vi "WVDIAL+HSRL_v4.0.vi"() -> ()   [LabVIEW 2012]
uses:
  C:/Users/H2ODial/Desktop/Shared Telescope WV DIAL Code/Libraries and VIs/PowerMeterCommands.dll
  Shared Telescope WV DIAL Code/Libraries and VIs/PowerMeterCommands.dll
  <vilib>/DAQmx/write.llb/DAQmx Write (Digital 1D Bool NChan 1Samp 1Line).vi
  <vilib>/DAQmx/miscellaneous.llb/DAQmx Fill In Error Info.vi
  <vilib>/Analysis/baseanly.llb/Mean (DBL).vi
  AMCS_Data.vi
  Libraries and VIs/Scalar_Data.vi
  <vilib>/Analysis/NI_AALBase.lvlib
  Libraries and VIs/Scalar_Data_2.vi
  Libraries and VIs/Scalar_Data_4.vi
  Libraries and VIs/Scalar_Data_3.vi
  Shared Telescope WV DIAL Code/bristol/CLDevIFace.dll
panel:
  out "FileHour":i32=20
  out "L_Count":i32=43
  out "background start":u32=534
  in  "Tab Control 2":enum32{"WV ND narrow", "WV ND wide"}(tab)=enum."WV ND wide"
  out "CH3 RingBuffer long":dbl[][](array[numeric])
  out "CH3 RingBuffer short":dbl[][](array[numeric])
  in  "?":T1(tab)=enum."Raw Counts combined"
  out "NRB":dbl[][](graph) caption="Water Vapor Number Density"
  out "NRB 2":dbl[][](graph)=[[-2.5020981634886346e-06, -3.8273570593616536e-05, -0.0001038319411503206, -0.00016406881143786204, -0.00024572601577053764, -0.00034001735639440826, -0.0003495277310288337, -0.00033797799127632697, -2.508089447238247e-05, 0.0004628603911393724, 0.0008910726426874336, 0.0014015403952404464, 0.0014313599056918725, 0.0023638962541973306, 0.00363462235094875, 0.005273167971630326, 0.007177084059402028, 0.007921603484325369, 0.010612501535131786, 0.013715391450269933, 0.01773512062835457, 0.025311202683991355, 0.029501238164518568, 0.03663684456864366, 0.042833095042680805, 0.04585338221968253, 0.05157986876646168, 0.057672169500993145, 0.06480582531005098, 0.07494068068754126, 0.08374302915097871, 0.09012600975592831, 0.0975137618371565, 0.10316252486978073, 0.10713266491787977, 0.11105920366892658, 0.11731957195587771, 0.12190536182534215, 0.13263667129454806, 0.14291236842912694, 0.15648209640166563, 0.17000563027429774, 0.1781337441537761, 0.18845836788040057, 0.18774352015967605, 0.1846468106536388, 0.18853627471102877, 0.18467849065439743, 0.19086511631707134, 0.2040589251100288, 0.207911100976431, 0.2171413823506752, 0.22141130681510074, 0.21910574498821542, 0.22451361076955265, 0.23126120500572805, 0.2339651115949773, 0.23260695324025257, 0.2442695368570803, 0.24254083915478225, 0.24350501849934109, 0.25495583092371427, 0.256919203446593, 0.2588364738795642, 0.2752215466716228, 0.2780859354051604, 0.276346005548185, 0.2745175766787534, 0.2601535580068366, 0.2676645740334584, 0.28421418272066157, 0.3206297444553061, 0.7143078116413505, 21.54115268912089, 33.95125947144662, 31.700981872059664, 41.68522002923662, 49.68783445276399, 45.33320709409449, 50.91175336548996, 41.008304913663714, 7.850979651089744, 0.6303614668230137, 0.015684134239805404, -0.10748397859242446, -0.14387707768036828, -0.16031827295901913, -0.18772557122864725, -0.18330253680007566, -0.18786123473446648, -0.19225778267096172, -0.1708619433096678, -0.18061455888020886, -0.20344725887325812, -0.21222191618851236, -0.2230615330389505, -0.22863568943154486, -0.21415229293082613, -0.19801980569945724, -0.17746233563109473, -0.17232152452285898, -0.19301319899423522, -0.1928522325449715, -0.20695955144125755, -0.2198018954874654, -0.20891051933015198, -0.2450116286469604, -0.2762364146721713, -0.25775858469018326, -0.2869767975303511, -0.31227413136513704, -0.30464323595703785, -0.3409117288411666, -0.3002103543236415, -0.23741414224173096, -0.26319432381274527, -0.23706217272299082, -0.28542556132066793, -0.3145034821484638, -0.27746295249821534, -0.2910899621994402, -0.22821160056074022, -0.2453504388340374, -0.2668569865375988, -0.302726932626319, -0.36635809732218244, -0.31647236719541494, -0.3452309484397592, -0.3275452371280285, -0.3333382932273667, -0.33548626372238755, -0.25688129406848426, -0.2467778023481867, -0.23498727603876554, -0.3129911904091031, -0.36614944944121386, -0.3533463690282559, -0.34154994204384004, -0.25165828962384623, -0.31691690943776746, -0.3245958208612461, -0.30425963660235494, -0.36843072902715324, -0.3157345000339491, -0.3275597079763837, -0.35818288327065395, -0.352364263091795, -0.33006433024904047, -0.3112468058790122, -0.23728059325129242, -0.22160963498338146, -0.22843717220060503, -0.31911234637289393, -0.43330862371719997, -0.45699042470294016, -0.4997768306732525, -0.4433418654318298, -0.44943541181506524, -0.482701240492616, -0.45281165642757787, -0.4539575719756435, -0.44359959762718015, -0.394802905964343, -0.43110696608508436, -0.4487943579107743, -0.44914927650382974, -0.4947334937868066, -0.5341525316404566, -0.45103820079960005, -0.4235942576800866, -0.42969521521255355, -0.3104652257561939, -0.3955757538174749, -0.3907148860769188, -0.3413445405384114, -0.44499503326768464, -0.4321269376895156, -0.46081506960875707, -0.4251383509343469, -0.41557002793056597, -0.40480981179417447, -0.34227620645148243, -0.2837964365676406, -0.2403409864667895, -0.31151461583845225, -0.40458731751210936, -0.4530771605846155, -0.530890834134058, -0.5174474687334719, -0.4705780895443756, -0.6251390473827461, -0.5608002128241332, -0.4805744396213767, -0.4939558392940799, -0.49893090586369987, -0.5815126113425622, -0.7539013482542295, -0.7201830577508319, -0.5974136122426202, -0.427319227255229, -0.23109328371912188, -0.37265592068247794, -0.4846088601881629, -0.5593198327797039, -0.6475257233138102, -0.6087540942922537, -0.4874376718973655, -0.47865733754219053, -0.5401916562010755, -0.596485197542672, -0.5963785290973199, -0.5983461777031588, -0.44328861700080574, -0.26085296759952376, -0.2699562750294853, -0.34464975700012546, -0.378374175405242, -0.509164782406029, -0.49723438050335145, -0.55406973131386, -0.5550984406698001, -0.43996054512749955, -0.5206803647051025, -0.4095467324146769, -0.48370538312072786, -0.5692902449808945, -0.6330050873588459, -0.8193325502186768, -0.8779549530887577, -0.816539854359666, -0.6441653120171549, -0.4727360575130327, -0.4628552538239389, -0.5620478433524031, -0.655494042494383, -0.7399613369892488, -0.6405030408770369, -0.5765708949382735, -0.4726984725137904, -0.3915113429195965, -0.3134944364340016, -0.2248912333800384, -0.36875022215993414, -0.3554536886236827, -0.5980166385656092, -0.8193537790579545, -0.7521812952169191, -0.6971205141068005, -0.6181283857949139, -0.5900935588544917, -0.7562170181152746, -0.6416065082367906, -0.7307816848017402, -0.5270352944590446, -0.300116480279226, -0.37553963593937656, -0.2941933059065934, -0.47641380968548086, -0.5378654657741927, -0.6071779010544753, -0.4686312128566513, -0.5899512920252556, -0.6862698061644342, -0.7428879117678355, -0.8761602999416397, -0.7561276317699211, -0.7202615010974514, -0.7483281485207611, -0.7482154522350888, -0.5525177903179376, -0.4488008176595967, -0.22978861391703273, -0.13150232773217932, -0.1332402387625776, -0.06078266202039725, -0.39966517834005755, -0.5783801042920869, -0.8171422439228425, -0.9551656614336947, -0.8733043067019355, -0.6959516078841153, -0.7690989054771367, -0.8652022149225229, -0.6099182034625025, -0.7679998738959176, -0.7223416094461833, -0.7570644057546929, -1.2654974200164584, -1.3779590792235303, -1.5622266280255943, -1.386936070753788, -1.2471038836252353, -1.087283687193855, -0.8721120158881883, -1.0872571189847513, -0.9849759903134073, -0.771411546098274, -0.8509297898990206, -0.9081599500982982, -0.6790337607839299, -0.9278070419202001, -0.621797181323692, -0.5821482738615157, -1.0750661807231106, -1.2314382214462831, -1.5519022989390405, -1.4796651905938325, -1.2102421860882273, -1.0282077259873421, -0.4362873109031171, -0.40559426367495305, -0.2292032463648166, -0.21857441066377944, -0.9109430342662433, -1.282550258698898, -1.3876047401862814, -1.5045893419592666, -1.4374711281318844, -1.2050621952116298, -1.0103568077270157, -0.5897468684843571, -0.29535566057607804, -0.27893832184515194, -0.6263885355424194, -0.9074170726475529, -0.9534692140938759, -0.9710631908445434, -0.760777904963038, -0.8433895851549431, -0.7917487575180413, -0.7514584846094501, -0.8766094127754804, -0.671180633107386, -0.5887340833307931, -0.6049688202388804, -0.6515728951252249, -0.7953097338321125, -0.9273888663025621, -0.6352708304436501, -0.7532266459861103, -0.953097474788277, -1.014056313184273, -1.2798394152447108, -1.2552531089492367, -1.3478709811287533, -1.4390342075966889, -1.426306262141701, -1.381381316355439, -0.9252331614157784, -0.41493739744643776, -0.3243230693658629, -0.06387449281903544, -0.18609024214117245, -0.7804262391658887, -1.0493895157641866, -1.3174091629330624, -1.3903818994181472, -1.152477696612482, -1.0616779068473232, -0.9080173908622341, -0.8545100052333319, -0.47579763315226625, -0.08556205823523852, -0.22014402145078743, -0.10890642998361617, -0.5553035660570823, -0.2958777336933946, -0.3959921627809348, -0.556970419169587, -0.4186254510131068, -0.7485884874552019, -0.19289238765646766, 0.05430929448269791, -0.35478245323789875, -1.0561668550116012, -1.1898220201473728, -1.2458813203298933, -0.815334398103235, -0.0671490954357261, -0.018451762627068893, -0.11119254378964742, -0.4427154390499537, -0.6760221931822215, -1.3461845836896529, -1.8076463186027565, -1.8385077103062597, -1.7869301307658811, -1.6232306012680962, -1.4738471688873729, -1.3087672612167474, -1.2315906623490736, -1.1135123530760682, -1.139861483958716, -1.2569515292132314, -1.4088959931515883, -1.1250574891186882, -1.001539558123051, -0.7088183927720361, -0.514128544452265, -0.3454411632455565, 0.3000404281767336, 0.1645627582469719, 0.04890717768161907, 0.08947454524138758, -0.07724098944459341, -0.058958284211915034, -0.3667306904105761, -0.9904304551610316, -1.7027285480575052, -1.306338059968992, -1.1597564928464528, -0.3530837286192967, 0.5746539364824368, 0.23334933859722826, 0.4182851174867973, -0.30059774866289063, -0.8890626237655932, -0.9472750803671779, -0.8578628063534488, -0.9533360290473383, -0.5079315412639782, -0.26717148091086973, -0.45138122167384986, -0.8642746108786942, -0.7295568974321442, -0.6794525679270975, -0.4380641006827398, 0.5769193464805378, 0.22719774605138796, -0.2983324510443344, -0.30673253473033524, -0.8094870539813328, -1.035132568856701, -0.4124781117273112, -0.2747964251818897, -0.11039052863799699, -0.5885488301511802, -0.8058036703841541, -0.4663379722359256, -0.33030440722377336, -0.467927769570105, -1.1000558593661727, -2.0467207202621625, -2.551496069836077, -2.0536979920090666, -1.3499994517878882, -1.153871773838675, -0.5889425800789698, -0.2969193437698364, -0.37189047692613214, -0.09857520941841777, -0.892482435033178, -0.3015291458282375, -0.4266194375179333, -0.1408214342371235, 0.16821762837943968, -0.40361403530403833, -0.7177182682819262, -1.0728370530752864, -1.3729370161062138, -1.357043316659708, -1.0180794658931187, -1.3953152006681284, -0.7536344811984687, -0.5284048490717401, -0.4122172561441862, -0.054807712791502865, 0.5146587876030838, 0.4753438773876348, 0.3674548243403802, -0.7042427610448878, -1.1016058965545648, -0.9988289529332682, -1.6435072651641673, -0.6465888479397265, -0.7806826027457424, -1.022038241655911, -0.230679192242146, -0.759068236712521, -0.7535460754503612, -1.7178022862235443, -1.5663725973853304, -0.7565920024141967, -1.0450226922537755, -0.5586958948537327, -0.5488466781858061, -0.5568035653235451, -1.1032149253845942, -0.8009372538073485, -0.34126394357978, -0.8844203222099551, -0.6006849348938932, -0.6731739721978937, -1.460340765246951, -1.4452465918657313, -0.26441783208271397, -0.4943103053231315, -0.14316728933687042, 0.47572218129688315, -0.40079671920864024, -0.5505246695459326, -0.7083516606019646, -0.03233006932487573, -0.512690199641294, 0.26494490817366023, -0.7759032781550804, -1.578772092440307, -0.09584587307128617, 0.45052636975528176, 0.49960481452995287, 0.13866569826607072, -1.756634496879691, -3.626331301345096, -2.473565538083194, -2.245781662386054, -1.8764305761241498, -0.45052407312514464, -0.752383991024165, -0.758988271335676, 0.176068333208736, -0.1380694180006847, -0.06847766192829471, -0.37563895911621303, -0.9959950091463621, -0.9345547358580696, -1.2513440806923193, -0.41094699891746117, -0.2097207952913438, -1.4365356108808607, -0.7837923842133756, -0.3968929772583404, -1.0140166859071411, -0.9038007040018414, -0.7252283164133516, -1.5910573858643522, -0.25161165903524585, 0.3124499929369491, -0.7977022908808816, -0.9890490078668146, -1.1747915260490664, -1.0295378767351495, 0.45640125561722844, 1.0024654779812845, 0.6740581377789816, 1.033309351341288, 0.6186635225683902, -0.30003043189290396, 0.20275337833113002, 0.49308937811843856, 0.1813997653039158, 0.22789885511426033, 0.8665664819010523, 0.24739566365173932, 0.6284997182377698, 1.6889726435607322, 0.0, 0.0, 0.0, 0.0, 0.0]] caption="Water Vapor Number Density"
  out "CH 1 (WV off) counts display":dbl[][](graph) caption="Water Vapor Number Density"
  out "CH 3 (HSRL comb) counts display":dbl[][](graph)=[[163.47999999999956, -42.52000000000044, 147.47999999999956, 56.47999999999956, 162.47999999999956, -112.52000000000044, 181.47999999999956, 69.47999999999956, 61.47999999999956, -109.52000000000044, 99.47999999999956, 24.479999999999563, 29.479999999999563, -9.520000000000437, 82.47999999999956, 93.47999999999956, 110.47999999999956, -50.52000000000044, 22.479999999999563, -20.520000000000437, -58.52000000000044, 64.47999999999956, 110.47999999999956, 140.47999999999956, 300.47999999999956, 243.47999999999956, 153.47999999999956, 253.47999999999956, 165.47999999999956, 274.47999999999956, 247.47999999999956, 380.47999999999956, 156.47999999999956, 346.47999999999956, 248.47999999999956, 285.47999999999956, 327.47999999999956, 353.47999999999956, 258.47999999999956, 140.47999999999956, 243.47999999999956, 243.47999999999956, 229.47999999999956, 238.47999999999956, 279.47999999999956, 188.47999999999956, 327.47999999999956, 293.47999999999956, 292.47999999999956, 291.47999999999956, 196.47999999999956, 333.47999999999956, 129.47999999999956, 72.47999999999956, 119.47999999999956, 267.47999999999956, 205.47999999999956, 135.47999999999956, 305.47999999999956, 111.47999999999956, 145.47999999999956, 190.47999999999956, 271.47999999999956, 144.47999999999956, 133.47999999999956, 230.47999999999956, 162.47999999999956, 201.47999999999956, 195.47999999999956, 277.47999999999956, 258.47999999999956, 80.47999999999956, 44.47999999999956, 160.47999999999956, 347.47999999999956, 882.4799999999996, 31366.48, 56924.479999999996, -5504.52, 57991.479999999996, 42322.479999999996, 13697.48, 1435.4799999999996, 48.47999999999956, -40.52000000000044, -63.52000000000044, 22.479999999999563, -217.52000000000044, 91.47999999999956, -239.52000000000044, -60.52000000000044, -95.52000000000044, 6.479999999999563, -24.520000000000437, -143.52000000000044, -131.52000000000044, 25.479999999999563, -192.52000000000044, 31.479999999999563, -141.52000000000044, 71.47999999999956, -31.520000000000437, -63.52000000000044, -57.52000000000044, -23.520000000000437, -109.52000000000044, -10.520000000000437, 4.479999999999563, -42.52000000000044, -61.52000000000044, -92.52000000000044, -39.52000000000044, -46.52000000000044, 124.47999999999956, -113.52000000000044, 28.479999999999563, 55.47999999999956, -83.52000000000044, -197.52000000000044, 48.47999999999956, -50.52000000000044, -60.52000000000044, -104.52000000000044, -64.52000000000044, -26.520000000000437, -72.52000000000044, 34.47999999999956, 85.47999999999956, -56.52000000000044, -177.52000000000044, -104.52000000000044, -89.52000000000044, -140.52000000000044, -46.52000000000044, 0.47999999999956344, -11.520000000000437, -73.52000000000044, 29.479999999999563, -94.52000000000044, -59.52000000000044, -53.52000000000044, 38.47999999999956, -137.52000000000044, 57.47999999999956, 3.4799999999995634, -143.52000000000044, -10.520000000000437, 69.47999999999956, -167.52000000000044, -3.5200000000004366, 62.47999999999956, 6.479999999999563, 5.479999999999563, -83.52000000000044, -31.520000000000437, -159.52000000000044, -85.52000000000044, -72.52000000000044, -163.52000000000044, -137.52000000000044, -108.52000000000044, -30.520000000000437, 86.47999999999956, -37.52000000000044, 50.47999999999956, -66.52000000000044, 115.47999999999956, 45.47999999999956, 150.47999999999956, -129.52000000000044, -45.52000000000044, 28.479999999999563, -82.52000000000044, -160.52000000000044, -107.52000000000044, 59.47999999999956, -273.52000000000044, -3.5200000000004366, -25.520000000000437, -28.520000000000437, -9.520000000000437, -21.520000000000437, -111.52000000000044, 3.4799999999995634, -113.52000000000044, -100.52000000000044, 5.479999999999563, -9.520000000000437, 19.479999999999563, 59.47999999999956, -135.52000000000044, 83.47999999999956, 0.47999999999956344, -2.5200000000004366, -197.52000000000044, -24.520000000000437, 15.479999999999563, 2.4799999999995634, -176.52000000000044, -151.52000000000044, 113.47999999999956, 0.47999999999956344, 49.47999999999956, 115.47999999999956, -214.52000000000044, -17.520000000000437, 15.479999999999563, -41.52000000000044, 43.47999999999956, -36.52000000000044, -52.52000000000044, -157.52000000000044, -244.52000000000044, -63.52000000000044, 72.47999999999956, 90.47999999999956, 43.47999999999956, -9.520000000000437, 20.479999999999563, 145.47999999999956, -57.52000000000044, -139.52000000000044, 59.47999999999956, 51.47999999999956, -102.52000000000044, -199.52000000000044, -21.520000000000437, 111.47999999999956, -76.52000000000044, 54.47999999999956, -28.520000000000437, 8.479999999999563, 32.47999999999956, -121.52000000000044, -142.52000000000044, -106.52000000000044, 21.479999999999563, -22.520000000000437, 44.47999999999956, 43.47999999999956, -155.52000000000044, 64.47999999999956, 140.47999999999956, -107.52000000000044, -2.5200000000004366, 71.47999999999956, -17.520000000000437, -33.52000000000044, -85.52000000000044, 121.47999999999956, -191.52000000000044, 114.47999999999956, 2.4799999999995634, 24.479999999999563, 143.47999999999956, -107.52000000000044, 107.47999999999956, -2.5200000000004366, 31.479999999999563, -55.52000000000044, -102.52000000000044, -0.5200000000004366, -93.52000000000044, -209.52000000000044, 110.47999999999956, -50.52000000000044, 36.47999999999956, -52.52000000000044, 88.47999999999956, 22.479999999999563, -84.52000000000044, 52.47999999999956, 105.47999999999956, -94.52000000000044, 3.4799999999995634, -114.52000000000044, 108.47999999999956, -101.52000000000044, -3.5200000000004366, 86.47999999999956, -96.52000000000044, -42.52000000000044, -116.52000000000044, 90.47999999999956, 47.47999999999956, -26.520000000000437, -97.52000000000044, -161.52000000000044, 34.47999999999956, -30.520000000000437, 54.47999999999956, -117.52000000000044, -85.52000000000044, 46.47999999999956, 69.47999999999956, -1.5200000000004366, 135.47999999999956, 49.47999999999956, 4.479999999999563, 71.47999999999956, -11.520000000000437, -89.52000000000044, 83.47999999999956, -77.52000000000044, -74.52000000000044, -125.52000000000044, -176.52000000000044, -90.52000000000044, -0.5200000000004366, -148.52000000000044, 26.479999999999563, -34.52000000000044, -106.52000000000044, 97.47999999999956, 62.47999999999956, -68.52000000000044, 103.47999999999956, 68.47999999999956, 44.47999999999956, -1.5200000000004366, -112.52000000000044, 8.479999999999563, -159.52000000000044, 34.47999999999956, 34.47999999999956, -59.52000000000044, -89.52000000000044, -55.52000000000044, -82.52000000000044, 1.4799999999995634, -21.520000000000437, 13.479999999999563, 65.47999999999956, 154.47999999999956, -1.5200000000004366, -56.52000000000044, -3.5200000000004366, 89.47999999999956, 26.479999999999563, -15.520000000000437, 14.479999999999563, -28.520000000000437, -17.520000000000437, 38.47999999999956, -207.52000000000044, 30.479999999999563, -2.5200000000004366, 19.479999999999563, -59.52000000000044, 17.479999999999563, 3.4799999999995634, -23.520000000000437, 9.479999999999563, 178.47999999999956, 111.47999999999956, -89.52000000000044, -157.52000000000044, -84.52000000000044, -6.520000000000437, 80.47999999999956, 139.47999999999956, 15.479999999999563, -79.52000000000044, -157.52000000000044, 117.47999999999956, 12.479999999999563, -65.52000000000044, -15.520000000000437, -123.52000000000044, -44.52000000000044, 34.47999999999956, 2.4799999999995634, -118.52000000000044, -15.520000000000437, 34.47999999999956, 4.479999999999563, -17.520000000000437, -46.52000000000044, 103.47999999999956, 33.47999999999956, -6.520000000000437, 5.479999999999563, 94.47999999999956, -185.52000000000044, -14.520000000000437, -142.52000000000044, -40.52000000000044, -82.52000000000044, -8.520000000000437, -96.52000000000044, -58.52000000000044, -18.520000000000437, 35.47999999999956, 42.47999999999956, -8.520000000000437, 102.47999999999956, 159.47999999999956, 29.479999999999563, 131.47999999999956, 20.479999999999563, -62.52000000000044, -42.52000000000044, 99.47999999999956, 48.47999999999956, -1.5200000000004366, 35.47999999999956, -32.52000000000044, 128.47999999999956, -8.520000000000437, -83.52000000000044, 55.47999999999956, -1.5200000000004366, -92.52000000000044, 58.47999999999956, 23.479999999999563, 101.47999999999956, 63.47999999999956, -2.5200000000004366, 151.47999999999956, 6.479999999999563, 47.47999999999956, 44.47999999999956, -96.52000000000044, 79.47999999999956, -147.52000000000044, 25.479999999999563, -124.52000000000044, 77.47999999999956, 63.47999999999956, -5.520000000000437, 27.479999999999563, -142.52000000000044, -36.52000000000044, -58.52000000000044, -98.52000000000044, -83.52000000000044, 21.479999999999563, -7.520000000000437, -51.52000000000044, -123.52000000000044, 5.479999999999563, 69.47999999999956, -55.52000000000044, -79.52000000000044, 68.47999999999956, -40.52000000000044, -54.52000000000044, 28.479999999999563, -50.52000000000044, 64.47999999999956, -87.52000000000044, 104.47999999999956, 48.47999999999956, 44.47999999999956, -165.52000000000044, 87.47999999999956, -116.52000000000044, 5.479999999999563, -68.52000000000044, 44.47999999999956, 180.47999999999956, 175.47999999999956, 117.47999999999956, -28.520000000000437, 74.47999999999956, 83.47999999999956, 95.47999999999956, 121.47999999999956, 67.47999999999956, 15.479999999999563, 74.47999999999956, -1.5200000000004366, 2.4799999999995634, -21.520000000000437, -232.52000000000044, 83.47999999999956, -96.52000000000044, 8.479999999999563, -115.52000000000044, -87.52000000000044, 4.479999999999563, 20.479999999999563, 67.47999999999956, -180.52000000000044, 8.479999999999563, -62.52000000000044, -75.52000000000044, -18.520000000000437, -116.52000000000044, 61.47999999999956, -23.520000000000437, 79.47999999999956, 112.47999999999956, -79.52000000000044, -41.52000000000044, -162.52000000000044, 22.479999999999563, -24.520000000000437, -2.5200000000004366, -26.520000000000437, 71.47999999999956, 4.479999999999563, 4.479999999999563, -99.52000000000044, 84.47999999999956, -61.52000000000044, 33.47999999999956, -67.52000000000044, -71.52000000000044, 43.47999999999956, -15.520000000000437, -79.52000000000044, -63.52000000000044, -3.5200000000004366, -43.52000000000044, -105.52000000000044, -6.520000000000437, -38.52000000000044, -38.52000000000044, 16.479999999999563, 129.47999999999956, -28.520000000000437, 16.479999999999563, -50.52000000000044, 132.47999999999956, -76.52000000000044, 34.47999999999956, 47.47999999999956, -135.52000000000044, -27.520000000000437, 43.47999999999956, -111.52000000000044, 79.47999999999956, 74.47999999999956, -33.52000000000044, -53.52000000000044, 28.479999999999563, -17.520000000000437, 83.47999999999956, -30.520000000000437, -17.520000000000437, 13.479999999999563, 10.479999999999563, -45.52000000000044, 54.47999999999956, 165.47999999999956, -3.5200000000004366, -40.52000000000044, -41.52000000000044, -2.5200000000004366, -18.520000000000437, 44.47999999999956, -45.52000000000044, -103.52000000000044, 84.47999999999956, -46.52000000000044, 1.4799999999995634, 16.479999999999563, -2.5200000000004366, 0.0]] caption="Water Vapor Number Density"
  out "CH3 (HSRL combined) smooth S":dbl[](array[numeric])=[-5.880967741935467, -22.493870967741916, -27.122903225806432, -24.10677419354837, -23.10677419354837, -22.203548387096756, -16.768064516129016, -12.413225806451594, -0.7277419354838548, 10.877096774193564, 17.304516129032276, 22.869032258064532, 19.901290322580664, 28.336774193548404, 37.949677419354856, 48.3851612903226, 58.328709677419376, 57.42548387096776, 69.03838709677422, 80.51419354838711, 94.41741935483871, 122.74000000000001, 130.87709677419355, 149.24, 160.7803225806452, 159.1351612903226, 165.98193548387098, 172.55451612903227, 180.74, 195.27225806451614, 204.33677419354842, 206.37709677419357, 209.95774193548388, 209.24806451612903, 205.07064516129034, 200.94967741935486, 200.95774193548388, 197.97387096774196, 204.48193548387098, 209.43354838709678, 218.24806451612906, 225.9335483870968, 225.85290322580647, 228.19967741935488, 217.36903225806455, 204.61903225806455, 200.14322580645162, 187.99, 186.44161290322583, 191.42548387096775, 187.47387096774196, 188.3367741935484, 184.86903225806452, 176.24806451612903, 174.09483870967745, 172.98193548387098, 168.92548387096775, 162.21580645161293, 164.61903225806452, 158.06258064516132, 153.53838709677422, 155.6109677419355, 151.87709677419355, 148.27225806451617, 152.8367741935484, 149.78838709677422, 144.44967741935486, 139.3125806451613, 128.24, 128.19967741935486, 132.3125806451613, 145.12709677419355, 313.9254838709678, 8378.159354838708, 12241.586774193547, 11271.489999999998, 13944.506129032256, 15799.47387096774, 14332.546451612903, 15460.320645161291, 12615.24806451613, 2662.3851612903227, 214.5383870967742, 5.22387096774195, -34.977741935483856, -45.74387096774191, -49.808387096774176, -57.009999999999984, -54.42129032258063, -54.54225806451611, -54.598709677419336, -47.469677419354824, -49.106774193548375, -54.147096774193535, -55.300322580645144, -56.92129032258063, -57.14709677419353, -52.437419354838696, -47.50999999999999, -41.72774193548386, -39.719677419354824, -43.62290322580643, -42.74387096774192, -44.99387096774192, -46.880967741935464, -43.719677419354824, -50.32451612903225, -55.69548387096773, -51.018064516129016, -55.77612903225805, -59.606774193548375, -57.1148387096774, -62.79225806451611, -54.32451612903224, -42.211612903225785, -45.99387096774191, -40.719677419354824, -48.20354838709676, -52.227741935483856, -45.308387096774176, -46.75193548387095, -36.050322580645144, -38.130967741935464, -40.808387096774176, -45.558387096774176, -54.268064516129016, -46.139032258064496, -49.550322580645144, -46.28419354838709, -46.380967741935464, -45.96967741935482, -34.66322580645159, -32.800322580645144, -30.768064516129016, -40.380967741935464, -46.550322580645144, -44.268064516129016, -42.171290322580624, -30.622903225806432, -38.018064516129016, -38.389032258064496, -35.47774193548385, -42.3648387096774, -35.800322580645144, -36.63096774193547, -39.509999999999984, -38.34064516129031, -35.42935483870966, -32.96161290322579, -24.792258064516115, -22.848709677419336, -23.24387096774192, -32.050322580645144, -42.96161290322579, -44.727741935483856, -48.29225806451611, -42.29225806451611, -42.33258064516127, -44.89709677419353, -41.590645161290304, -41.179354838709656, -39.74387096774192, -34.937419354838696, -37.687419354838696, -38.759999999999984, -38.32451612903223, -41.711612903225785, -44.50193548387095, -37.130967741935464, -34.46161290322579, -34.550322580645144, -24.671290322580628, -31.07451612903224, -30.340645161290304, -26.20354838709676, -33.77612903225805, -32.42935483870966, -34.19548387096772, -31.195483870967728, -30.155161290322567, -29.050322580645144, -24.292258064516112, -19.921290322580628, -16.687419354838696, -21.397096774193532, -27.49387096774192, -30.46161290322579, -35.31645161290321, -34.058387096774176, -30.647096774193535, -40.29225806451611, -35.768064516129016, -30.332580645161272, -30.856774193548368, -30.848709677419336, -35.590645161290304, -45.679354838709656, -43.19548387096772, -35.469677419354824, -25.114838709677404, -13.445483870967724, -21.469677419354824, -27.647096774193532, -31.59870967741934, -36.227741935483856, -33.727741935483856, -26.74387096774192, -26.009999999999984, -29.07451612903224, -31.800322580645144, -31.49387096774192, -31.300322580645147, -22.969677419354824, -13.3890322580645, -13.727741935483854, -17.364838709677404, -18.8890322580645, -25.187419354838696, -24.372903225806436, -26.913225806451596, -26.71967741935482, -20.985806451612888, -24.614838709677404, -19.187419354838692, -22.46161290322579, -26.20354838709676, -28.88096774193547, -37.05838709677418, -39.3648387096774, -36.29225806451612, -28.380967741935468, -20.647096774193532, -20.042258064516112, -24.130967741935468, -27.905161290322564, -31.235806451612888, -26.808387096774176, -23.929354838709664, -19.453548387096756, -15.977741935483856, -12.687419354838694, -9.026129032258048, -14.679354838709662, -14.03419354838708, -23.421290322580628, -31.832580645161276, -28.985806451612888, -26.647096774193535, -23.437419354838696, -22.195483870967728, -28.219677419354824, -23.75193548387095, -26.840645161290304, -19.20354838709676, -10.848709677419336, -13.46967741935482, -10.469677419354822, -16.82451612903224, -18.848709677419336, -21.1148387096774, -16.171290322580628, -20.20354838709676, -23.32451612903224, -25.058387096774176, -29.332580645161272, -25.122903225806432, -23.751935483870948, -24.49387096774192, -24.30838709677418, -17.816451612903208, -14.364838709677404, -7.300322580645146, -4.147096774193532, -4.171290322580629, -1.8890322580644998, -12.332580645161274, -17.719677419354824, -24.856774193548368, -28.848709677419333, -26.187419354838692, -20.719677419354824, -22.735806451612888, -25.397096774193532, -17.776129032258048, -22.227741935483856, -20.759999999999984, -21.606774193548368, -35.87290322580644, -38.79225806451611, -43.67935483870966, -38.509999999999984, -34.3890322580645, -29.776129032258048, -23.719677419354824, -29.372903225806436, -26.429354838709664, -20.558387096774176, -22.526129032258048, -23.880967741935468, -17.735806451612888, -24.074516129032244, -16.026129032258048, -14.905161290322564, -27.34870967741934, -31.122903225806436, -38.969677419354824, -36.91322580645159, -29.99387096774192, -25.316451612903208, -10.671290322580628, -9.856774193548372, -5.53419354838708, -5.24387096774192, -21.719677419354824, -30.389032258064503, -32.67129032258063, -35.20354838709676, -33.42129032258063, -27.840645161290308, -23.195483870967728, -13.453548387096758, -6.695483870967726, -6.284193548387081, -14.026129032258048, -20.195483870967728, -21.090645161290308, -21.34870967741934, -16.622903225806436, -18.316451612903208, -17.090645161290308, -16.122903225806436, -18.695483870967728, -14.227741935483854, -12.405161290322564, -12.671290322580628, -13.566451612903208, -16.46161290322579, -19.082580645161276, -12.993870967741918, -15.31645161290321, -19.268064516129016, -20.380967741935468, -25.574516129032244, -24.937419354838692, -26.622903225806436, -28.259999999999984, -27.84870967741934, -26.81645161290321, -17.85677419354837, -7.96161290322579, -6.187419354838694, -1.2116129032257903, -3.509999999999984, -14.6390322580645, -19.57451612903224, -24.437419354838692, -25.64709677419353, -21.139032258064496, -19.364838709677404, -16.469677419354824, -15.413225806451596, -8.534193548387082, -1.5261290322580485, -3.9051612903225643, -1.9212903225806286, -9.74387096774192, -5.163225806451596, -6.872903225806435, -9.614838709677404, -7.187419354838693, -12.78419354838708, -3.2761290322580474, 0.9174193548387262, -5.96161290322579, -17.655161290322564, -19.78419354838708, -20.60677419354837, -13.413225806451596, -1.0987096774193386, -0.30032258064514505, -1.800322580645145, -7.130967741935468, -10.832580645161274, -21.46161290322579, -28.67129032258063, -29.009999999999984, -28.050322580645144, -25.34870967741934, -22.897096774193532, -20.227741935483852, -18.937419354838696, -17.03419354838708, -17.348709677419336, -19.03419354838708, -21.227741935483856, -16.864838709677404, -14.937419354838694, -10.518064516129016, -7.590645161290306, -5.074516129032242, 4.385161290322596, 2.393225806451629, 0.7077419354838868, 1.2883870967742097, -1.106774193548371, -0.8406451612903063, -5.203548387096758, -13.985806451612886, -23.92935483870966, -18.268064516129016, -16.1390322580645, -4.8890322580645, 7.917419354838726, 3.199677419354855, 5.707741935483886, -4.082580645161274, -12.018064516129016, -12.74387096774192, -11.485806451612888, -12.703548387096758, -6.735806451612888, -3.526129032258048, -5.929354838709662, -11.300322580645144, -9.49387096774192, -8.800322580645144, -5.647096774193531, 7.401290322580662, 2.901290322580661, -3.7922580645161132, -3.880967741935468, -10.195483870967726, -12.977741935483856, -5.147096774193532, -3.413225806451597, -1.364838709677403, -7.24387096774192, -9.872903225806436, -5.687419354838695, -4.009999999999985, -5.655161290322565, -13.235806451612888, -24.518064516129016, -30.42935483870966, -24.380967741935468, -15.953548387096758, -13.574516129032244, -6.897096774193531, -3.46161290322579, -4.31645161290321, -1.1390322580644998, -10.268064516129016, -3.453548387096758, -4.864838709677404, -1.5987096774193392, 1.9012903225806612, -4.542258064516112, -8.042258064516112, -11.969677419354822, -15.251935483870952, -15.009999999999982, -11.21161290322579, -15.300322580645144, -8.227741935483856, -5.743870967741919, -4.46161290322579, -0.5906451612903062, 5.522258064516146, 5.078709677419371, 3.9093548387096946, -7.46161290322579, -11.622903225806436, -10.49387096774192, -17.195483870967728, -6.735806451612886, -8.098709677419338, -10.558387096774178, -2.3729032258064353, -7.776129032258048, -7.687419354838693, -17.45354838709676, -15.848709677419338, -7.622903225806435, -10.485806451612888, -5.582580645161274, -5.46161290322579, -5.518064516129016, -10.8890322580645, -7.872903225806435, -3.340645161290305, -8.622903225806436, -5.832580645161275, -6.509999999999985, -14.06645161290321, -13.864838709677404, -2.526129032258048, -4.703548387096758, -1.3567741935483704, 4.490000000000016, -3.768064516129016, -5.155161290322565, -6.606774193548371, -0.30032258064514394, -4.743870967741919, 2.441612903225823, -7.122903225806435, -14.437419354838692, -0.8729032258064358, 4.086774193548404, 4.514193548387114, 1.2480645161290491, -15.751935483870952, -32.397096774193535, -22.009999999999984, -19.905161290322564, -16.566451612903208, -3.9616129032257894, -6.590645161290306, -6.622903225806435, 1.5303225806451777, -1.1954838709677256, -0.5906451612903062, -3.2277419354838544, -8.526129032258048, -7.969677419354823, -10.630967741935468, -3.477741935483855, -1.7680645161290158, -12.066451612903208, -6.558387096774176, -3.3083870967741777, -8.421290322580628, -7.477741935483854, -5.977741935483854, -13.06645161290321, -2.0583870967741773, 2.5464516129032413, -6.477741935483854, -8.001935483870952, -9.469677419354822, -8.268064516129016, 3.651290322580661, 7.990000000000016, 5.352903225806468, 8.175483870967758, 4.877096774193565, -2.35677419354837, 1.586774193548404, 3.8448387096774366, 1.4093548387096946, 1.7641935483871132, 6.683548387096791, 1.9012903225806612, 4.812580645161307, 12.885161290322596]
  out "CH3 (HSRL combined) smooth L":dbl[](array[numeric])=[-17.463260869565204, -33.82195652173912, -32.468695652173906, -29.849130434782598, -27.300217391304336, -24.00673913043477, -20.300217391304336, -15.452391304347815, -3.789347826086945, 3.134565217391315, 8.21608695652175, 15.313913043478271, 17.096521739130445, 24.406304347826097, 37.22695652173914, 50.313913043478266, 59.91717391304349, 63.75413043478262, 72.37369565217392, 80.30847826086958, 89.92260869565219, 112.75413043478261, 125.13456521739131, 139.44434782608698, 152.9389130434783, 154.23782608695655, 163.46608695652174, 170.97695652173914, 180.7541304347826, 194.03130434782605, 194.91173913043477, 203.4008695652174, 201.88456521739133, 200.015, 202.22152173913045, 197.3519565217391, 198.8247826086956, 198.87913043478258, 204.13456521739133, 205.3030434782609, 210.59652173913045, 216.87369565217395, 213.50956521739135, 213.9389130434783, 207.96065217391305, 196.74869565217392, 191.24869565217392, 185.69434782608695, 182.81934782608695, 188.68347826086958, 187.17260869565217, 189.5041304347826, 186.8247826086956, 174.515, 171.55304347826086, 164.6726086956522, 160.5258695652174, 155.08565217391305, 159.10739130434783, 153.4008695652174, 150.3954347826087, 151.98782608695655, 149.48239130434786, 145.79217391304348, 144.72695652173914, 142.58021739130436, 132.5095652173913, 132.23782608695655, 124.54217391304348, 125.18891304347827, 128.18891304347827, 136.4389130434783, 302.9117391304348, 7948.79760869565, 12767.781304347824, 12528.460652173913, 15319.455217391303, 17737.069347826087, 15606.493260869567, 16072.585652173913, 13111.77586956522, 3011.84652173913, 276.5204347826086, -5.528478260869555, -48.359999999999985, -57.838260869565204, -55.430652173913025, -57.90347826086955, -52.80565217391303, -51.39804347826086, -56.0936956521739, -50.89804347826086, -50.62086956521738, -53.968695652173906, -56.54478260869564, -55.3545652173913, -55.37630434782608, -51.75130434782608, -49.76217391304347, -47.65891304347825, -48.2186956521739, -51.838260869565204, -49.446956521739125, -52.64804347826086, -50.53934782608694, -48.13717391304347, -51.98499999999999, -55.86543478260869, -56.13717391304347, -57.14260869565217, -60.05021739130434, -57.061086956521734, -60.05021739130433, -53.92521739130434, -44.631739130434774, -47.63717391304347, -43.81652173913043, -52.69152173913042, -58.506739130434774, -54.31108695652173, -53.88717391304347, -42.300217391304336, -38.69695652173912, -36.62630434782608, -41.050217391304336, -51.78391304347825, -47.57739130434781, -53.963260869565204, -52.15347826086956, -50.78391304347825, -48.38717391304347, -39.40891304347825, -36.8491304347826, -35.91978260869564, -44.04478260869564, -43.90891304347825, -41.66978260869564, -39.19152173913042, -32.94152173913042, -38.15891304347825, -43.70239130434781, -42.13717391304347, -47.653478260869555, -48.80021739130434, -45.68065217391303, -46.278478260869555, -47.506739130434774, -42.62630434782608, -39.903478260869555, -33.44152173913042, -29.876304347826075, -32.28391304347825, -39.00673913043477, -48.7078260869565, -49.609999999999985, -47.56652173913042, -43.91434782608694, -41.77847826086955, -43.300217391304336, -41.017608695652164, -38.52847826086955, -42.25673913043477, -34.892608695652164, -39.28391304347825, -38.11543478260868, -30.74586956521738, -37.78391304347825, -39.66978260869564, -39.349130434782595, -41.696956521739125, -38.963260869565204, -32.0936956521739, -36.414347826086946, -36.52304347826086, -34.82195652173912, -39.506739130434774, -34.446956521739125, -30.963260869565207, -27.88173913043477, -24.648043478260856, -22.648043478260856, -19.2186956521739, -15.751304347826075, -19.376304347826075, -24.713260869565204, -32.44695652173912, -36.31652173913042, -38.31652173913042, -39.45239130434781, -41.89260869565216, -50.33282608695651, -46.54478260869564, -43.582826086956516, -38.55565217391303, -37.39804347826086, -39.65891304347825, -45.53391304347825, -41.49043478260869, -37.55021739130433, -29.87086956521738, -22.39804347826086, -30.69695652173912, -34.94695652173912, -40.968695652173906, -46.131739130434774, -44.164347826086946, -35.31108695652173, -30.767608695652164, -27.44695652173912, -31.175217391304336, -33.3491304347826, -31.816521739130422, -28.33282608695651, -16.54478260869564, -15.354565217391293, -17.403478260869555, -18.51217391304347, -25.115434782608684, -22.53391304347825, -28.175217391304336, -27.946956521739118, -27.055652173913035, -30.273043478260856, -22.936086956521727, -24.36543478260868, -23.061086956521727, -26.54478260869564, -33.82739130434781, -38.93608695652173, -37.245869565217376, -32.10456521739129, -26.436086956521727, -22.23499999999999, -27.24586956521738, -27.838260869565204, -32.56108695652173, -27.452391304347813, -21.811086956521727, -22.006739130434774, -17.202391304347813, -16.15347826086955, -14.816521739130424, -18.267608695652164, -18.555652173913032, -24.707826086956512, -27.490434782608684, -26.04478260869564, -26.131739130434774, -24.29478260869564, -27.974130434782598, -30.60456521739129, -28.941521739130422, -37.218695652173906, -31.202391304347817, -24.50130434782608, -20.403478260869555, -11.425217391304336, -14.57195652173912, -16.055652173913032, -17.865434782608684, -16.490434782608684, -24.555652173913032, -29.077391304347813, -32.01217391304347, -33.1045652173913, -28.620869565217383, -22.099130434782598, -25.436086956521727, -26.876304347826075, -16.54478260869564, -15.267608695652163, -8.381739130434772, -4.452391304347815, -5.805652173913032, -7.33282608695651, -11.446956521739118, -17.153478260869555, -24.126304347826075, -26.555652173913032, -25.04478260869564, -20.91978260869564, -21.403478260869555, -23.76217391304347, -21.686086956521727, -24.45239130434782, -20.392608695652164, -15.914347826086946, -22.25130434782608, -22.186086956521727, -28.25673913043477, -27.83282608695651, -30.680652173913032, -30.25130434782608, -25.18608695652173, -30.29478260869564, -26.29478260869564, -22.164347826086942, -25.370869565217383, -25.7186956521739, -19.191521739130422, -25.50130434782608, -20.229565217391293, -22.52304347826086, -30.724130434782598, -32.13717391304347, -37.53391304347825, -33.914347826086946, -30.533913043478254, -27.789347826086946, -16.04478260869564, -12.148043478260858, -8.740434782608684, -6.506739130434771, -20.702391304347813, -25.832826086956512, -32.45239130434781, -33.35999999999999, -30.2241304347826, -26.300217391304336, -17.794782608695638, -11.64804347826086, -8.501304347826075, -12.827391304347815, -17.930652173913032, -17.816521739130422, -16.79478260869564, -18.12630434782608, -15.327391304347817, -22.16978260869564, -20.088260869565204, -17.566521739130422, -17.751304347826075, -11.778478260869553, -9.838260869565207, -9.82195652173912, -11.186086956521729, -16.838260869565204, -21.97956521739129, -20.41978260869564, -21.963260869565207, -25.52304347826086, -22.930652173913032, -24.582826086956512, -25.00130434782608, -24.664347826086946, -29.137173913043465, -26.767608695652164, -26.501304347826075, -17.56108695652173, -9.039347826086946, -9.544782608695641, -5.773043478260859, -6.7676086956521635, -13.224130434782598, -15.332826086956512, -19.365434782608688, -20.653478260869555, -20.300217391304336, -19.202391304347813, -16.191521739130422, -19.300217391304336, -12.789347826086946, -6.6589130434782495, -7.267608695652163, -5.044782608695641, -10.849130434782598, -13.251304347826077, -13.69695652173912, -14.838260869565206, -15.474130434782598, -17.012173913043465, -11.571956521739118, -9.32195652173912, -12.164347826086946, -20.41978260869564, -21.561086956521727, -18.158913043478247, -14.968695652173903, -2.838260869565206, -4.33282608695651, -9.137173913043467, -9.115434782608684, -14.169782608695641, -17.903478260869555, -19.724130434782598, -22.061086956521727, -22.446956521739118, -30.338260869565204, -32.39260869565216, -29.865434782608684, -27.941521739130422, -21.45782608695651, -20.343695652173903, -20.63717391304347, -20.202391304347813, -15.267608695652163, -12.729565217391293, -10.436086956521729, -8.430652173913032, -6.914347826086946, -1.4360869565217278, -1.5882608695652063, -6.153478260869554, -2.811086956521728, -4.392608695652163, -3.6263043478260757, -2.7349999999999888, -8.305652173913032, -16.175217391304336, -16.925217391304336, -13.843695652173903, -9.403478260869555, 2.3030434782608804, 3.7486956521739234, 3.955217391304359, 0.6889130434782718, -5.713260869565206, -5.501304347826075, -5.224130434782597, -8.811086956521727, -5.278478260869554, -4.484999999999989, -4.3002173913043364, -6.70782608695651, -5.718695652173902, -6.490434782608684, -9.278478260869553, -2.887173913043467, -5.403478260869553, -7.528478260869554, -2.7132608695652065, -7.7676086956521635, -5.876304347826076, -3.07195652173912, -0.46326086956520607, 2.8736956521739243, -7.528478260869555, -7.2132608695652065, -7.316521739130426, -5.914347826086947, -0.9034782608695533, -8.00673913043477, -15.756739130434772, -23.104565217391293, -24.349130434782598, -16.066521739130422, -17.740434782608684, -11.120869565217381, -8.213260869565207, -11.680652173913032, -3.5339130434782504, -7.050217391304337, 3.4823913043478365, 4.172608695652185, 4.188913043478271, 3.558478260869575, -7.245869565217381, -13.811086956521729, -20.441521739130426, -25.64804347826086, -20.289347826086946, -13.137173913043467, -9.533913043478249, 0.23239130434783695, -1.8708695652173803, -2.648043478260859, -4.506739130434772, -3.4306521739130322, -5.990434782608684, -6.37086956521738, -10.881739130434772, -13.952391304347817, -13.245869565217381, -17.066521739130426, -12.974130434782596, -9.941521739130424, -10.544782608695643, -5.87086956521738, -10.066521739130424, -13.267608695652163, -16.180652173913032, -14.756739130434772, -7.365434782608684, -9.577391304347815, -6.599130434782597, -9.653478260869553, -9.91978260869564, -11.02304347826086, -10.425217391304336, -4.555652173913033, -7.006739130434772, -5.756739130434772, -9.300217391304336, -14.566521739130426, -14.245869565217383, -5.767608695652164, -4.778478260869553, -2.5502173913043364, 2.531304347826098, -1.2513043478260757, -3.0665217391304234, -4.251304347826076, -2.3708695652173803, -7.615434782608684, 2.498695652173924, -2.5121739130434673, -7.501304347826076, 3.5530434782608804, 3.471521739130446, 1.5747826086956636, -2.4415217391304225, -16.00673913043477, -29.577391304347817, -20.707826086956512, -19.365434782608684, -16.571956521739118, -5.49586956521738, -10.164347826086946, -8.58282608695651, -0.7947826086956407, -2.631739130434771, 1.8302173913043591, 0.645434782608707, -5.305652173913032, -7.414347826086946, -10.061086956521729, -7.131739130434771, -7.859999999999989, -11.919782608695641, -4.686086956521727, 1.438913043478272, 1.4497826086956644, 0.7269565217391429, -1.1534782608695542, -10.088260869565206, -2.202391304347816, 3.2486956521739234, -6.555652173913033, -5.8002173913043364, -9.550217391304336, -8.077391304347813, 2.7486956521739243, 6.868260869565229, 4.3791304347826205, 4.705217391304359, 0.24326086956522852, -6.778478260869553, 0.645434782608707, -0.2839130434782496, 1.036739130434794, 5.536739130434794, 5.265000000000011, 5.00413043478262, 6.025869565217403, 7.922608695652185]
  out "CH3 Bin Readings":dbl[](array[numeric])=[7358.0, 7152.0, 7342.0, 7251.0, 7357.0, 7082.0, 7376.0, 7264.0, 7256.0, 7085.0, 7294.0, 7219.0, 7224.0, 7185.0, 7277.0, 7288.0, 7305.0, 7144.0, 7217.0, 7174.0, 7136.0, 7259.0, 7305.0, 7335.0, 7495.0, 7438.0, 7348.0, 7448.0, 7360.0, 7469.0, 7442.0, 7575.0, 7351.0, 7541.0, 7443.0, 7480.0, 7522.0, 7548.0, 7453.0, 7335.0, 7438.0, 7438.0, 7424.0, 7433.0, 7474.0, 7383.0, 7522.0, 7488.0, 7487.0, 7486.0, 7391.0, 7528.0, 7324.0, 7267.0, 7314.0, 7462.0, 7400.0, 7330.0, 7500.0, 7306.0, 7340.0, 7385.0, 7466.0, 7339.0, 7328.0, 7425.0, 7357.0, 7396.0, 7390.0, 7472.0, 7453.0, 7275.0, 7239.0, 7355.0, 7542.0, 8077.0, 38561.0, 64119.0, 1690.0, 65186.0, 49517.0, 20892.0, 8630.0, 7243.0, 7154.0, 7131.0, 7217.0, 6977.0, 7286.0, 6955.0, 7134.0, 7099.0, 7201.0, 7170.0, 7051.0, 7063.0, 7220.0, 7002.0, 7226.0, 7053.0, 7266.0, 7163.0, 7131.0, 7137.0, 7171.0, 7085.0, 7184.0, 7199.0, 7152.0, 7133.0, 7102.0, 7155.0, 7148.0, 7319.0, 7081.0, 7223.0, 7250.0, 7111.0, 6997.0, 7243.0, 7144.0, 7134.0, 7090.0, 7130.0, 7168.0, 7122.0, 7229.0, 7280.0, 7138.0, 7017.0, 7090.0, 7105.0, 7054.0, 7148.0, 7195.0, 7183.0, 7121.0, 7224.0, 7100.0, 7135.0, 7141.0, 7233.0, 7057.0, 7252.0, 7198.0, 7051.0, 7184.0, 7264.0, 7027.0, 7191.0, 7257.0, 7201.0, 7200.0, 7111.0, 7163.0, 7035.0, 7109.0, 7122.0, 7031.0, 7057.0, 7086.0, 7164.0, 7281.0, 7157.0, 7245.0, 7128.0, 7310.0, 7240.0, 7345.0, 7065.0, 7149.0, 7223.0, 7112.0, 7034.0, 7087.0, 7254.0, 6921.0, 7191.0, 7169.0, 7166.0, 7185.0, 7173.0, 7083.0, 7198.0, 7081.0, 7094.0, 7200.0, 7185.0, 7214.0, 7254.0, 7059.0, 7278.0, 7195.0, 7192.0, 6997.0, 7170.0, 7210.0, 7197.0, 7018.0, 7043.0, 7308.0, 7195.0, 7244.0, 7310.0, 6980.0, 7177.0, 7210.0, 7153.0, 7238.0, 7158.0, 7142.0, 7037.0, 6950.0, 7131.0, 7267.0, 7285.0, 7238.0, 7185.0, 7215.0, 7340.0, 7137.0, 7055.0, 7254.0, 7246.0, 7092.0, 6995.0, 7173.0, 7306.0, 7118.0, 7249.0, 7166.0, 7203.0, 7227.0, 7073.0, 7052.0, 7088.0, 7216.0, 7172.0, 7239.0, 7238.0, 7039.0, 7259.0, 7335.0, 7087.0, 7192.0, 7266.0, 7177.0, 7161.0, 7109.0, 7316.0, 7003.0, 7309.0, 7197.0, 7219.0, 7338.0, 7087.0, 7302.0, 7192.0, 7226.0, 7139.0, 7092.0, 7194.0, 7101.0, 6985.0, 7305.0, 7144.0, 7231.0, 7142.0, 7283.0, 7217.0, 7110.0, 7247.0, 7300.0, 7100.0, 7198.0, 7080.0, 7303.0, 7093.0, 7191.0, 7281.0, 7098.0, 7152.0, 7078.0, 7285.0, 7242.0, 7168.0, 7097.0, 7033.0, 7229.0, 7164.0, 7249.0, 7077.0, 7109.0, 7241.0, 7264.0, 7193.0, 7330.0, 7244.0, 7199.0, 7266.0, 7183.0, 7105.0, 7278.0, 7117.0, 7120.0, 7069.0, 7018.0, 7104.0, 7194.0, 7046.0, 7221.0, 7160.0, 7088.0, 7292.0, 7257.0, 7126.0, 7298.0, 7263.0, 7239.0, 7193.0, 7082.0, 7203.0, 7035.0, 7229.0, 7229.0, 7135.0, 7105.0, 7139.0, 7112.0, 7196.0, 7173.0, 7208.0, 7260.0, 7349.0, 7193.0, 7138.0, 7191.0, 7284.0, 7221.0, 7179.0, 7209.0, 7166.0, 7177.0, 7233.0, 6987.0, 7225.0, 7192.0, 7214.0, 7135.0, 7212.0, 7198.0, 7171.0, 7204.0, 7373.0, 7306.0, 7105.0, 7037.0, 7110.0, 7188.0, 7275.0, 7334.0, 7210.0, 7115.0, 7037.0, 7312.0, 7207.0, 7129.0, 7179.0, 7071.0, 7150.0, 7229.0, 7197.0, 7076.0, 7179.0, 7229.0, 7199.0, 7177.0, 7148.0, 7298.0, 7228.0, 7188.0, 7200.0, 7289.0, 7009.0, 7180.0, 7052.0, 7154.0, 7112.0, 7186.0, 7098.0, 7136.0, 7176.0, 7230.0, 7237.0, 7186.0, 7297.0, 7354.0, 7224.0, 7326.0, 7215.0, 7132.0, 7152.0, 7294.0, 7243.0, 7193.0, 7230.0, 7162.0, 7323.0, 7186.0, 7111.0, 7250.0, 7193.0, 7102.0, 7253.0, 7218.0, 7296.0, 7258.0, 7192.0, 7346.0, 7201.0, 7242.0, 7239.0, 7098.0, 7274.0, 7047.0, 7220.0, 7070.0, 7272.0, 7258.0, 7189.0, 7222.0, 7052.0, 7158.0, 7136.0, 7096.0, 7111.0, 7216.0, 7187.0, 7143.0, 7071.0, 7200.0, 7264.0, 7139.0, 7115.0, 7263.0, 7154.0, 7140.0, 7223.0, 7144.0, 7259.0, 7107.0, 7299.0, 7243.0, 7239.0, 7029.0, 7282.0, 7078.0, 7200.0, 7126.0, 7239.0, 7375.0, 7370.0, 7312.0, 7166.0, 7269.0, 7278.0, 7290.0, 7316.0, 7262.0, 7210.0, 7269.0, 7193.0, 7197.0, 7173.0, 6962.0, 7278.0, 7098.0, 7203.0, 7079.0, 7107.0, 7199.0, 7215.0, 7262.0, 7014.0, 7203.0, 7132.0, 7119.0, 7176.0, 7078.0, 7256.0, 7171.0, 7274.0, 7307.0, 7115.0, 7153.0, 7032.0, 7217.0, 7170.0, 7192.0, 7168.0, 7266.0, 7199.0, 7199.0, 7095.0, 7279.0, 7133.0, 7228.0, 7127.0, 7123.0, 7238.0, 7179.0, 7115.0, 7131.0, 7191.0, 7151.0, 7089.0, 7188.0, 7156.0, 7156.0, 7211.0, 7324.0, 7166.0, 7211.0, 7144.0, 7327.0, 7118.0, 7229.0, 7242.0, 7059.0, 7167.0, 7238.0, 7083.0, 7274.0, 7269.0, 7161.0, 7141.0, 7223.0, 7177.0, 7278.0, 7164.0, 7177.0, 7208.0, 7205.0, 7149.0, 7249.0, 7360.0, 7191.0, 7154.0, 7153.0, 7192.0, 7176.0, 7239.0, 7149.0, 7091.0, 7279.0, 7148.0, 7196.0, 7211.0, 7192.0]
  out "CH2 (molecular) smoothed":dbl[](array[numeric])=[-8.262500000000067, -7.802272727272793, -7.478409090909158, -13.739772727272793, -4.040909090909158, -9.21704545454552, -8.165909090909157, -3.84204545454552, -18.262500000000067, -9.864772727272793, -8.961363636363702, 1.3397727272726607, 17.56136363636357, 19.487499999999933, 21.055681818181753, 20.83977272727266, 24.709090909090843, 26.765909090909027, 25.635227272727207, 23.629545454545394, 23.021590909090843, 27.83977272727266, 33.52727272727266, 33.85113636363629, 40.01022727272721, 44.01590909090903, 53.04999999999993, 60.4136363636363, 50.67499999999993, 43.26590909090903, 40.38522727272721, 38.873863636363566, 43.60681818181811, 48.40227272727266, 45.4136363636363, 45.19772727272721, 45.76022727272721, 45.20340909090902, 53.54431818181811, 56.16931818181812, 60.0386363636363, 54.56704545454539, 49.44772727272721, 49.39659090909084, 47.77727272727267, 56.46477272727266, 54.88522727272721, 51.14659090909085, 45.07272727272721, 41.58977272727266, 39.85681818181811, 44.72045454545448, 48.17499999999994, 47.79999999999993, 41.8511363636363, 36.52159090909085, 36.40795454545448, 43.20909090909085, 48.16931818181812, 47.697727272727214, 46.67499999999994, 36.43636363636357, 37.64090909090903, 34.4136363636363, 31.567045454545386, 37.29431818181811, 42.10681818181811, 41.82272727272721, 40.94204545454539, 37.10681818181811, 22.53295454545448, 23.123863636363573, 14.82272727272721, 33.51022727272721, 233.14090909090902, 511.52159090909083, 694.6920454545455, 754.0045454545455, 570.4363636363636, 290.9193181818182, 105.51590909090902, 17.112499999999937, -9.756818181818248, -24.580681818181883, -25.68295454545461, -29.921590909090973, -28.569318181818247, -24.239772727272793, -23.450000000000067, -25.290909090909157, -21.47272727272734, -14.93863636363643, -8.768181818181883, -11.43863636363643, -11.353409090909157, -16.569318181818247, -19.756818181818247, -17.6488636363637, -19.847727272727337, -12.65454545454552, -13.53522727272734, -8.78522727272734, -1.6488636363637026, -2.359090909090976, -6.603409090909157, -9.603409090909157, -12.444318181818248, -11.711363636363702, -11.84772727272734, -8.739772727272793, -11.256818181818248, -18.773863636363703, -20.870454545454614, -24.24545454545461, -21.557954545454614, -27.705681818181887, -25.853409090909157, -28.0238636363637, -27.7738636363637, -22.887500000000063, -19.614772727272793, -14.978409090909157, -15.637500000000067, -10.273863636363702, -8.52954545454552, -15.217045454545522, -10.25113636363643, -10.325000000000067, -18.665909090909157, -8.052272727272793, -11.80795454545461, -9.27954545454552, -16.427272727272793, -20.700000000000067, -24.404545454545516, -32.17727272727279, -18.745454545454614, -24.040909090909157, -14.694318181818248, -18.762500000000067, -24.893181818181883, -27.78522727272734, -31.876136363636427, -28.68863636363643, -25.177272727272793, -20.637500000000067, -30.21704545454552, -22.325000000000067, -25.114772727272793, -12.722727272727337, -7.915909090909157, -18.228409090909157, -19.802272727272793, -29.16022727272734, -31.52954545454552, -33.47840909090915, -31.99545454545461, -32.74545454545461, -29.10340909090916, -14.171590909090977, -6.898863636363702, -9.046590909090975, -12.700000000000067, -15.78522727272734, -19.22272727272734, -15.859090909090973, -13.006818181818247, -16.785227272727337, -18.0863636363637, -11.34204545454552, -11.165909090909159, -13.75113636363643, -7.307954545454612, -13.302272727272793, -11.830681818181883, -10.086363636363702, -10.59204545454552, -10.944318181818247, -8.944318181818247, -8.523863636363702, -17.182954545454614, -17.120454545454614, -17.984090909090973, -15.415909090909157, -10.745454545454612, -7.50113636363643, -16.023863636363703, -10.006818181818247, -5.15454545454552, -12.34204545454552, -8.239772727272793, -15.84204545454552, -11.648863636363703, -6.228409090909157, 1.31136363636357, 3.7715909090908424, 3.5215909090908424, 2.7659090909090236, -4.421590909090977, -2.22272727272734, -11.052272727272793, -7.307954545454612, -8.450000000000067, -6.126136363636429, 1.0784090909090245, -5.154545454545522, 1.4761363636362963, -7.489772727272793, -13.819318181818248, -9.540909090909157, -6.336363636363702, -3.870454545454611, -7.609090909090975, -9.898863636363702, -23.7113636363637, -32.09204545454552, -26.18863636363643, -35.34204545454552, -34.9613636363637, -30.34204545454552, -27.15454545454552, -13.802272727272793, -5.540909090909157, -6.506818181818248, -11.012500000000067, -17.870454545454614, -19.10340909090916, -15.717045454545522, -22.268181818181887, -11.773863636363703, -12.53522727272734, -8.28522727272734, -2.9954545454546118, -10.109090909090975, -16.34204545454552, -17.421590909090977, -12.830681818181885, -15.995454545454614, -6.359090909090975, -4.887500000000066, -6.131818181818248, -1.3647727272727934, -3.1318181818182484, -7.43863636363643, -5.700000000000067, -9.200000000000067, -8.461363636363703, -2.870454545454613, -6.171590909090977, -3.654545454545521, -5.336363636363703, -11.637500000000067, -5.035227272727339, -13.296590909090975, -11.234090909090975, -14.853409090909157, -19.97272727272734, -9.620454545454614, -10.842045454545522, -3.8931818181818842, -1.637500000000066, -6.131818181818248, -8.71704545454552, -16.296590909090973, -22.66022727272734, -19.603409090909157, -12.205681818181885, -9.66022727272734, -8.444318181818247, -11.30795454545461, -12.057954545454612, -13.18295454545461, -7.557954545454611, -7.165909090909158, -15.586363636363703, -11.671590909090975, -12.194318181818247, -10.518181818181885, -4.370454545454612, -3.6545454545455205, -14.609090909090977, -18.711363636363703, -20.677272727272797, -14.63181818181825, -4.620454545454613, -2.7397727272727943, -2.3193181818182484, -10.34772727272734, -19.22272727272734, -22.734090909090973, -17.47272727272734, -21.484090909090973, -8.381818181818247, -5.097727272727338, -7.4556818181818825, -2.0409090909091567, -6.569318181818247, -7.586363636363703, -10.052272727272793, -11.870454545454612, -17.96704545454552, -15.455681818181883, -12.910227272727338, -10.160227272727338, -4.6318181818182484, -10.131818181818248, -19.194318181818247, -10.31931818181825, -12.234090909090977, -9.37613636363643, -5.671590909090976, -13.995454545454612, -15.245454545454612, -12.739772727272792, -13.205681818181883, -9.228409090909157, -10.069318181818248, -10.518181818181883, -6.8193181818182484, -12.00113636363643, -14.819318181818248, -14.381818181818247, -12.347727272727338, -16.978409090909157, -6.307954545454611, -11.586363636363703, -7.575000000000066, -2.5806818181818842, -8.046590909090975, -1.1375000000000655, 1.845454545454479, 3.0272727272726616, -4.637500000000066, 8.686363636363572, -2.319318181818247, -11.131818181818247, -4.495454545454612, -16.614772727272793, -22.10340909090916, -11.671590909090977, -9.950000000000067, -10.02954545454552, -6.393181818181884, -5.1318181818182484, -5.086363636363703, -5.739772727272793, -2.06363636363643, -5.682954545454612, -5.50113636363643, -2.194318181818248, 1.7261363636362974, 4.709090909090842, 2.7999999999999337, -3.773863636363703, -9.512500000000065, -12.540909090909157, -5.5693181818182484, -5.109090909090975, 2.521590909090843, 2.3795454545453882, -9.648863636363702, -5.063636363636429, -12.211363636363702, -11.62045454545461, 1.7943181818181158, -2.364772727272793, 1.7034090909090256, 2.9761363636362983, 2.0386363636362983, -0.2511363636364292, -6.137500000000066, -9.103409090909157, -17.319318181818247, -14.66022727272734, 1.2943181818181166, 7.623863636363572, 6.544318181818116, 6.743181818181753, -4.336363636363703, -6.961363636363703, -5.245454545454612, -1.6147727272727934, -8.177272727272793, -15.37613636363643, -14.580681818181883, -13.773863636363703, -13.018181818181885, -3.2227272727273384, -5.6318181818182484, -8.52954545454552, 0.03295454545447907, -5.575000000000066, -3.546590909090975, -6.097727272727338, -8.711363636363702, -7.84204545454552, -8.887500000000067, -11.978409090909157, -9.552272727272792, -20.012500000000067, -15.222727272727338, -10.00113636363643, -16.319318181818247, -11.177272727272793, -8.557954545454612, -9.15454545454552, -6.415909090909158, -1.9613636363637026, -10.950000000000067, -16.052272727272793, -23.807954545454614, -20.796590909090977, -16.467045454545524, -4.842045454545521, 0.20909090909084327, 3.174999999999934, -1.171590909090975, -2.5011363636364297, -6.575000000000067, -12.944318181818248, -2.06363636363643, -8.194318181818247, -2.2795454545455205, -0.6034090909091568, -7.120454545454612, -8.131818181818247, -7.268181818181885, -10.56363636363643, -10.682954545454612, -3.8704545454546118, -8.881818181818247, -0.9556818181818842, 0.7261363636362976, -4.552272727272793, 3.2943181818181153, 3.7659090909090245, 5.43636363636357, 11.356818181818115, 10.976136363636298, 5.7431818181817516, -1.0352272727273388, -11.262500000000067, -20.359090909090973, -20.864772727272793, -15.785227272727338, -0.20568181818188336, 8.663636363636297, 16.442045454545386, 15.12954545454539, 8.010227272727207, 4.538636363636297, -7.222727272727339, -11.171590909090977, -9.262500000000067, -7.313636363636429, -3.154545454545521, 4.334090909090843, 5.993181818181752, 6.356818181818116, 1.7147727272726616, 0.9590909090908433, -4.62613636363643, -7.961363636363703, -8.421590909090975, -13.620454545454612, -8.830681818181883, -4.137500000000066, 2.2829545454544795, -2.950000000000066, -2.262500000000066, -1.978409090909158, 6.2715909090908415, 9.135227272727205, 7.271590909090842, 8.379545454545386, -4.3193181818182484, 1.7772727272726607, -0.9272727272727939, -11.665909090909157, -11.05795454545461, -19.614772727272793, -18.160227272727337, -4.489772727272793, -8.870454545454614, 1.4420454545453882, 2.1124999999999337, -1.7454545454546118, -1.154545454545521, -8.12613636363643, -10.972727272727338, -20.43863636363643, -10.211363636363702, -12.87613636363643, -22.228409090909157, -24.603409090909157, -22.859090909090977, -20.205681818181883, -12.319318181818248, 2.2829545454544786, -8.859090909090975, -0.7681818181818842, 4.265909090909025, -6.21704545454552, -1.1147727272727932, -3.15454545454552, -1.1488636363637026, -3.1204545454546118, 1.2772727272726612, 6.231818181818115, -1.0750000000000668, 7.7261363636362965, 3.37386363636357, -1.5068181818182482, -6.234090909090976, -8.455681818181885, -11.290909090909157, -17.31363636363643, -7.7738636363637035, -6.006818181818248, 3.220454545454479, 5.9306818181817516, 0.23181818181811575, -2.092045454545521, -5.057954545454612, -4.057954545454612, 3.8624999999999337, -2.262500000000067, -2.239772727272794, -6.745454545454612, -9.273863636363702, -7.234090909090975, -7.523863636363703, -0.14886363636370237, -8.859090909090975, 0.06704545454538868, -1.6090909090909742, 1.674999999999934, 14.947727272727207, 8.99886363636357, 11.521590909090843, 3.4874999999999337, -2.7340909090909755, -0.32500000000006635, -0.5238636363637026, 5.470454545454479, 2.1522727272726607, -1.296590909090976, -6.529545454545521, -9.637500000000067, -10.898863636363703, -2.330681818181885, 4.669318181818115, 10.442045454545386, 9.606818181818115, 2.0784090909090236]
  out "CH 2 Bin Readings":dbl[](array[numeric])=[13746.0, 13515.0, 13729.0, 13765.0, 13722.0, 13858.0, 13624.0, 13492.0, 13584.0, 13798.0, 13716.0, 13769.0, 13457.0, 13597.0, 13524.0, 13687.0, 13652.0, 13884.0, 13618.0, 13683.0, 13642.0, 13554.0, 13656.0, 13554.0, 13640.0, 13751.0, 13707.0, 13662.0, 13923.0, 13858.0, 13640.0, 13686.0, 13769.0, 13514.0, 13644.0, 13874.0, 13688.0, 13830.0, 13873.0, 13614.0, 13895.0, 13580.0, 13502.0, 13590.0, 13594.0, 13913.0, 13714.0, 13671.0, 13558.0, 13902.0, 13514.0, 13568.0, 13675.0, 13821.0, 13607.0, 13732.0, 13919.0, 13661.0, 13681.0, 13782.0, 13622.0, 13670.0, 13714.0, 13701.0, 13753.0, 13664.0, 13679.0, 13654.0, 13605.0, 13586.0, 13419.0, 13521.0, 13838.0, 13721.0, 13739.0, 13642.0, 13673.0, 14571.0, 14922.0, 14816.0, 14111.0, 13983.0, 13470.0, 13539.0, 13608.0, 13453.0, 13585.0, 13673.0, 13725.0, 13580.0, 13683.0, 13584.0, 13602.0, 13505.0, 13715.0, 13647.0, 13555.0, 13354.0, 13373.0, 13646.0, 13538.0, 13655.0, 13465.0, 13570.0, 13680.0, 13802.0, 13584.0, 13680.0, 13490.0, 13662.0, 13678.0, 13613.0, 13437.0, 13644.0, 13807.0, 13613.0, 13731.0, 13526.0, 13554.0, 13527.0, 13644.0, 13472.0, 13624.0, 13554.0, 13920.0, 13522.0, 13665.0, 13493.0, 13662.0, 13528.0, 13805.0, 13746.0, 13745.0, 13488.0, 13719.0, 13812.0, 13692.0, 13668.0, 13702.0, 13679.0, 13626.0, 13611.0, 13538.0, 13498.0, 13676.0, 13544.0, 13867.0, 13513.0, 13451.0, 13685.0, 13585.0, 13679.0, 13661.0, 13575.0, 13779.0, 13767.0, 13656.0, 13542.0, 13563.0, 13594.0, 13724.0, 13714.0, 13573.0, 13731.0, 13462.0, 13655.0, 13728.0, 13770.0, 13573.0, 13567.0, 13392.0, 13676.0, 13585.0, 13484.0, 13455.0, 13485.0, 13654.0, 13743.0, 13715.0, 13717.0, 13543.0, 13749.0, 13559.0, 13665.0, 13680.0, 13543.0, 13733.0, 13521.0, 13675.0, 13719.0, 13860.0, 13597.0, 13633.0, 13639.0, 13608.0, 13707.0, 13676.0, 13555.0, 13598.0, 13496.0, 13648.0, 13577.0, 13583.0, 13669.0, 13509.0, 13576.0, 13412.0, 13740.0, 13598.0, 13571.0, 13737.0, 13446.0, 13770.0, 13400.0, 13753.0, 13560.0, 13713.0, 13583.0, 13599.0, 13903.0, 13598.0, 13835.0, 13952.0, 13567.0, 13844.0, 13526.0, 13531.0, 13544.0, 13647.0, 13775.0, 13596.0, 13419.0, 13618.0, 13534.0, 13563.0, 13469.0, 13520.0, 13569.0, 13694.0, 13812.0, 13641.0, 13575.0, 13464.0, 13745.0, 13737.0, 13812.0, 13728.0, 13487.0, 13631.0, 13626.0, 13673.0, 13613.0, 13481.0, 13614.0, 13664.0, 13628.0, 13593.0, 13387.0, 13733.0, 13427.0, 13674.0, 13654.0, 13806.0, 13702.0, 13546.0, 13699.0, 13502.0, 13826.0, 13664.0, 13648.0, 13567.0, 13640.0, 13554.0, 13465.0, 13783.0, 13496.0, 13764.0, 13520.0, 13593.0, 13736.0, 13647.0, 13528.0, 13707.0, 13421.0, 13644.0, 13631.0, 13591.0, 13595.0, 13698.0, 13699.0, 13573.0, 13639.0, 13864.0, 13820.0, 13430.0, 13603.0, 13544.0, 13589.0, 13512.0, 13520.0, 13648.0, 13676.0, 13746.0, 13488.0, 13457.0, 13505.0, 13666.0, 13632.0, 13631.0, 13325.0, 13809.0, 13779.0, 13642.0, 13497.0, 13659.0, 13596.0, 13749.0, 13509.0, 13390.0, 13702.0, 13515.0, 13672.0, 13412.0, 13564.0, 13757.0, 13407.0, 13792.0, 13796.0, 13577.0, 13585.0, 13720.0, 13507.0, 13615.0, 13507.0, 13723.0, 13490.0, 13643.0, 13669.0, 13717.0, 13634.0, 13805.0, 13534.0, 13554.0, 13452.0, 13436.0, 13505.0, 13849.0, 13538.0, 13773.0, 13526.0, 13609.0, 13777.0, 13789.0, 13698.0, 13542.0, 13500.0, 13481.0, 13447.0, 13512.0, 13730.0, 13587.0, 13457.0, 13488.0, 13482.0, 13737.0, 13665.0, 13633.0, 13513.0, 13640.0, 13742.0, 13646.0, 13647.0, 13727.0, 13626.0, 13539.0, 13609.0, 13614.0, 13791.0, 13541.0, 13519.0, 13494.0, 13552.0, 13611.0, 13688.0, 13535.0, 13706.0, 13653.0, 13725.0, 13663.0, 13796.0, 13533.0, 13498.0, 13521.0, 13773.0, 13568.0, 13733.0, 13679.0, 13589.0, 13601.0, 13606.0, 13705.0, 13615.0, 13613.0, 13743.0, 13477.0, 13541.0, 13616.0, 13702.0, 13602.0, 13679.0, 13649.0, 13593.0, 13634.0, 13767.0, 13737.0, 13672.0, 13729.0, 13641.0, 13693.0, 13534.0, 13759.0, 13645.0, 13434.0, 13506.0, 13525.0, 13644.0, 13526.0, 13746.0, 13683.0, 13506.0, 13555.0, 13740.0, 13409.0, 13752.0, 13793.0, 13680.0, 13393.0, 13686.0, 13563.0, 13554.0, 13814.0, 13438.0, 13709.0, 13553.0, 13630.0, 13684.0, 13739.0, 13457.0, 13794.0, 13487.0, 13465.0, 13502.0, 13814.0, 13579.0, 13398.0, 13495.0, 13597.0, 13693.0, 13581.0, 13638.0, 13408.0, 13514.0, 13824.0, 13646.0, 13845.0, 13801.0, 13547.0, 13549.0, 13767.0, 13660.0, 13659.0, 13658.0, 13435.0, 13703.0, 13489.0, 13632.0, 13743.0, 13584.0, 13603.0, 13521.0, 13668.0, 13676.0, 13645.0, 13640.0, 13645.0, 13639.0, 13512.0, 13652.0, 13659.0, 13399.0, 13610.0, 13750.0, 13659.0, 13466.0, 13856.0, 13907.0, 13854.0, 13574.0, 13385.0, 13607.0, 13660.0, 13590.0, 13682.0, 13671.0, 13633.0, 13657.0, 13592.0, 13592.0, 13635.0, 13726.0, 13723.0, 13615.0, 13503.0, 13713.0, 13672.0, 13823.0, 13650.0, 13820.0, 13590.0, 13577.0, 13569.0, 13606.0, 13693.0, 13683.0, 13624.0, 13532.0, 13508.0, 13547.0, 13532.0, 13568.0, 13608.0, 13799.0, 13576.0, 13741.0, 13598.0, 13568.0, 13537.0, 13754.0, 13583.0, 13403.0, 13697.0, 13521.0, 13599.0, 13665.0, 13419.0, 13802.0, 13691.0, 13753.0, 13686.0, 13853.0, 13579.0, 13728.0, 13627.0, 13500.0, 13590.0, 13671.0, 13590.0, 13777.0, 13659.0]
  in  "stop":bool
  in  "Reset Average":bool=TRUE
  in  "Save Data?":bool=TRUE
  in  "Collect Data?":bool=TRUE
  in  "ILX Address":i32=6 min=0 step=1
  in  "Lambda On DBR Current":dbl=171.13999999999868
  in  "Lambda Off DBR Current":dbl=172.9499999999997
  in  "Tab Control":T2(tab)=enum."NRB"
  out "NRB plot":cluster{"Y":dbl[], "Y":dbl[]}[](graph)=[{"Y"=[0.0, 0.0, 0.0, 0.0, 0.0, 0.0, 0.0, 0.0, 0.0, 0.0, 0.0, 0.0, 0.0, 0.0, 0.0, 0.0, 0.0, 0.0, 0.0, 0.0, 0.0, 0.0, 0.0, 0.0, 0.0, 0.0, 0.0, 0.0, 0.0, 0.0, 0.0, 0.0, 0.0, 0.0, 0.0, 0.0, 0.0, 0.0, 0.0, 0.0, 0.0, 0.0, 0.0, 0.0, 0.0, 0.0, 0.0, 0.0, 0.0, 0.0, 0.0, 0.0, 0.0, 0.0, 0.0, 0.0, 0.0, 0.0, 0.0, 0.0, 0.0, 0.0, 0.0, 0.0, 0.0, 0.0, 0.0, 0.0, 0.0, 0.0, 0.0, 0.0, 0.0, 0.0, 0.0, 0.0, 0.0, 0.0, 0.0, 0.0, 0.0, 0.0, 0.0, 0.0, 0.0, 0.0, 0.0, 0.0, 0.0, 0.0, 0.0, 0.0, 0.0, 0.0, 0.0, 0.0, 0.0, 0.0, 0.0, 0.0, 0.0, 0.0, 0.0, 0.0, 0.0, 0.0, 0.0, 0.0, 0.0, 0.0, 0.0, 0.0, 0.0, 0.0, 0.0, 0.0, 0.0, 0.0, 0.0, 0.0, 0.0, 0.0, 0.0, 0.0, 0.0, 0.0, 0.0, 0.0, 0.0, 0.0, 0.0, 0.0, 0.0, 0.0, 0.0, 0.0, 0.0, 0.0, 0.0, 0.0, 0.0, 0.0, 0.0, 0.0, 0.0, 0.0, 0.0, 0.0, 0.0, 0.0, 0.0, 0.0, 0.0, 0.0, 0.0, 0.0, 0.0, 0.0, 0.0, 0.0, 0.0, 0.0, 0.0, 0.0, 0.0, 0.0, 0.0, 0.0, 0.0, 0.0, 0.0, 0.0, 0.0, 0.0, 0.0, 0.0, 0.0, 0.0, 0.0, 0.0, 0.0, 0.0, 0.0, 0.0, 0.0, 0.0, 0.0, 0.0, 0.0, 0.0, 0.0, 0.0, 0.0, 0.0, 0.0, 0.0, 0.0, 0.0, 0.0, 0.0, 0.0, 0.0, 0.0, 0.0, 0.0, 0.0, 0.0, 0.0, 0.0, 0.0, 0.0, 0.0, 0.0, 0.0, 0.0, 0.0, 0.0, 0.0, 0.0, 0.0, 0.0, 0.0, 0.0, 0.0, 0.0, 0.0, 0.0, 0.0, 0.0, 0.0, 0.0, 0.0, 0.0, 0.0, 0.0, 0.0, 0.0, 0.0, 0.0, 0.0, 0.0, 0.0, 0.0, 0.0, 0.0, 0.0, 0.0, 0.0, 0.0, 0.0, 0.0, 0.0, 0.0, 0.0, 0.0, 0.0, 0.0, 0.0, 0.0, 0.0, 0.0, 0.0, 0.0, 0.0, 0.0, 0.0, 0.0, 0.0, 0.0, 0.0, 0.0, 0.0, 0.0, 0.0, 0.0, 0.0, 0.0, 0.0, 0.0, 0.0, 0.0, 0.0, 0.0, 0.0, 0.0, 0.0, 0.0, 0.0, 0.0, 0.0, 0.0, 0.0, 0.0, 0.0, 0.0, 0.0, 0.0, 0.0, 0.0, 0.0, 0.0, 0.0, 0.0, 0.0, 0.0, 0.0, 0.0, 0.0, 0.0, 0.0, 0.0, 0.0, 0.0, 0.0, 0.0, 0.0, 0.0, 0.0, 0.0, 0.0, 0.0, 0.0, 0.0, 0.0, 0.0, 0.0, 0.0, 0.0, 0.0, 0.0, 0.0, 0.0, 0.0, 0.0, 0.0, 0.0, 0.0, 0.0, 0.0, 0.0, 0.0, 0.0, 0.0, 0.0, 0.0, 0.0, 0.0, 0.0, 0.0, 0.0, 0.0, 0.0, 0.0, 0.0, 0.0, 0.0, 0.0, 0.0, 0.0, 0.0, 0.0, 0.0, 0.0, 0.0, 0.0, 0.0, 0.0, 0.0, 0.0, 0.0, 0.0, 0.0, 0.0, 0.0, 0.0, 0.0, 0.0, 0.0, 0.0, 0.0, 0.0, 0.0, 0.0, 0.0, 0.0, 0.0, 0.0, 0.0, 0.0, 0.0, 0.0, 0.0, 0.0, 0.0, 0.0, 0.0, 0.0, 0.0, 0.0, 0.0, 0.0, 0.0, 0.0, 0.0, 0.0, 0.0, 0.0, 0.0, 0.0, 0.0, 0.0, 0.0, 0.0, 0.0, 0.0, 0.0, 0.0, 0.0, 0.0, 0.0, 0.0, 0.0, 0.0, 0.0, 0.0, 0.0, 0.0, 0.0, 0.0, 0.0, 0.0, 0.0, 0.0, 0.0, 0.0, 0.0, 0.0, 0.0, 0.0, 0.0, 0.0, 0.0, 0.0, 0.0, 0.0, 0.0, 0.0, 0.0, 0.0, 0.0, 0.0, 0.0, 0.0, 0.0, 0.0, 0.0, 0.0, 0.0, 0.0, 0.0, 0.0, 0.0, 0.0, 0.0, 0.0, 0.0, 0.0, 0.0, 0.0, 0.0, 0.0, 0.0, 0.0, 0.0, 0.0, 0.0, 0.0, 0.0, 0.0, 0.0, 0.0, 0.0, 0.0, 0.0, 0.0, 0.0, 0.0, 0.0, 0.0, 0.0, 0.0, 0.0, 0.0, 0.0, 0.0, 0.0, 0.0, 0.0, 0.0, 0.0, 0.0, 0.0, 0.0, 0.0, 0.0, 0.0, 0.0, 0.0, 0.0, 0.0, 0.0, 0.0, 0.0, 0.0, 0.0, 0.0, 0.0, 0.0, 0.0, 0.0, 0.0, 0.0, 0.0, 0.0, 0.0, 0.0, 0.0, 0.0, 0.0, 0.0, 0.0, 0.0, 0.0, 0.0, 0.0, 0.0, 0.0, 0.0, 0.0, 0.0, 0.0, 0.0, 0.0, 0.0, 0.0, 0.0, 0.0, 0.0, 0.0, 0.0, 0.0, 0.0, 0.0, 0.0, 0.0], "Y"=[0.0375, 0.075, 0.11249999999999999, 0.15, 0.1875, 0.225, 0.26249999999999996, 0.3, 0.33749999999999997, 0.37499999999999994, 0.4125, 0.44999999999999996, 0.48749999999999993, 0.525, 0.5625, 0.6, 0.6375, 0.6749999999999999, 0.7124999999999999, 0.75, 0.7875, 0.825, 0.8624999999999999, 0.8999999999999999, 0.9374999999999999, 0.975, 1.0125, 1.05, 1.0875000000000001, 1.125, 1.1625, 1.2, 1.2375, 1.2750000000000001, 1.3125, 1.35, 1.3875, 1.425, 1.4625000000000001, 1.5, 1.5375, 1.575, 1.6125, 1.6500000000000001, 1.6875, 1.725, 1.7625, 1.8, 1.8375, 1.875, 1.9125, 1.95, 1.9875, 2.025, 2.0625, 2.1, 2.1375, 2.175, 2.2125, 2.25, 2.2875, 2.325, 2.3625, 2.4, 2.4375, 2.475, 2.5125, 2.55, 2.5875, 2.625, 2.6625, 2.7, 2.7375, 2.775, 2.8125, 2.85, 2.8875, 2.925, 2.9625, 3.0, 3.0375, 3.075, 3.1125, 3.15, 3.1875, 3.225, 3.2625, 3.3, 3.3375, 3.375, 3.4125, 3.45, 3.4875, 3.525, 3.5625, 3.6, 3.6374999999999997, 3.675, 3.7125, 3.75, 3.7875, 3.8249999999999997, 3.8625, 3.9, 3.9375, 3.975, 4.012499999999999, 4.05, 4.0874999999999995, 4.124999999999999, 4.1625, 4.199999999999999, 4.2375, 4.2749999999999995, 4.312499999999999, 4.35, 4.387499999999999, 4.425, 4.4624999999999995, 4.499999999999999, 4.5375, 4.574999999999999, 4.6125, 4.6499999999999995, 4.687499999999999, 4.725, 4.762499999999999, 4.8, 4.8374999999999995, 4.874999999999999, 4.9125, 4.949999999999999, 4.9875, 5.0249999999999995, 5.062499999999999, 5.1, 5.137499999999999, 5.175, 5.2124999999999995, 5.249999999999999, 5.2875, 5.324999999999999, 5.3625, 5.3999999999999995, 5.437499999999999, 5.475, 5.512499999999999, 5.55, 5.5874999999999995, 5.624999999999999, 5.6625, 5.699999999999999, 5.7375, 5.7749999999999995, 5.812499999999999, 5.85, 5.887499999999999, 5.925, 5.9624999999999995, 5.999999999999999, 6.0375, 6.074999999999999, 6.1125, 6.1499999999999995, 6.187499999999999, 6.225, 6.262499999999999, 6.3, 6.3374999999999995, 6.374999999999999, 6.4125, 6.449999999999999, 6.4875, 6.5249999999999995, 6.562499999999999, 6.6, 6.637499999999999, 6.675, 6.7124999999999995, 6.749999999999999, 6.7875, 6.824999999999999, 6.8625, 6.8999999999999995, 6.937499999999999, 6.975, 7.012499999999999, 7.05, 7.0874999999999995, 7.124999999999999, 7.1625, 7.199999999999999, 7.237499999999999, 7.2749999999999995, 7.312499999999999, 7.35, 7.387499999999999, 7.424999999999999, 7.4624999999999995, 7.499999999999999, 7.5375, 7.574999999999999, 7.612499999999999, 7.6499999999999995, 7.687499999999999, 7.725, 7.762499999999999, 7.799999999999999, 7.8374999999999995, 7.874999999999999, 7.9125, 7.949999999999999, 7.987499999999999, 8.025, 8.0625, 8.1, 8.1375, 8.174999999999999, 8.212499999999999, 8.25, 8.2875, 8.325, 8.362499999999999, 8.399999999999999, 8.4375, 8.475, 8.5125, 8.549999999999999, 8.587499999999999, 8.625, 8.6625, 8.7, 8.737499999999999, 8.774999999999999, 8.8125, 8.85, 8.8875, 8.924999999999999, 8.962499999999999, 9.0, 9.0375, 9.075, 9.112499999999999, 9.149999999999999, 9.1875, 9.225, 9.2625, 9.299999999999999, 9.337499999999999, 9.375, 9.4125, 9.45, 9.487499999999999, 9.524999999999999, 9.5625, 9.6, 9.6375, 9.674999999999999, 9.712499999999999, 9.75, 9.7875, 9.825, 9.862499999999999, 9.899999999999999, 9.9375, 9.975, 10.0125, 10.049999999999999, 10.087499999999999, 10.125, 10.1625, 10.2, 10.237499999999999, 10.274999999999999, 10.3125, 10.35, 10.3875, 10.424999999999999, 10.462499999999999, 10.5, 10.5375, 10.575, 10.612499999999999, 10.649999999999999, 10.6875, 10.725, 10.7625, 10.799999999999999, 10.837499999999999, 10.875, 10.9125, 10.95, 10.987499999999999, 11.024999999999999, 11.0625, 11.1, 11.1375, 11.174999999999999, 11.212499999999999, 11.25, 11.2875, 11.325, 11.362499999999999, 11.399999999999999, 11.4375, 11.475, 11.5125, 11.549999999999999, 11.587499999999999, 11.625, 11.6625, 11.7, 11.737499999999999, 11.774999999999999, 11.8125, 11.85, 11.8875, 11.924999999999999, 11.962499999999999, 12.0, 12.0375, 12.075, 12.112499999999999, 12.149999999999999, 12.1875, 12.225, 12.2625, 12.299999999999999, 12.337499999999999, 12.375, 12.4125, 12.45, 12.487499999999999, 12.524999999999999, 12.5625, 12.6, 12.6375, 12.674999999999999, 12.712499999999999, 12.75, 12.7875, 12.825, 12.862499999999999, 12.899999999999999, 12.9375, 12.975, 13.0125, 13.049999999999999, 13.087499999999999, 13.125, 13.1625, 13.2, 13.237499999999999, 13.274999999999999, 13.3125, 13.35, 13.3875, 13.424999999999999, 13.462499999999999, 13.5, 13.5375, 13.575, 13.612499999999999, 13.649999999999999, 13.6875, 13.725, 13.7625, 13.799999999999999, 13.837499999999999, 13.875, 13.9125, 13.95, 13.987499999999999, 14.024999999999999, 14.0625, 14.1, 14.1375, 14.174999999999999, 14.212499999999999, 14.25, 14.2875, 14.325, 14.362499999999999, 14.399999999999999, 14.437499999999998, 14.475, 14.5125, 14.549999999999999, 14.587499999999999, 14.624999999999998, 14.6625, 14.7, 14.737499999999999, 14.774999999999999, 14.812499999999998, 14.85, 14.8875, 14.924999999999999, 14.962499999999999, 14.999999999999998, 15.0375, 15.075, 15.112499999999999, 15.149999999999999, 15.187499999999998, 15.225, 15.2625, 15.299999999999999, 15.337499999999999, 15.374999999999998, 15.4125, 15.45, 15.487499999999999, 15.524999999999999, 15.562499999999998, 15.6, 15.6375, 15.674999999999999, 15.712499999999999, 15.749999999999998, 15.7875, 15.825, 15.862499999999999, 15.899999999999999, 15.937499999999998, 15.975, 16.0125, 16.05, 16.087500000000002, 16.125, 16.1625, 16.2, 16.2375, 16.275000000000002, 16.3125, 16.35, 16.3875, 16.425, 16.462500000000002, 16.5, 16.5375, 16.575, 16.6125, 16.650000000000002, 16.6875, 16.725, 16.7625, 16.8, 16.837500000000002, 16.875, 16.9125, 16.95, 16.9875, 17.025000000000002, 17.0625, 17.1, 17.1375, 17.175, 17.212500000000002, 17.25, 17.2875, 17.325, 17.3625, 17.400000000000002, 17.4375, 17.475, 17.5125, 17.55, 17.587500000000002, 17.625, 17.6625, 17.7, 17.7375, 17.775000000000002, 17.8125, 17.85, 17.8875, 17.925, 17.962500000000002, 18.0, 18.0375, 18.075, 18.1125, 18.150000000000002, 18.1875, 18.225, 18.2625, 18.3, 18.337500000000002, 18.375, 18.4125, 18.45, 18.4875, 18.525000000000002, 18.5625, 18.6, 18.6375, 18.675, 18.712500000000002, 18.75, 18.7875, 18.825, 18.8625, 18.900000000000002, 18.9375, 18.975, 19.0125, 19.05, 19.087500000000002, 19.125, 19.1625, 19.2, 19.2375, 19.275000000000002, 19.3125, 19.35, 19.3875, 19.425, 19.462500000000002, 19.5, 19.5375, 19.575, 19.6125, 19.650000000000002, 19.6875, 19.725, 19.7625, 19.8, 19.837500000000002, 19.875, 19.9125, 19.95, 19.9875, 20.025000000000002, 20.0625, 20.1, 20.1375, 20.175, 20.212500000000002, 20.25, 20.2875, 20.325, 20.3625, 20.400000000000002, 20.4375, 20.475, 20.5125, 20.55, 20.587500000000002, 20.625, 20.6625, 20.7, 20.7375, 20.775000000000002, 20.8125, 20.85, 20.8875, 20.925, 20.962500000000002, 21.0]}, ...(2 in all)]
  in  "background length":i32=25
  out "Correction":cluster{"Y":dbl[], "Y":dbl[]}[](graph)=[{"Y"=[1.0, 1.0, 1.0, 1.0, 1.0, 1.0, 1.0, 1.0, 1.0, 1.0, 1.0, 1.0, 1.0, 1.0, 1.0, 1.0, 1.0, 1.0, 1.0, 1.0, 1.0, 1.0, 1.0, 1.0, 1.0, 1.0, 1.0, 1.0, 1.0, 1.0, 1.0, 1.0, 1.0, 1.0, 1.0, 1.0, 1.0, 1.0, 1.0, 1.0, 1.0, 1.0, 1.0, 1.0, 1.0, 1.0, 1.0, 1.0, 1.0, 1.0, 1.0, 1.0, 1.0, 1.0, 1.0, 1.0, 1.0, 1.0, 1.0, 1.0, 1.0, 1.0, 1.0, 1.0, 1.0, 1.0, 1.0, 1.0, 1.0, 1.0, 1.0, 1.0, 1.0, 1.0, 1.0, 1.0, 1.0, 1.0, 1.0, 1.0, 1.0, 1.0, 1.0, 1.0, 1.0, 1.0, 1.0, 1.0, 1.0, 1.0, 1.0, 1.0, 1.0, 1.0, 1.0, 1.0, 1.0, 1.0, 1.0, 1.0, 1.0, 1.0, 1.0, 1.0, 1.0, 1.0, 1.0, 1.0, 1.0, 1.0, 1.0, 1.0, 1.0, 1.0, 1.0, 1.0, 1.0, 1.0, 1.0, 1.0, 1.0, 1.0, 1.0, 1.0, 1.0, 1.0, 1.0, 1.0, 1.0, 1.0, 1.0, 1.0, 1.0, 1.0, 1.0, 1.0, 1.0, 1.0, 1.0, 1.0, 1.0, 1.0, 1.0, 1.0, 1.0, 1.0, 1.0, 1.0, 1.0, 1.0, 1.0, 1.0, 1.0, 1.0, 1.0, 1.0, 1.0, 1.0, 1.0, 1.0, 1.0, 1.0, 1.0, 1.0, 1.0, 1.0, 1.0, 1.0, 1.0, 1.0, 1.0, 1.0, 1.0, 1.0, 1.0, 1.0, 1.0, 1.0, 1.0, 1.0, 1.0, 1.0, 1.0, 1.0, 1.0, 1.0, 1.0, 1.0, 1.0, 1.0, 1.0, 1.0, 1.0, 1.0, 1.0, 1.0, 1.0, 1.0, 1.0, 1.0, 1.0, 1.0, 1.0, 1.0, 1.0, 1.0, 1.0, 1.0, 1.0, 1.0, 1.0, 1.0, 1.0, 1.0, 1.0, 1.0, 1.0, 1.0, 1.0, 1.0, 1.0, 1.0, 1.0, 1.0, 1.0, 1.0, 1.0, 1.0, 1.0, 1.0, 1.0, 1.0, 1.0, 1.0, 1.0, 1.0, 1.0, 1.0, 1.0, 1.0, 1.0, 1.0, 1.0, 1.0, 1.0, 1.0, 1.0, 1.0, 1.0, 1.0, 1.0, 1.0, 1.0, 1.0, 1.0, 1.0, 1.0, 1.0, 1.0, 1.0, 1.0, 1.0, 1.0, 1.0, 1.0, 1.0, 1.0, 1.0, 1.0, 1.0, 1.0, 1.0, 1.0, 1.0, 1.0, 1.0, 1.0, 1.0, 1.0, 1.0, 1.0, 1.0, 1.0, 1.0, 1.0, 1.0, 1.0, 1.0, 1.0, 1.0, 1.0, 1.0, 1.0, 1.0, 1.0, 1.0, 1.0, 1.0, 1.0, 1.0, 1.0, 1.0, 1.0, 1.0, 1.0, 1.0, 1.0, 1.0, 1.0, 1.0, 1.0, 1.0, 1.0, 1.0, 1.0, 1.0, 1.0, 1.0, 1.0, 1.0, 1.0, 1.0, 1.0, 1.0, 1.0, 1.0, 1.0, 1.0, 1.0, 1.0, 1.0, 1.0, 1.0, 1.0, 1.0, 1.0, 1.0, 1.0, 1.0, 1.0, 1.0, 1.0, 1.0, 1.0, 1.0, 1.0, 1.0, 1.0, 1.0, 1.0, 1.0, 1.0, 1.0, 1.0, 1.0, 1.0, 1.0, 1.0, 1.0, 1.0, 1.0, 1.0, 1.0, 1.0, 1.0, 1.0, 1.0, 1.0, 1.0, 1.0, 1.0, 1.0, 1.0, 1.0, 1.0, 1.0, 1.0, 1.0, 1.0, 1.0, 1.0, 1.0, 1.0, 1.0, 1.0, 1.0, 1.0, 1.0, 1.0, 1.0, 1.0, 1.0, 1.0, 1.0, 1.0, 1.0, 1.0, 1.0, 1.0, 1.0, 1.0, 1.0, 1.0, 1.0, 1.0, 1.0, 1.0, 1.0, 1.0, 1.0, 1.0, 1.0, 1.0, 1.0, 1.0, 1.0, 1.0, 1.0, 1.0, 1.0, 1.0, 1.0, 1.0, 1.0, 1.0, 1.0, 1.0, 1.0, 1.0, 1.0, 1.0, 1.0, 1.0, 1.0, 1.0, 1.0, 1.0, 1.0, 1.0, 1.0, 1.0, 1.0, 1.0, 1.0, 1.0, 1.0, 1.0, 1.0, 1.0, 1.0, 1.0, 1.0, 1.0, 1.0, 1.0, 1.0, 1.0, 1.0, 1.0, 1.0, 1.0, 1.0, 1.0, 1.0, 1.0, 1.0, 1.0, 1.0, 1.0, 1.0, 1.0, 1.0, 1.0, 1.0, 1.0, 1.0, 1.0, 1.0, 1.0, 1.0, 1.0, 1.0, 1.0, 1.0, 1.0, 1.0, 1.0, 1.0, 1.0, 1.0, 1.0, 1.0, 1.0, 1.0, 1.0, 1.0, 1.0, 1.0, 1.0, 1.0, 1.0, 1.0, 1.0, 1.0, 1.0, 1.0, 1.0, 1.0, 1.0, 1.0, 1.0, 1.0, 1.0, 1.0, 1.0, 1.0, 1.0, 1.0, 1.0, 1.0, 1.0, 1.0, 1.0, 1.0, 1.0, 1.0, 1.0, 1.0, 1.0, 1.0, 1.0, 1.0, 1.0, 1.0, 1.0, 1.0, 1.0, 1.0, 1.0, 1.0, 1.0, 1.0, 1.0, 1.0, 1.0, 1.0, 1.0, 1.0, 1.0, 1.0, 1.0, 1.0, 1.0, 1.0, 1.0], "Y"=[0.0375, 0.075, 0.11249999999999999, 0.15, 0.1875, 0.225, 0.26249999999999996, 0.3, 0.33749999999999997, 0.37499999999999994, 0.4125, 0.44999999999999996, 0.48749999999999993, 0.525, 0.5625, 0.6, 0.6375, 0.6749999999999999, 0.7124999999999999, 0.75, 0.7875, 0.825, 0.8624999999999999, 0.8999999999999999, 0.9374999999999999, 0.975, 1.0125, 1.05, 1.0875000000000001, 1.125, 1.1625, 1.2, 1.2375, 1.2750000000000001, 1.3125, 1.35, 1.3875, 1.425, 1.4625000000000001, 1.5, 1.5375, 1.575, 1.6125, 1.6500000000000001, 1.6875, 1.725, 1.7625, 1.8, 1.8375, 1.875, 1.9125, 1.95, 1.9875, 2.025, 2.0625, 2.1, 2.1375, 2.175, 2.2125, 2.25, 2.2875, 2.325, 2.3625, 2.4, 2.4375, 2.475, 2.5125, 2.55, 2.5875, 2.625, 2.6625, 2.7, 2.7375, 2.775, 2.8125, 2.85, 2.8875, 2.925, 2.9625, 3.0, 3.0375, 3.075, 3.1125, 3.15, 3.1875, 3.225, 3.2625, 3.3, 3.3375, 3.375, 3.4125, 3.45, 3.4875, 3.525, 3.5625, 3.6, 3.6374999999999997, 3.675, 3.7125, 3.75, 3.7875, 3.8249999999999997, 3.8625, 3.9, 3.9375, 3.975, 4.012499999999999, 4.05, 4.0874999999999995, 4.124999999999999, 4.1625, 4.199999999999999, 4.2375, 4.2749999999999995, 4.312499999999999, 4.35, 4.387499999999999, 4.425, 4.4624999999999995, 4.499999999999999, 4.5375, 4.574999999999999, 4.6125, 4.6499999999999995, 4.687499999999999, 4.725, 4.762499999999999, 4.8, 4.8374999999999995, 4.874999999999999, 4.9125, 4.949999999999999, 4.9875, 5.0249999999999995, 5.062499999999999, 5.1, 5.137499999999999, 5.175, 5.2124999999999995, 5.249999999999999, 5.2875, 5.324999999999999, 5.3625, 5.3999999999999995, 5.437499999999999, 5.475, 5.512499999999999, 5.55, 5.5874999999999995, 5.624999999999999, 5.6625, 5.699999999999999, 5.7375, 5.7749999999999995, 5.812499999999999, 5.85, 5.887499999999999, 5.925, 5.9624999999999995, 5.999999999999999, 6.0375, 6.074999999999999, 6.1125, 6.1499999999999995, 6.187499999999999, 6.225, 6.262499999999999, 6.3, 6.3374999999999995, 6.374999999999999, 6.4125, 6.449999999999999, 6.4875, 6.5249999999999995, 6.562499999999999, 6.6, 6.637499999999999, 6.675, 6.7124999999999995, 6.749999999999999, 6.7875, 6.824999999999999, 6.8625, 6.8999999999999995, 6.937499999999999, 6.975, 7.012499999999999, 7.05, 7.0874999999999995, 7.124999999999999, 7.1625, 7.199999999999999, 7.237499999999999, 7.2749999999999995, 7.312499999999999, 7.35, 7.387499999999999, 7.424999999999999, 7.4624999999999995, 7.499999999999999, 7.5375, 7.574999999999999, 7.612499999999999, 7.6499999999999995, 7.687499999999999, 7.725, 7.762499999999999, 7.799999999999999, 7.8374999999999995, 7.874999999999999, 7.9125, 7.949999999999999, 7.987499999999999, 8.025, 8.0625, 8.1, 8.1375, 8.174999999999999, 8.212499999999999, 8.25, 8.2875, 8.325, 8.362499999999999, 8.399999999999999, 8.4375, 8.475, 8.5125, 8.549999999999999, 8.587499999999999, 8.625, 8.6625, 8.7, 8.737499999999999, 8.774999999999999, 8.8125, 8.85, 8.8875, 8.924999999999999, 8.962499999999999, 9.0, 9.0375, 9.075, 9.112499999999999, 9.149999999999999, 9.1875, 9.225, 9.2625, 9.299999999999999, 9.337499999999999, 9.375, 9.4125, 9.45, 9.487499999999999, 9.524999999999999, 9.5625, 9.6, 9.6375, 9.674999999999999, 9.712499999999999, 9.75, 9.7875, 9.825, 9.862499999999999, 9.899999999999999, 9.9375, 9.975, 10.0125, 10.049999999999999, 10.087499999999999, 10.125, 10.1625, 10.2, 10.237499999999999, 10.274999999999999, 10.3125, 10.35, 10.3875, 10.424999999999999, 10.462499999999999, 10.5, 10.5375, 10.575, 10.612499999999999, 10.649999999999999, 10.6875, 10.725, 10.7625, 10.799999999999999, 10.837499999999999, 10.875, 10.9125, 10.95, 10.987499999999999, 11.024999999999999, 11.0625, 11.1, 11.1375, 11.174999999999999, 11.212499999999999, 11.25, 11.2875, 11.325, 11.362499999999999, 11.399999999999999, 11.4375, 11.475, 11.5125, 11.549999999999999, 11.587499999999999, 11.625, 11.6625, 11.7, 11.737499999999999, 11.774999999999999, 11.8125, 11.85, 11.8875, 11.924999999999999, 11.962499999999999, 12.0, 12.0375, 12.075, 12.112499999999999, 12.149999999999999, 12.1875, 12.225, 12.2625, 12.299999999999999, 12.337499999999999, 12.375, 12.4125, 12.45, 12.487499999999999, 12.524999999999999, 12.5625, 12.6, 12.6375, 12.674999999999999, 12.712499999999999, 12.75, 12.7875, 12.825, 12.862499999999999, 12.899999999999999, 12.9375, 12.975, 13.0125, 13.049999999999999, 13.087499999999999, 13.125, 13.1625, 13.2, 13.237499999999999, 13.274999999999999, 13.3125, 13.35, 13.3875, 13.424999999999999, 13.462499999999999, 13.5, 13.5375, 13.575, 13.612499999999999, 13.649999999999999, 13.6875, 13.725, 13.7625, 13.799999999999999, 13.837499999999999, 13.875, 13.9125, 13.95, 13.987499999999999, 14.024999999999999, 14.0625, 14.1, 14.1375, 14.174999999999999, 14.212499999999999, 14.25, 14.2875, 14.325, 14.362499999999999, 14.399999999999999, 14.437499999999998, 14.475, 14.5125, 14.549999999999999, 14.587499999999999, 14.624999999999998, 14.6625, 14.7, 14.737499999999999, 14.774999999999999, 14.812499999999998, 14.85, 14.8875, 14.924999999999999, 14.962499999999999, 14.999999999999998, 15.0375, 15.075, 15.112499999999999, 15.149999999999999, 15.187499999999998, 15.225, 15.2625, 15.299999999999999, 15.337499999999999, 15.374999999999998, 15.4125, 15.45, 15.487499999999999, 15.524999999999999, 15.562499999999998, 15.6, 15.6375, 15.674999999999999, 15.712499999999999, 15.749999999999998, 15.7875, 15.825, 15.862499999999999, 15.899999999999999, 15.937499999999998, 15.975, 16.0125, 16.05, 16.087500000000002, 16.125, 16.1625, 16.2, 16.2375, 16.275000000000002, 16.3125, 16.35, 16.3875, 16.425, 16.462500000000002, 16.5, 16.5375, 16.575, 16.6125, 16.650000000000002, 16.6875, 16.725, 16.7625, 16.8, 16.837500000000002, 16.875, 16.9125, 16.95, 16.9875, 17.025000000000002, 17.0625, 17.1, 17.1375, 17.175, 17.212500000000002, 17.25, 17.2875, 17.325, 17.3625, 17.400000000000002, 17.4375, 17.475, 17.5125, 17.55, 17.587500000000002, 17.625, 17.6625, 17.7, 17.7375, 17.775000000000002, 17.8125, 17.85, 17.8875, 17.925, 17.962500000000002, 18.0, 18.0375, 18.075, 18.1125, 18.150000000000002, 18.1875, 18.225, 18.2625, 18.3, 18.337500000000002, 18.375, 18.4125, 18.45, 18.4875, 18.525000000000002, 18.5625, 18.6, 18.6375, 18.675, 18.712500000000002, 18.75, 18.7875, 18.825, 18.8625, 18.900000000000002, 18.9375, 18.975, 19.0125, 19.05, 19.087500000000002, 19.125, 19.1625, 19.2, 19.2375, 19.275000000000002, 19.3125, 19.35, 19.3875, 19.425, 19.462500000000002, 19.5, 19.5375, 19.575, 19.6125, 19.650000000000002, 19.6875, 19.725, 19.7625, 19.8, 19.837500000000002, 19.875, 19.9125, 19.95, 19.9875, 20.025000000000002, 20.0625, 20.1, 20.1375, 20.175, 20.212500000000002, 20.25, 20.2875, 20.325, 20.3625, 20.400000000000002, 20.4375, 20.475, 20.5125, 20.55, 20.587500000000002, 20.625, 20.6625, 20.7, 20.7375, 20.775000000000002, 20.8125, 20.85, 20.8875, 20.925, 20.962500000000002, 21.0]}, ...(2 in all)]
  in  "dead time":dbl=3.7e-08
  out "CH1 RingBuffer long":dbl[][](array[numeric])
  out "CH1 RingBuffer short":dbl[][](array[numeric])
  in  "Weather":T3(tab)
  out "Temperature (C)":dbl(graph)=21.258241758241766
  out "Pressure (mb)":dbl(graph)=838.5851648351648
  out "Relative Humdity (%)":dbl(graph)=16.775030525030523
  out "Pulse Energy (Micro Joule)":T4(graph)
  out "?":cluster{"mean":dbl, "mean":dbl}(graph)={"mean"=0.0, "mean"=2014566.3283164161}
  out "Index":i32=44
  out "CH1 (WV off) smooth L":dbl[](array[numeric])
  out "CH1  Bin Readings":dbl[](array[numeric])
  out "CH1 (WV off) smooth S":dbl[](array[numeric])
  out "CH0 (WV on) smoothed":dbl[](array[numeric])
  out "CH 0 Bin Readings":dbl[](array[numeric])
  out "Range Corrected Altitude Array":dbl[](array[numeric])=[1406.25, 5625.0, 12656.25, 22500.0, 35156.25, 50625.0, 68906.25, 90000.0, 113906.25, 140625.0, 170156.25, 202500.0, 237656.25, 275625.0, 316406.25, 360000.0, 406406.25, 455625.0, 507656.25, 562500.0, 620156.25, 680625.0, 743906.25, 810000.0, 878906.25, 950625.0, 1025156.25, 1102500.0, 1182656.25, 1265625.0, 1351406.25, 1440000.0, 1531406.25, 1625625.0, 1722656.25, 1822500.0, 1925156.25, 2030625.0, 2138906.25, 2250000.0, 2363906.25, 2480625.0, 2600156.25, 2722500.0, 2847656.25, 2975625.0, 3106406.25, 3240000.0, 3376406.25, 3515625.0, 3657656.25, 3802500.0, 3950156.25, 4100625.0, 4253906.25, 4410000.0, 4568906.25, 4730625.0, 4895156.25, 5062500.0, 5232656.25, 5405625.0, 5581406.25, 5760000.0, 5941406.25, 6125625.0, 6312656.25, 6502500.0, 6695156.25, 6890625.0, 7088906.25, 7290000.0, 7493906.25, 7700625.0, 7910156.25, 8122500.0, 8337656.25, 8555625.0, 8776406.25, 9000000.0, 9226406.25, 9455625.0, 9687656.25, 9922500.0, 10160156.25, 10400625.0, 10643906.25, 10890000.0, 11138906.25, 11390625.0, 11645156.25, 11902500.0, 12162656.25, 12425625.0, 12691406.25, 12960000.0, 13231406.25, 13505625.0, 13782656.25, 14062500.0, 14345156.25, 14630625.0, 14918906.25, 15210000.0, 15503906.25, 15800625.0, 16100156.25, 16402500.0, 16707656.25, 17015625.0, 17326406.25, 17640000.0, 17956406.25, 18275625.0, 18597656.25, 18922500.0, 19250156.25, 19580625.0, 19913906.25, 20250000.0, 20588906.25, 20930625.0, 21275156.25, 21622500.0, 21972656.25, 22325625.0, 22681406.25, 23040000.0, 23401406.25, 23765625.0, 24132656.25, 24502500.0, 24875156.25, 25250625.0, 25628906.25, 26010000.0, 26393906.25, 26780625.0, 27170156.25, 27562500.0, 27957656.25, 28355625.0, 28756406.25, 29160000.0, 29566406.25, 29975625.0, 30387656.25, 30802500.0, 31220156.25, 31640625.0, 32063906.25, 32490000.0, 32918906.25, 33350625.0, 33785156.25, 34222500.0, 34662656.25, 35105625.0, 35551406.25, 36000000.0, 36451406.25, 36905625.0, 37362656.25, 37822500.0, 38285156.25, 38750625.0, 39218906.25, 39690000.0, 40163906.25, 40640625.0, 41120156.25, 41602500.0, 42087656.25, 42575625.0, 43066406.25, 43560000.0, 44056406.25, 44555625.0, 45057656.25, 45562500.0, 46070156.25, 46580625.0, 47093906.25, 47610000.0, 48128906.25, 48650625.0, 49175156.25, 49702500.0, 50232656.25, 50765625.0, 51301406.25, 51840000.0, 52381406.25, 52925625.0, 53472656.25, 54022500.0, 54575156.25, 55130625.0, 55688906.25, 56250000.0, 56813906.25, 57380625.0, 57950156.25, 58522500.0, 59097656.25, 59675625.0, 60256406.25, 60840000.0, 61426406.25, 62015625.0, 62607656.25, 63202500.0, 63800156.25, 64400625.0, 65003906.25, 65610000.0, 66218906.25, 66830625.0, 67445156.25, 68062500.0, 68682656.25, 69305625.0, 69931406.25, 70560000.0, 71191406.25, 71825625.0, 72462656.25, 73102500.0, 73745156.25, 74390625.0, 75038906.25, 75690000.0, 76343906.25, 77000625.0, 77660156.25, 78322500.0, 78987656.25, 79655625.0, 80326406.25, 81000000.0, 81676406.25, 82355625.0, 83037656.25, 83722500.0, 84410156.25, 85100625.0, 85793906.25, 86490000.0, 87188906.25, 87890625.0, 88595156.25, 89302500.0, 90012656.25, 90725625.0, 91441406.25, 92160000.0, 92881406.25, 93605625.0, 94332656.25, 95062500.0, 95795156.25, 96530625.0, 97268906.25, 98010000.0, 98753906.25, 99500625.0, 100250156.25, 101002500.0, 101757656.25, 102515625.0, 103276406.25, 104040000.0, 104806406.25, 105575625.0, 106347656.25, 107122500.0, 107900156.25, 108680625.0, 109463906.25, 110250000.0, 111038906.25, 111830625.0, 112625156.25, 113422500.0, 114222656.25, 115025625.0, 115831406.25, 116640000.0, 117451406.25, 118265625.0, 119082656.25, 119902500.0, 120725156.25, 121550625.0, 122378906.25, 123210000.0, 124043906.25, 124880625.0, 125720156.25, 126562500.0, 127407656.25, 128255625.0, 129106406.25, 129960000.0, 130816406.25, 131675625.0, 132537656.25, 133402500.0, 134270156.25, 135140625.0, 136013906.25, 136890000.0, 137768906.25, 138650625.0, 139535156.25, 140422500.0, 141312656.25, 142205625.0, 143101406.25, 144000000.0, 144901406.25, 145805625.0, 146712656.25, 147622500.0, 148535156.25, 149450625.0, 150368906.25, 151290000.0, 152213906.25, 153140625.0, 154070156.25, 155002500.0, 155937656.25, 156875625.0, 157816406.25, 158760000.0, 159706406.25, 160655625.0, 161607656.25, 162562500.0, 163520156.25, 164480625.0, 165443906.25, 166410000.0, 167378906.25, 168350625.0, 169325156.25, 170302500.0, 171282656.25, 172265625.0, 173251406.25, 174240000.0, 175231406.25, 176225625.0, 177222656.25, 178222500.0, 179225156.25, 180230625.0, 181238906.25, 182250000.0, 183263906.25, 184280625.0, 185300156.25, 186322500.0, 187347656.25, 188375625.0, 189406406.25, 190440000.0, 191476406.25, 192515625.0, 193557656.25, 194602500.0, 195650156.25, 196700625.0, 197753906.25, 198810000.0, 199868906.25, 200930625.0, 201995156.25, 203062500.0, 204132656.25, 205205625.0, 206281406.25, 207360000.0, 208441406.25, 209525625.0, 210612656.25, 211702500.0, 212795156.25, 213890625.0, 214988906.25, 216090000.0, 217193906.25, 218300625.0, 219410156.25, 220522500.0, 221637656.25, 222755625.0, 223876406.25, 225000000.0, 226126406.25, 227255625.0, 228387656.25, 229522500.0, 230660156.25, 231800625.0, 232943906.25, 234090000.0, 235238906.25, 236390625.0, 237545156.25, 238702500.0, 239862656.25, 241025625.0, 242191406.25, 243360000.0, 244531406.25, 245705625.0, 246882656.25, 248062500.0, 249245156.25, 250430625.0, 251618906.25, 252810000.0, 254003906.25, 255200625.0, 256400156.25, 257602500.0, 258807656.25, 260015625.0, 261226406.25, 262440000.0, 263656406.25, 264875625.0, 266097656.25, 267322500.0, 268550156.25, 269780625.0, 271013906.25, 272250000.0, 273488906.25, 274730625.0, 275975156.25, 277222500.0, 278472656.25, 279725625.0, 280981406.25, 282240000.0, 283501406.25, 284765625.0, 286032656.25, 287302500.0, 288575156.25, 289850625.0, 291128906.25, 292410000.0, 293693906.25, 294980625.0, 296270156.25, 297562500.0, 298857656.25, 300155625.0, 301456406.25, 302760000.0, 304066406.25, 305375625.0, 306687656.25, 308002500.0, 309320156.25, 310640625.0, 311963906.25, 313290000.0, 314618906.25, 315950625.0, 317285156.25, 318622500.0, 319962656.25, 321305625.0, 322651406.25, 324000000.0, 325351406.25, 326705625.0, 328062656.25, 329422500.0, 330785156.25, 332150625.0, 333518906.25, 334890000.0, 336263906.25, 337640625.0, 339020156.25, 340402500.0, 341787656.25, 343175625.0, 344566406.25, 345960000.0, 347356406.25, 348755625.0, 350157656.25, 351562500.0, 352970156.25, 354380625.0, 355793906.25, 357210000.0, 358628906.25, 360050625.0, 361475156.25, 362902500.0, 364332656.25, 365765625.0, 367201406.25, 368640000.0, 370081406.25, 371525625.0, 372972656.25, 374422500.0, 375875156.25, 377330625.0, 378788906.25, 380250000.0, 381713906.25, 383180625.0, 384650156.25, 386122500.0, 387597656.25, 389075625.0, 390556406.25, 392040000.0, 393526406.25, 395015625.0, 396507656.25, 398002500.0, 399500156.25, 401000625.0, 402503906.25, 404010000.0, 405518906.25, 407030625.0, 408545156.25, 410062500.0, 411582656.25, 413105625.0, 414631406.25, 416160000.0, 417691406.25, 419225625.0, 420762656.25, 422302500.0, 423845156.25, 425390625.0, 426938906.25, 428490000.0, 430043906.25, 431600625.0, 433160156.25, 434722500.0, 436287656.25, 437855625.0, 439426406.25, 441000000.0]
  out "Altitude Array (km)":dbl[](array[numeric])=[0.0375, 0.075, 0.11249999999999999, 0.15, 0.1875, 0.225, 0.26249999999999996, 0.3, 0.33749999999999997, 0.37499999999999994, 0.4125, 0.44999999999999996, 0.48749999999999993, 0.525, 0.5625, 0.6, 0.6375, 0.6749999999999999, 0.7124999999999999, 0.75, 0.7875, 0.825, 0.8624999999999999, 0.8999999999999999, 0.9374999999999999, 0.975, 1.0125, 1.05, 1.0875000000000001, 1.125, 1.1625, 1.2, 1.2375, 1.2750000000000001, 1.3125, 1.35, 1.3875, 1.425, 1.4625000000000001, 1.5, 1.5375, 1.575, 1.6125, 1.6500000000000001, 1.6875, 1.725, 1.7625, 1.8, 1.8375, 1.875, 1.9125, 1.95, 1.9875, 2.025, 2.0625, 2.1, 2.1375, 2.175, 2.2125, 2.25, 2.2875, 2.325, 2.3625, 2.4, 2.4375, 2.475, 2.5125, 2.55, 2.5875, 2.625, 2.6625, 2.7, 2.7375, 2.775, 2.8125, 2.85, 2.8875, 2.925, 2.9625, 3.0, 3.0375, 3.075, 3.1125, 3.15, 3.1875, 3.225, 3.2625, 3.3, 3.3375, 3.375, 3.4125, 3.45, 3.4875, 3.525, 3.5625, 3.6, 3.6374999999999997, 3.675, 3.7125, 3.75, 3.7875, 3.8249999999999997, 3.8625, 3.9, 3.9375, 3.975, 4.012499999999999, 4.05, 4.0874999999999995, 4.124999999999999, 4.1625, 4.199999999999999, 4.2375, 4.2749999999999995, 4.312499999999999, 4.35, 4.387499999999999, 4.425, 4.4624999999999995, 4.499999999999999, 4.5375, 4.574999999999999, 4.6125, 4.6499999999999995, 4.687499999999999, 4.725, 4.762499999999999, 4.8, 4.8374999999999995, 4.874999999999999, 4.9125, 4.949999999999999, 4.9875, 5.0249999999999995, 5.062499999999999, 5.1, 5.137499999999999, 5.175, 5.2124999999999995, 5.249999999999999, 5.2875, 5.324999999999999, 5.3625, 5.3999999999999995, 5.437499999999999, 5.475, 5.512499999999999, 5.55, 5.5874999999999995, 5.624999999999999, 5.6625, 5.699999999999999, 5.7375, 5.7749999999999995, 5.812499999999999, 5.85, 5.887499999999999, 5.925, 5.9624999999999995, 5.999999999999999, 6.0375, 6.074999999999999, 6.1125, 6.1499999999999995, 6.187499999999999, 6.225, 6.262499999999999, 6.3, 6.3374999999999995, 6.374999999999999, 6.4125, 6.449999999999999, 6.4875, 6.5249999999999995, 6.562499999999999, 6.6, 6.637499999999999, 6.675, 6.7124999999999995, 6.749999999999999, 6.7875, 6.824999999999999, 6.8625, 6.8999999999999995, 6.937499999999999, 6.975, 7.012499999999999, 7.05, 7.0874999999999995, 7.124999999999999, 7.1625, 7.199999999999999, 7.237499999999999, 7.2749999999999995, 7.312499999999999, 7.35, 7.387499999999999, 7.424999999999999, 7.4624999999999995, 7.499999999999999, 7.5375, 7.574999999999999, 7.612499999999999, 7.6499999999999995, 7.687499999999999, 7.725, 7.762499999999999, 7.799999999999999, 7.8374999999999995, 7.874999999999999, 7.9125, 7.949999999999999, 7.987499999999999, 8.025, 8.0625, 8.1, 8.1375, 8.174999999999999, 8.212499999999999, 8.25, 8.2875, 8.325, 8.362499999999999, 8.399999999999999, 8.4375, 8.475, 8.5125, 8.549999999999999, 8.587499999999999, 8.625, 8.6625, 8.7, 8.737499999999999, 8.774999999999999, 8.8125, 8.85, 8.8875, 8.924999999999999, 8.962499999999999, 9.0, 9.0375, 9.075, 9.112499999999999, 9.149999999999999, 9.1875, 9.225, 9.2625, 9.299999999999999, 9.337499999999999, 9.375, 9.4125, 9.45, 9.487499999999999, 9.524999999999999, 9.5625, 9.6, 9.6375, 9.674999999999999, 9.712499999999999, 9.75, 9.7875, 9.825, 9.862499999999999, 9.899999999999999, 9.9375, 9.975, 10.0125, 10.049999999999999, 10.087499999999999, 10.125, 10.1625, 10.2, 10.237499999999999, 10.274999999999999, 10.3125, 10.35, 10.3875, 10.424999999999999, 10.462499999999999, 10.5, 10.5375, 10.575, 10.612499999999999, 10.649999999999999, 10.6875, 10.725, 10.7625, 10.799999999999999, 10.837499999999999, 10.875, 10.9125, 10.95, 10.987499999999999, 11.024999999999999, 11.0625, 11.1, 11.1375, 11.174999999999999, 11.212499999999999, 11.25, 11.2875, 11.325, 11.362499999999999, 11.399999999999999, 11.4375, 11.475, 11.5125, 11.549999999999999, 11.587499999999999, 11.625, 11.6625, 11.7, 11.737499999999999, 11.774999999999999, 11.8125, 11.85, 11.8875, 11.924999999999999, 11.962499999999999, 12.0, 12.0375, 12.075, 12.112499999999999, 12.149999999999999, 12.1875, 12.225, 12.2625, 12.299999999999999, 12.337499999999999, 12.375, 12.4125, 12.45, 12.487499999999999, 12.524999999999999, 12.5625, 12.6, 12.6375, 12.674999999999999, 12.712499999999999, 12.75, 12.7875, 12.825, 12.862499999999999, 12.899999999999999, 12.9375, 12.975, 13.0125, 13.049999999999999, 13.087499999999999, 13.125, 13.1625, 13.2, 13.237499999999999, 13.274999999999999, 13.3125, 13.35, 13.3875, 13.424999999999999, 13.462499999999999, 13.5, 13.5375, 13.575, 13.612499999999999, 13.649999999999999, 13.6875, 13.725, 13.7625, 13.799999999999999, 13.837499999999999, 13.875, 13.9125, 13.95, 13.987499999999999, 14.024999999999999, 14.0625, 14.1, 14.1375, 14.174999999999999, 14.212499999999999, 14.25, 14.2875, 14.325, 14.362499999999999, 14.399999999999999, 14.437499999999998, 14.475, 14.5125, 14.549999999999999, 14.587499999999999, 14.624999999999998, 14.6625, 14.7, 14.737499999999999, 14.774999999999999, 14.812499999999998, 14.85, 14.8875, 14.924999999999999, 14.962499999999999, 14.999999999999998, 15.0375, 15.075, 15.112499999999999, 15.149999999999999, 15.187499999999998, 15.225, 15.2625, 15.299999999999999, 15.337499999999999, 15.374999999999998, 15.4125, 15.45, 15.487499999999999, 15.524999999999999, 15.562499999999998, 15.6, 15.6375, 15.674999999999999, 15.712499999999999, 15.749999999999998, 15.7875, 15.825, 15.862499999999999, 15.899999999999999, 15.937499999999998, 15.975, 16.0125, 16.05, 16.087500000000002, 16.125, 16.1625, 16.2, 16.2375, 16.275000000000002, 16.3125, 16.35, 16.3875, 16.425, 16.462500000000002, 16.5, 16.5375, 16.575, 16.6125, 16.650000000000002, 16.6875, 16.725, 16.7625, 16.8, 16.837500000000002, 16.875, 16.9125, 16.95, 16.9875, 17.025000000000002, 17.0625, 17.1, 17.1375, 17.175, 17.212500000000002, 17.25, 17.2875, 17.325, 17.3625, 17.400000000000002, 17.4375, 17.475, 17.5125, 17.55, 17.587500000000002, 17.625, 17.6625, 17.7, 17.7375, 17.775000000000002, 17.8125, 17.85, 17.8875, 17.925, 17.962500000000002, 18.0, 18.0375, 18.075, 18.1125, 18.150000000000002, 18.1875, 18.225, 18.2625, 18.3, 18.337500000000002, 18.375, 18.4125, 18.45, 18.4875, 18.525000000000002, 18.5625, 18.6, 18.6375, 18.675, 18.712500000000002, 18.75, 18.7875, 18.825, 18.8625, 18.900000000000002, 18.9375, 18.975, 19.0125, 19.05, 19.087500000000002, 19.125, 19.1625, 19.2, 19.2375, 19.275000000000002, 19.3125, 19.35, 19.3875, 19.425, 19.462500000000002, 19.5, 19.5375, 19.575, 19.6125, 19.650000000000002, 19.6875, 19.725, 19.7625, 19.8, 19.837500000000002, 19.875, 19.9125, 19.95, 19.9875, 20.025000000000002, 20.0625, 20.1, 20.1375, 20.175, 20.212500000000002, 20.25, 20.2875, 20.325, 20.3625, 20.400000000000002, 20.4375, 20.475, 20.5125, 20.55, 20.587500000000002, 20.625, 20.6625, 20.7, 20.7375, 20.775000000000002, 20.8125, 20.85, 20.8875, 20.925, 20.962500000000002, 21.0]
  out "Offline Pulse Energy":dbl
  out "Online Pulse Energy":dbl
  in  "Instrument Control":T5(tab)
  in  "Device In":refnum<visa-resource-name>="Pro8000"
  in  "Settings":T6={"Module"=enum."WV Online TEC", "WV Online TEC"=14.209649999999913, "WV Online LD"=0.16, "WV Offline TEC"=29.53825, "WV Offline LD"=0.16, "WV Etalon TEC"=30.0, "HSRL Etalon TEC"=18.9999638, "HSRL TEC"=14.172, "HSRL LD"=0.16} {"HSRL LD" min=0.0 max=0.18 step=0.001 format="%.3p"; "HSRL TEC" min=14.0 max=28.0 step=0.1 format="%.3g"; "WV Offline LD" min=0.0 max=0.18 step=0.001 format="%.3p"; "WV Online LD" min=0.0 max=0.18 step=0.001 format="%.3p"; "HSRL Etalon TEC" format="%.2g"; "WV Etalon TEC" format="%.2g"; "WV Offline TEC" min=16.0 max=30.0 step=0.1 format="%.3g"; "WV Online TEC" min=14.0 max=28.0 step=0.1 format="%.3g"}
  out "Readings":T7={"Pro8000"=TRUE, "WV OnLine TEC"=14.2108402, "WV Online TEC"=TRUE, "WV Online LD"=0.160613284, "WV Online LD"=TRUE, "WV Offline TEC"=23.042078, "WV Offline TEC"=FALSE, "WV Offline LD"=0.000177734386, "WV Offline LD"=FALSE, "WV EtalonTEC"=30.0244102, "WV Etalon TEC"=TRUE, "HSRL Etalon TEC"=9.51464272, "HSRL Etalon TEC"=FALSE, "HSRL TEC"=-12.375, "HSRL TEC "=FALSE, "HSRL LD"=0.0, "HSRL LD"=FALSE} {"HSRL LD" format="%.3p"; "HSRL TEC" format="%.3g"; "WV Offline LD" format="%.3p"; "WV Online LD" format="%.3p"; "HSRL Etalon TEC" format="%.3g"; "WV EtalonTEC" format="%.3g"; "WV Offline TEC" format="%.3g"; "WV OnLine TEC" format="%.3g"}
  in  "Pulse B Polarity":enum32{"Low", "High"}(ring)=enum."High"
  in  "Pulse A Delay(ns)":u32=1040 min=80 max=327600
  in  "Pulse B Delay(ns)":u32=170000 min=80 max=327600 step=1
  in  "Accumulation Delay(ns)":u32=10 min=10 max=1270 step=1
  in  "Sync Pulse Polarity":enum32{"Low", "High"}(ring)=enum."High"
  in  "Pulse A Polarity":enum32{"Low", "High"}(ring)=enum."High"
  in  "Number of Bins":u32=560 min=2 max=4095 step=1
  in  "Number of Accumulates":u32=14285 min=1 max=32767 step=1
  in  "Time Resolution Per Bin(ns)":u32=250 min=5 max=1063 step=1
  out "AMCS_Profile":i32=481
  in  "WV Online Set (nm)":dbl=780.24612 format="%.5f"
  out "WV Online Read (nm)":dbl=780.246142655685 format="%.5f"
  out "WV Offline Read (nm)":dbl=780.2460604321718 format="%.5f"
  in  "WV Offline Set (nm)":dbl=780.24612 format="%#.5f"
  in  "Bristol In":i32=5
  out "Bristol Out":i32
  out "WL_Difference":dbl=2.2655685029349115e-05 format="%#_3e"
  out "WL Difference off":dbl=-5.956782820248918e-05 format="%#_3e"
  out "Wavelength Lock Online":bool=TRUE
  out "Wavelength Lock Offline":bool=TRUE
  in  "calculate absorption cross sections":bool
  in  "Online_Tol":dbl=5e-05 format="%#_15g"
  in  "Cancel online":bool
  in  "Offline_Tol":dbl=0.001 format="%#_15g"
  in  "Cancel Offline":bool
  in  "y":dbl=0.00025 format="%#_6p"
  in  "Smoothing Range":dbl=150.0
  in  "Total DIAL Integration Time (Minutes)":i32=3
  in  "Data Reads (number of loops)":i32=1
  in  "Total Aerosol Integration Time (Minutes)":dbl=0.5
  in  "Scalar Wait Time":u32
  out "Smoothed Bins":dbl=4.0
  in  "NewportIn":string
  in  "logging":bool
  out "Newport Device Key":string
  in  "SampleSize":i32=2
  out "NewportRef":refnum<k24>
  in  "Switch Comm Port":refnum<visa-resource-name>="COM3"
  out "FF_On_Ref":refnum<file>
  out "FF_On_Ptr":i64=208288 format="%.2p"
  out "FF_Off_Ref":refnum<file>
  out "FF_Off_Ptr":i64=199232 format="%.2p"
  out "NF_On_Ref":refnum<file>
  out "NF_On_Ptr":i64=208288 format="%.2p"
  out "NF_Off_Ref":refnum<file>
  out "NF_Off_Ptr":i64=199232 format="%.2p"
  out "DataOpen":bool=TRUE
  out "File Path_Far Field (out)":string="C:\\Users\\H2ODial\\Desktop\\SharedTeleWVData\\170314FF\\20"
  out "File Path_Near Field (out)":string="C:\\Users\\H2ODial\\Desktop\\SharedTeleWVData\\170314NF\\20"
  in  "Data File DIR (in)":string="C:\\Users\\H2ODial\\Desktop\\SharedTeleWVData\\"
  out "TRHP":T8={"Temp C"=21.258241758241766, "RelH %"=16.775030525030523, "Press hPa"=838.5851648351648, "AbH g/m^3"=3.0830280830280827}
  in  "WS visa":refnum<visa-resource-name>="LuftWS"
  in  "WS_On/Off":bool=TRUE
  in  "bins":u32=560 min=2 max=4095 step=1
  out "y offset":u32=10
  in  "ns scale":u32=250
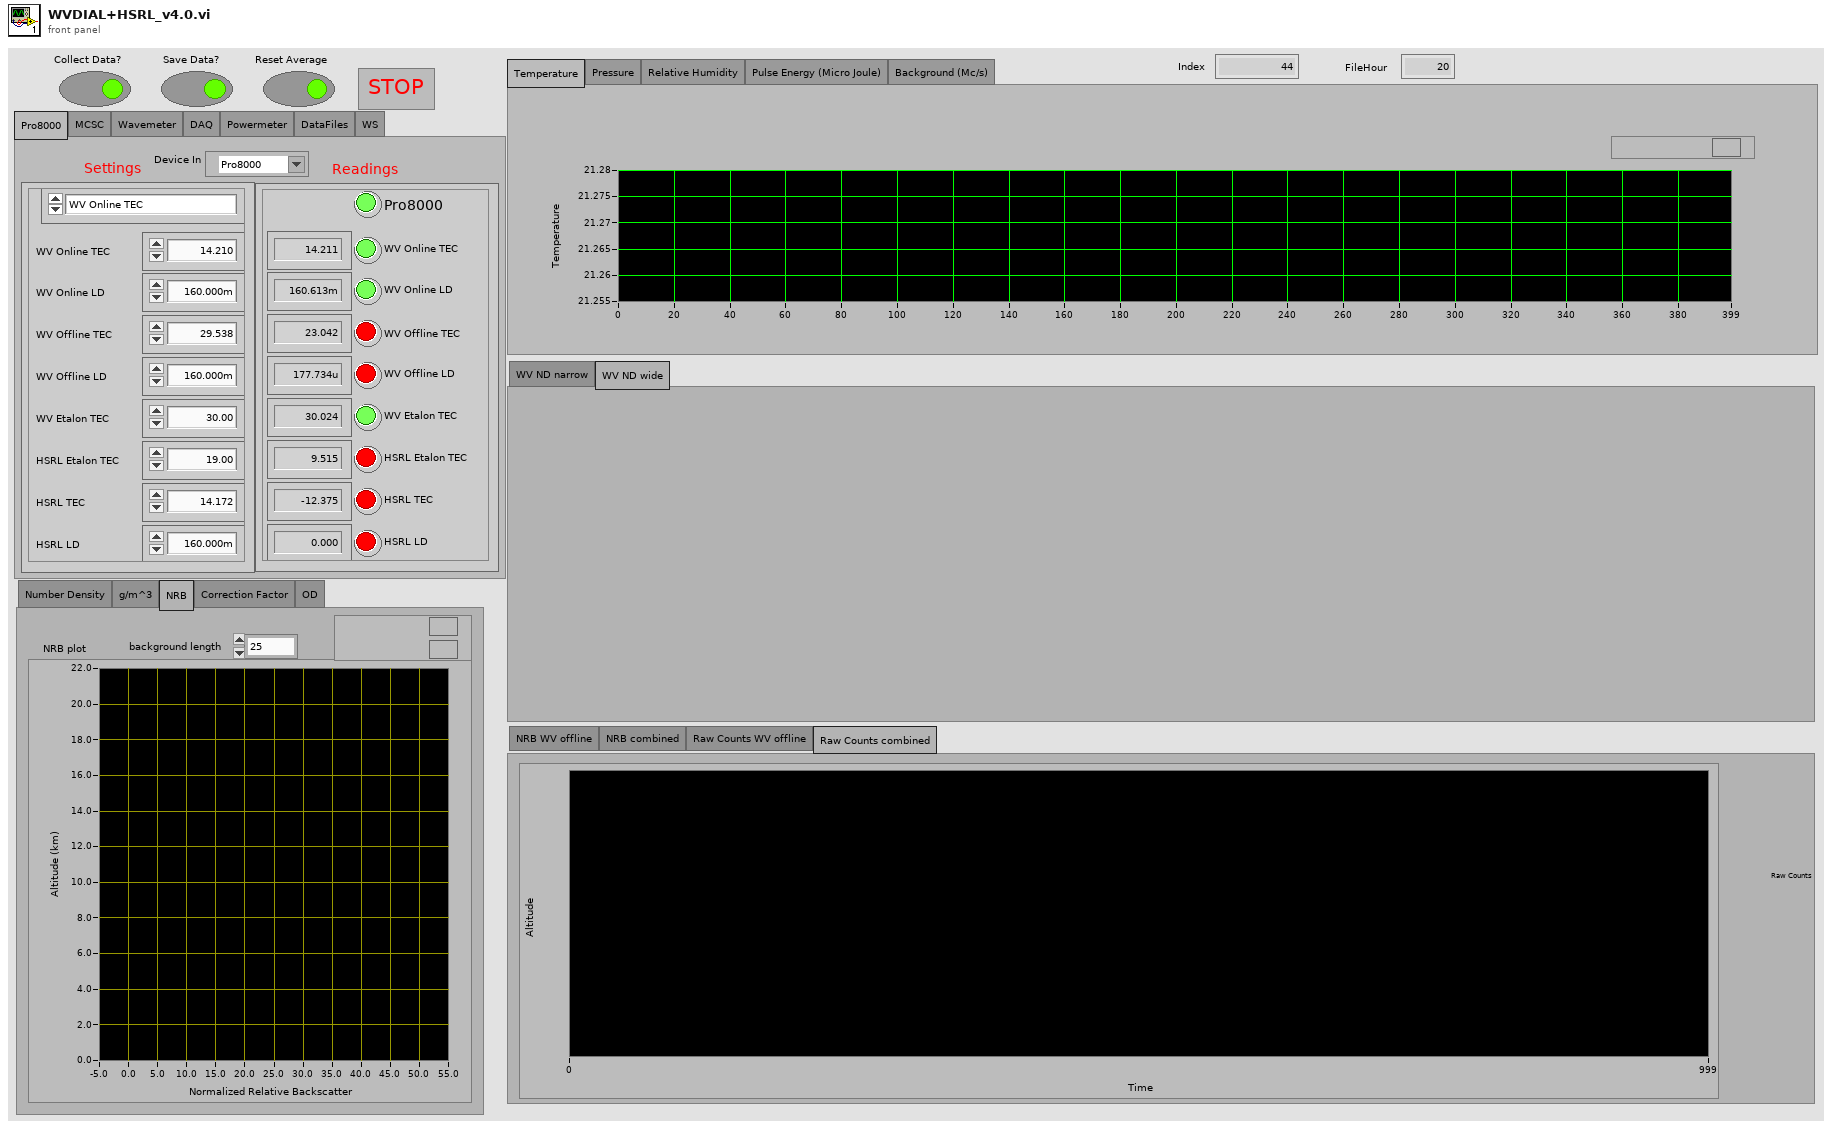
[diagram p1: front panel]
types:
  T1 = enum32{"NRB WV offline", "NRB combined", "Raw Counts WV offline", "Raw Counts combined"}
  T2 = enum32{"Number Density", "g/m^3", "NRB", "Correction Factor", "OD"}
  T3 = enum32{"Temperature", "Pressure", "Relative Humidity", "Pulse Energy (Micro Joule)", "Background (Mc/s)"}
  T4 = cluster{"Online Pulse Energy":dbl, "Pulse Energy Offline":dbl}
  T5 = enum32{"Pro8000", "MCSC", "Wavemeter", "DAQ", "Powermeter", "DataFiles", "WS"}
  T6 = cluster{"Module":enum16{"WV Online TEC", "WV Online LD", "WV Offline TEC", "WV Offline LD", "WV Etalon TEC", "HSRL Etalon TEC", "HSRL TEC", "HSRL LD"}, "WV Online TEC":dbl, "WV Online LD":dbl, "WV Offline TEC":dbl, "WV Offline LD":dbl, "WV Etalon TEC":dbl, "HSRL Etalon TEC":dbl, "HSRL TEC":dbl, "HSRL LD":dbl}
  T7 = cluster{"Pro8000":bool, "WV OnLine TEC":dbl, "WV Online TEC":bool, "WV Online LD":dbl, "WV Online LD":bool, "WV Offline TEC":dbl, "WV Offline TEC":bool, "WV Offline LD":dbl, "WV Offline LD":bool, "WV EtalonTEC":dbl, "WV Etalon TEC":bool, "HSRL Etalon TEC":dbl, "HSRL Etalon TEC":bool, "HSRL TEC":dbl, "HSRL TEC ":bool, "HSRL LD":dbl, "HSRL LD":bool}
  T8 = cluster{"Temp C":dbl, "RelH %":dbl, "Press hPa":dbl, "AbH g/m^3":dbl}
  T9 = enum16{"Open_TL", "Close_TL", "Verify_ID", "TEC_Sensor", "SET", "READ", "ON", "OFF", "Set_Limits", "Read_Limits", "Enable_Status", "Read_Status"}
  T10 = enum16{"Initialize ILX", "Set ON T", "Set Off T", "Set ON I", "Set Off I", "Set On Lim", "Set Off Lim", "Read ILX", "TEC ON/OFF", "LASER ON/OFF", "Status?", "ILX OFF"}
  T11 = enum16{"open", "replace", "create", "open or create", "replace or create", "replace or create with confirmation"}
  T12 = enum16{"WV Online TEC", "WV Online LD", "WV Offline TEC", "WV Offline LD", "WV Etalon TEC", "HSRL Etalon TEC", "HSRL TEC", "HSRL LD"}
  T13 = cluster{"Temp":dbl, "RelH":dbl, "Press":dbl, "AbH":dbl}
  T14 = typedef "LVDateTimeRec.ctl" = cluster{"fractional second":dbl, "second":i32, "minute":i32, "hour":i32, "day of month":i32, "month":i32, "year":i32, "day of week":i32, "day of year":i32, "DST":i32}
  T15 = cluster{"Online Pulse Energy":dbl, "Offline Pulse Energy":dbl}
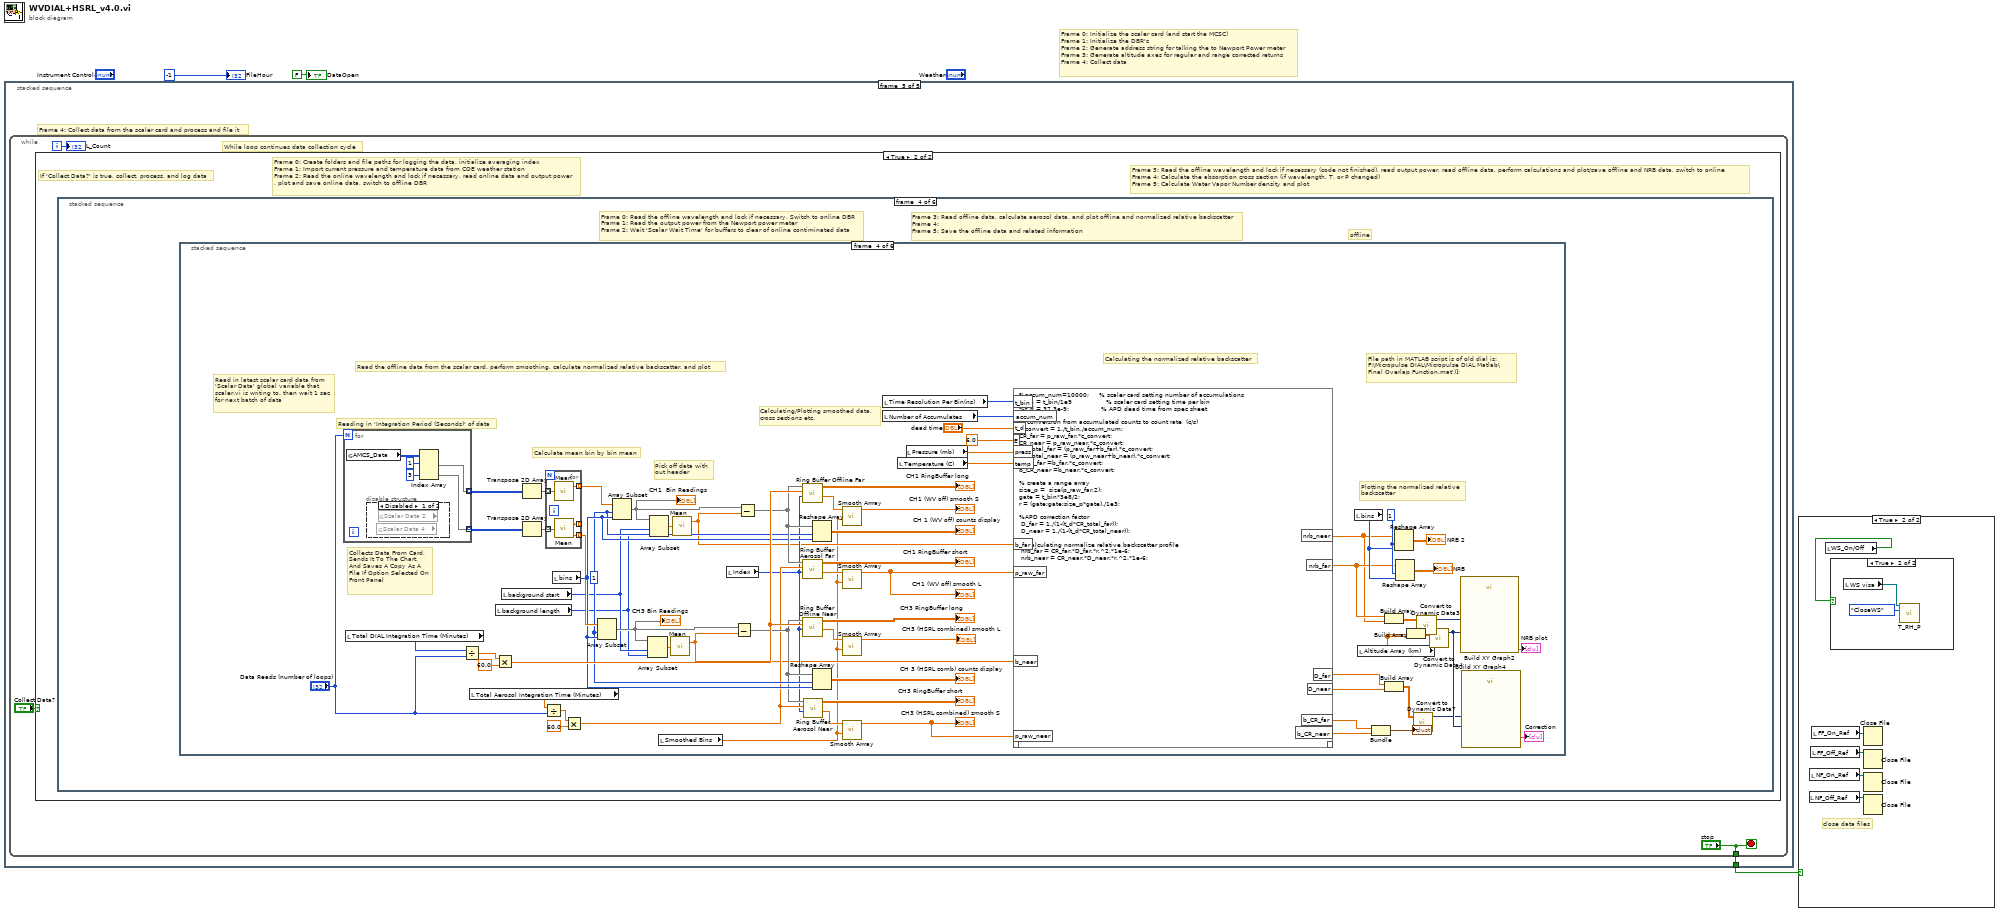
[diagram p0: block diagram]
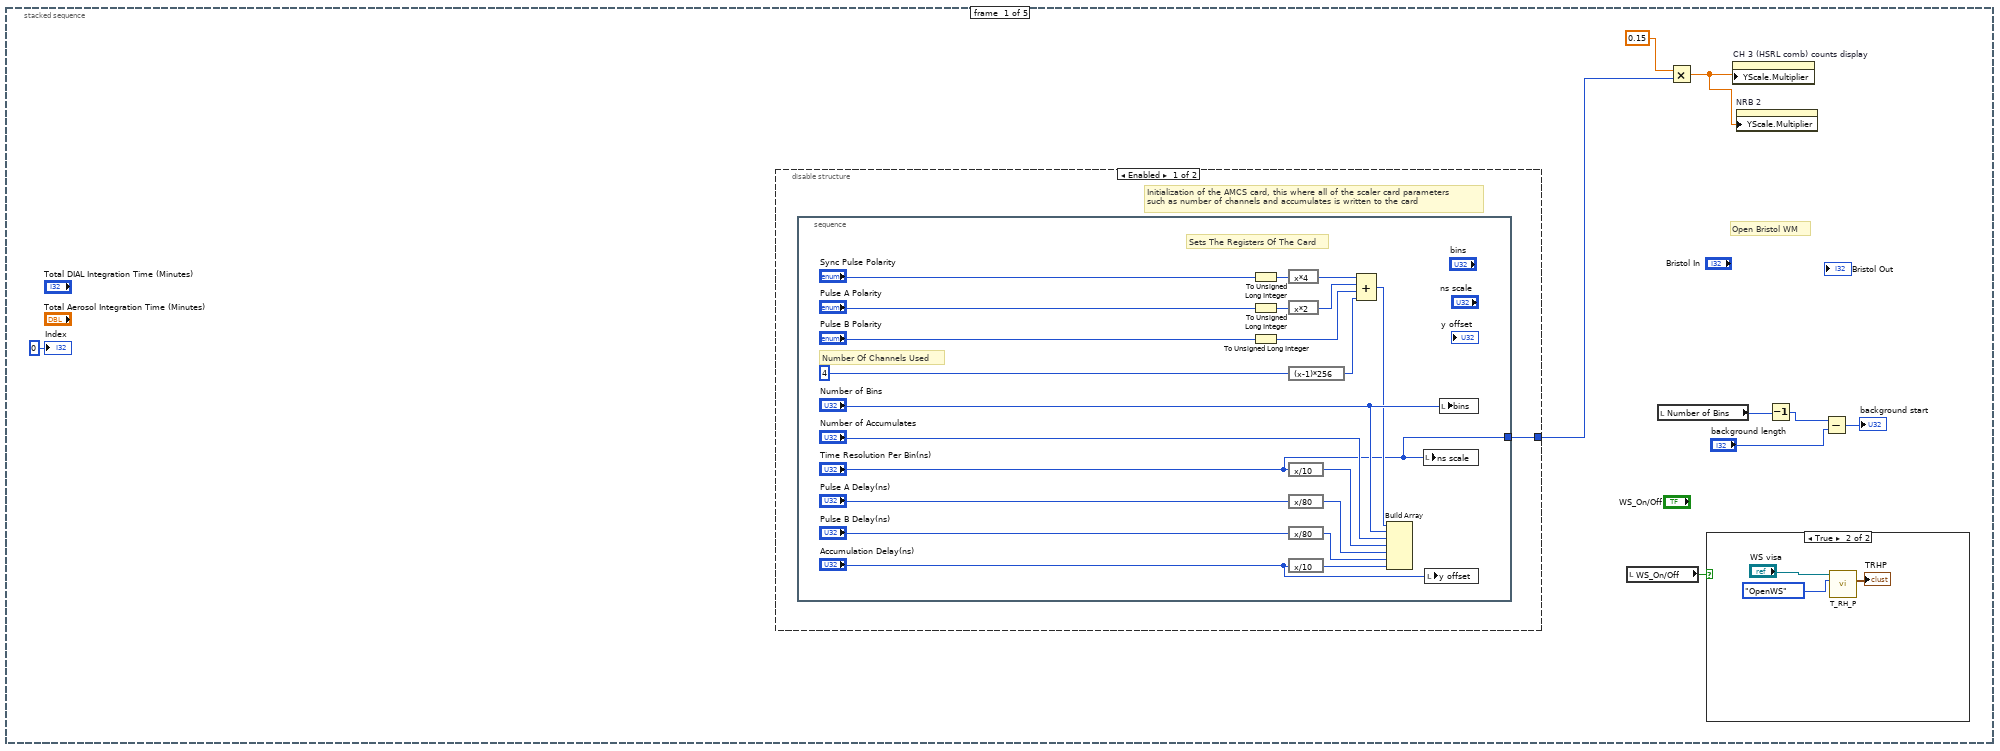
[diagram p4: hidden frame]
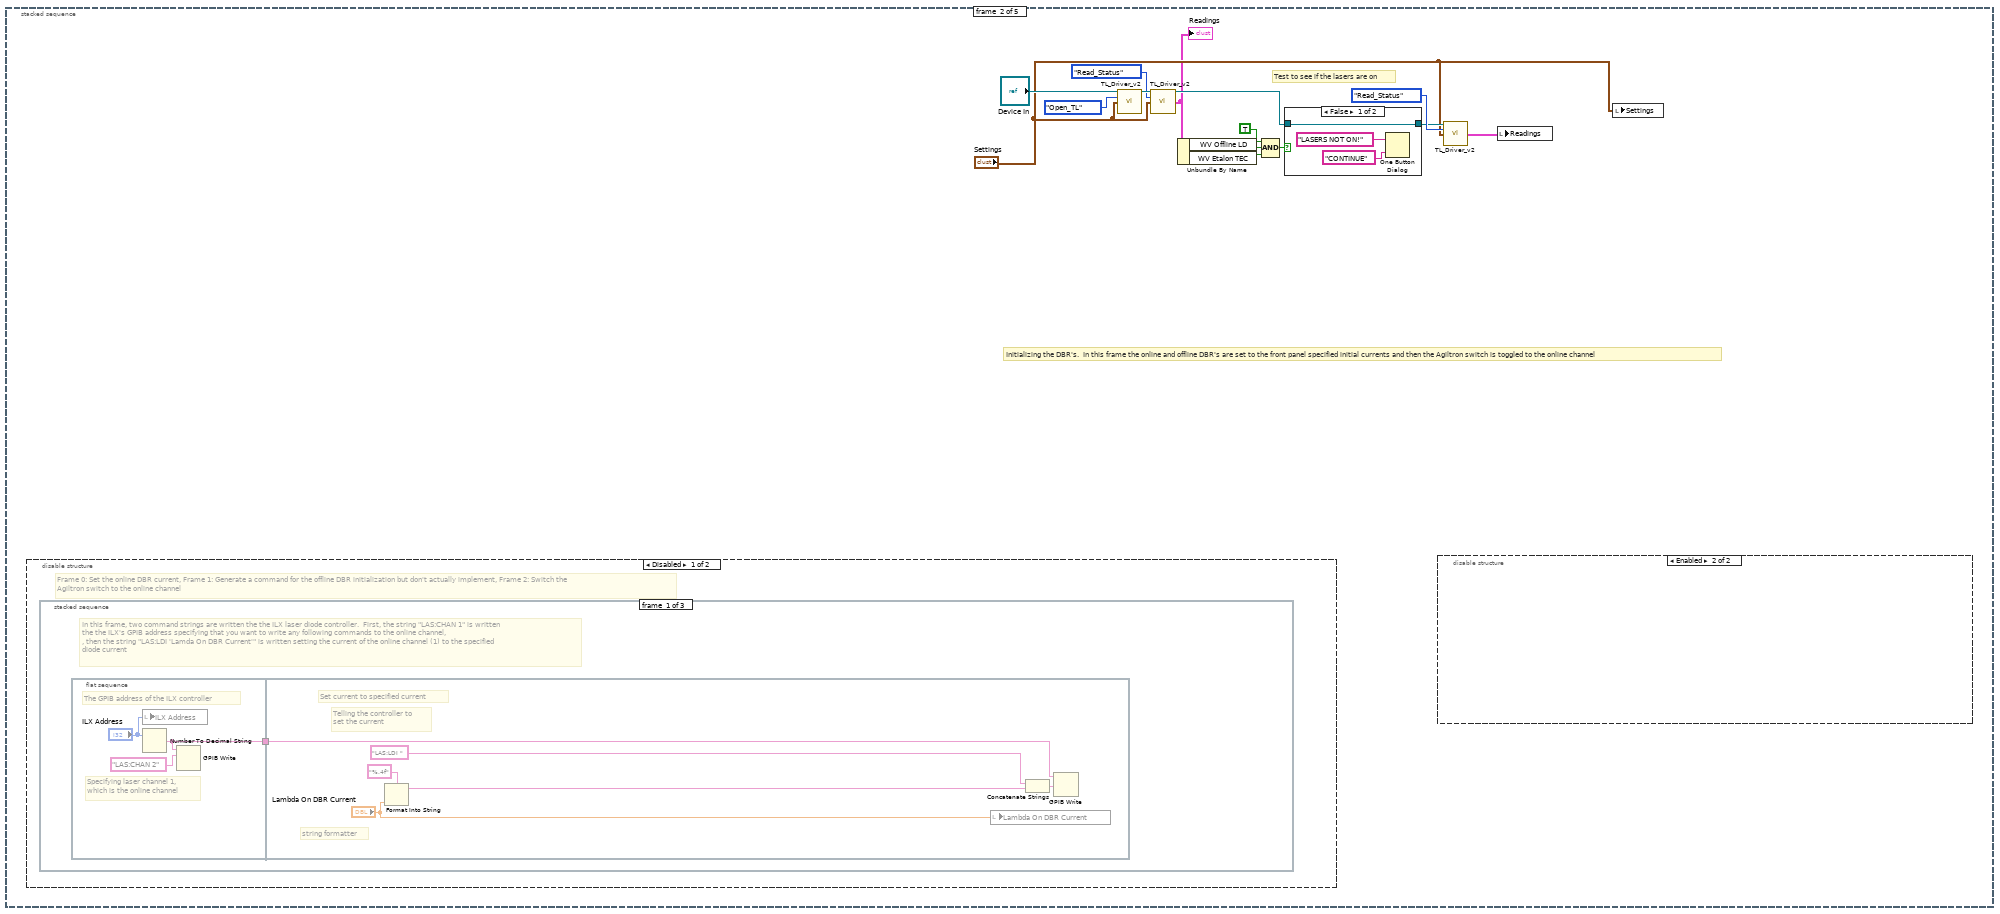
[diagram p7: hidden frame]
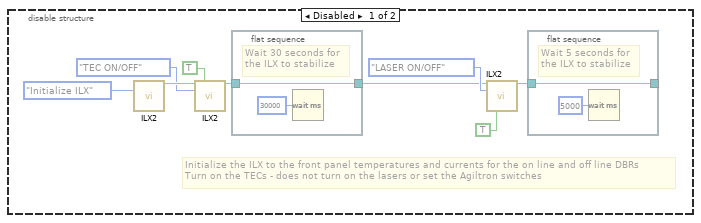
[diagram p9: hidden frame]
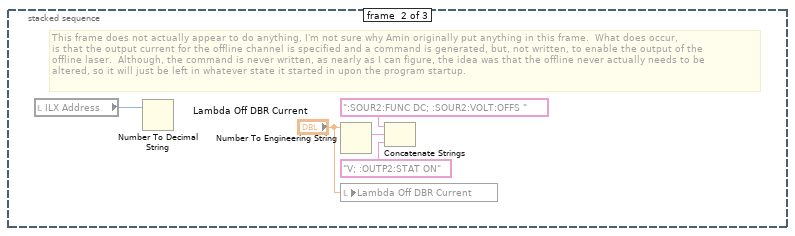
[diagram p10: hidden frame]
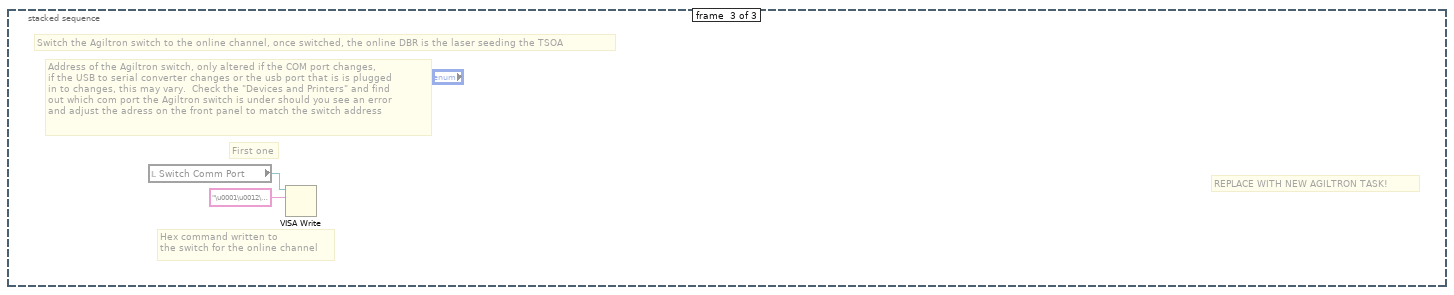
[diagram p11: hidden frame]
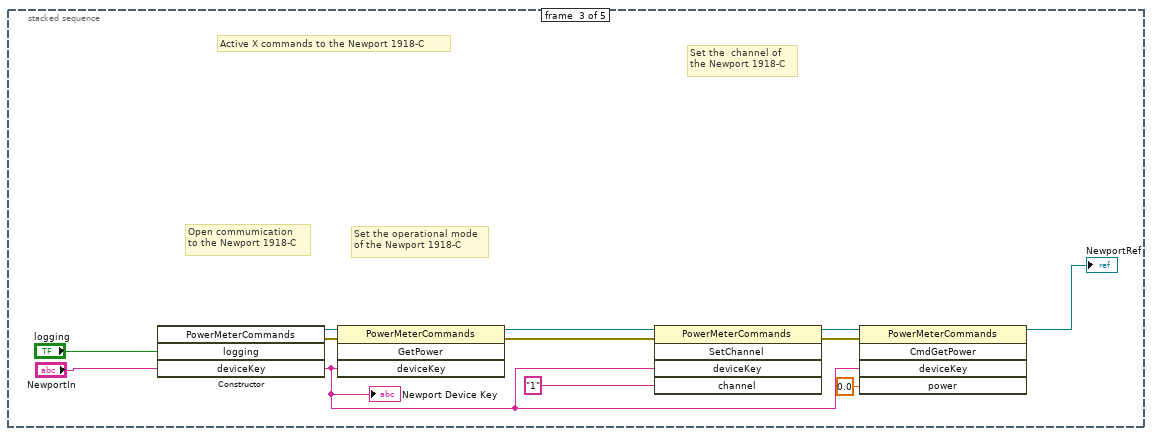
[diagram p13: hidden frame]
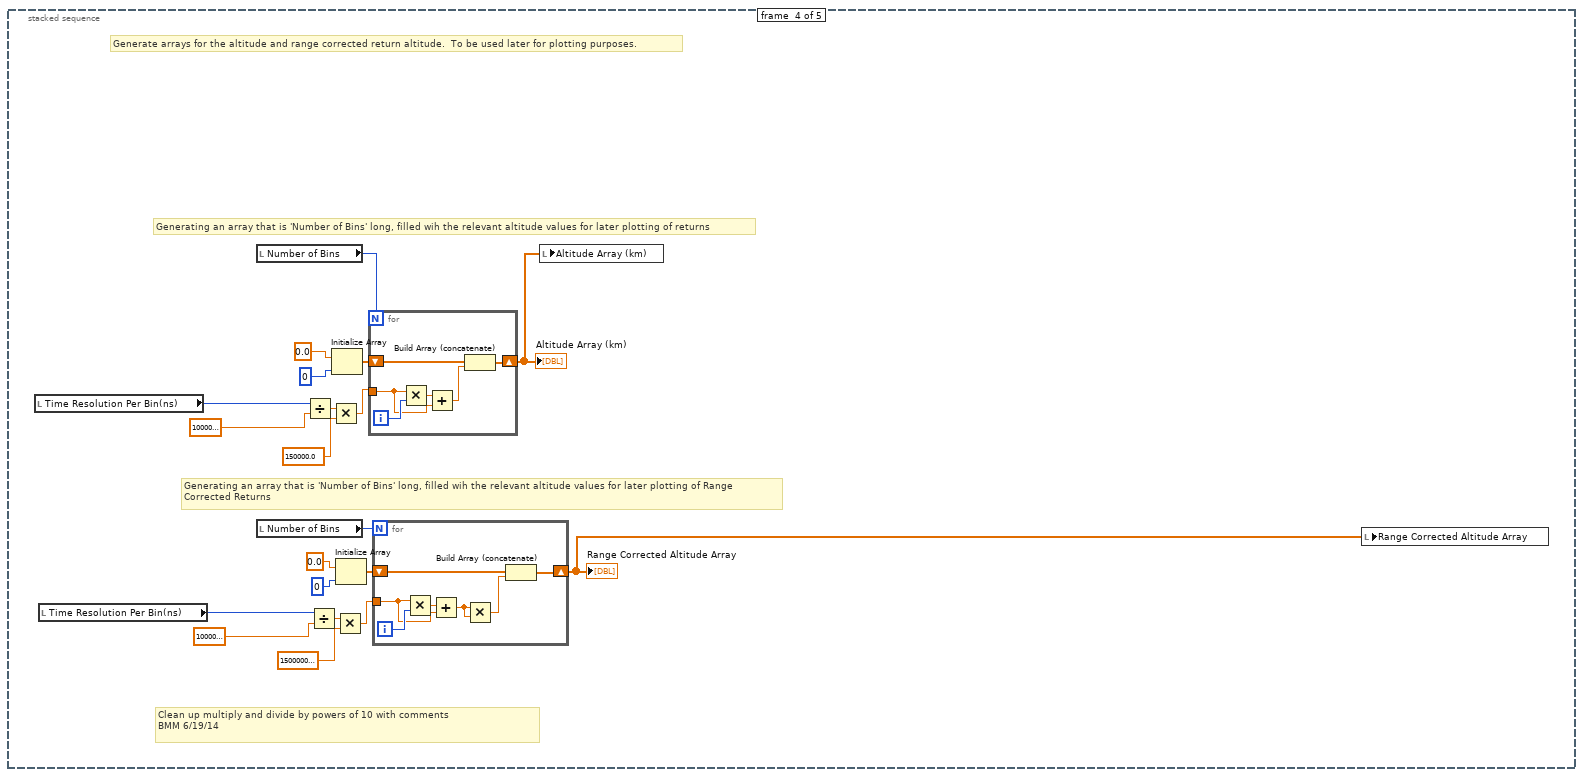
[diagram p14: hidden frame]
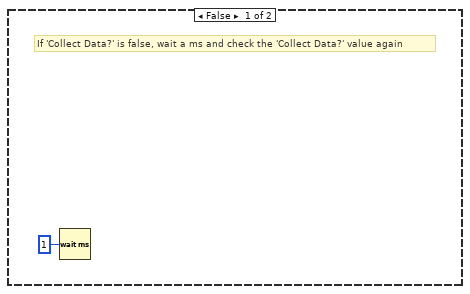
[diagram p15: hidden frame]
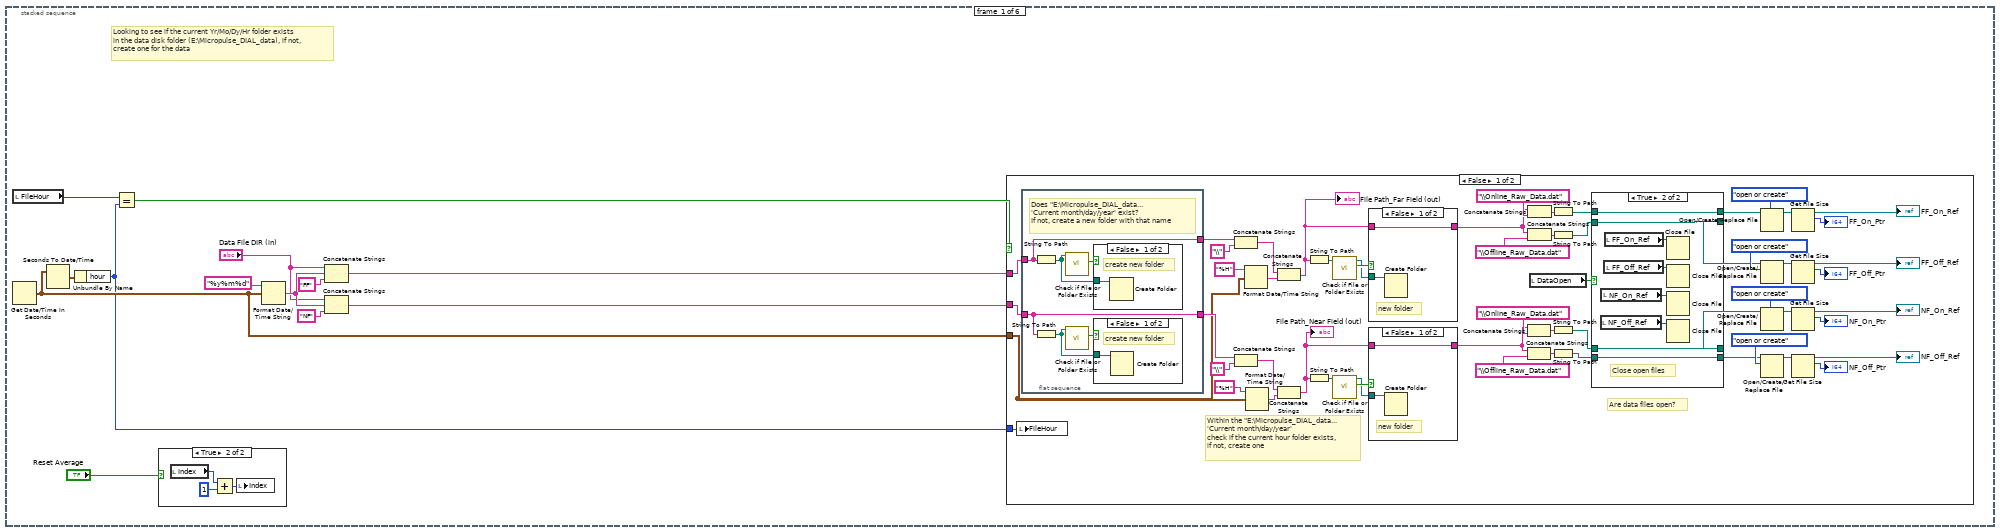
[diagram p16: hidden frame]
diagram:
  # "Frame 0: Initialize the scaler card (and start the MCSC)\nFrame 1: Initialize the DBR's\nFrame 2: Generate address string for talking the to Newport Power meter\nFrame 3: Generate altitude axes for regular and range corrected returns\nFrame 4: Collect data"
  n1 = stacked-sequence {
    tunnel: [_ _ _ _ w131] -> w3
    frame #0 {
      # "Open Bristol WM"
      n2 = disable-structure shown="Enabled" {
        disable-tunnel: [w16 _] -> w5
        frame Enabled {
          # "Initialization of the AMCS card, this where all of the scaler card parameters\nsuch as number of channels and accumulates is written to the card"
          n3 = stacked-sequence {
            tunnel: ["Time Resolution Per Bin(ns)"] -> w16
            frame #0 {
              # "Sets The Registers Of The Card"
              # "Number Of Channels Used"
              n4 = To Unsigned Long Integer(number="Sync Pulse Polarity") -> (unsigned 32bit integer=w18:u32)
              n5 = To Unsigned Long Integer(number="Pulse A Polarity") -> (unsigned 32bit integer=w22:u32)
              n6 = To Unsigned Long Integer(number="Pulse B Polarity") -> (unsigned 32bit integer=w20:u32)
              n7 = expression code="x*4"(w18) -> (w27:u32)
              n8 = expression code="x*2"(w22) -> (w26:u32)
              n9 = expression code="(x-1)*256"(u32 4 ("Number of Channels Used")) -> (w25:u32)
              n10 = expression code="x/10"("Time Resolution Per Bin(ns)") -> (w28:u32)
              n11 = expression code="x/80"("Pulse A Delay(ns)") -> (w35:u32)
              n12 = expression code="x/80"("Pulse B Delay(ns)") -> (w37:u32)
              n13 = expression code="x/10"("Accumulation Delay(ns)") -> (w36:u32)
              n14 = Compound Arithmetic op=ADD(w27, w26, w20, w25) -> (w24:u32)
              n15 = Build Array(w24, "Number of Bins", "Number of Accumulates", w28, w35, w37, w36) -> ()  [unwired: 1 out]
              n16 = local write "ns scale"("Time Resolution Per Bin(ns)") -> ()
              n17 = local write "y offset"("Accumulation Delay(ns)") -> ()
              n18 = local write "bins"("Number of Bins") -> ()
            }
          }
        }
        frame Disabled {
        }
      }
      n19 = local read "WS_On/Off"() -> (w7:bool)
      n20 = local read "Number of Bins"() -> (w11:u32)
      n21 = Multiply(x=0.15, y=w5) -> (x*y=w4:dbl)
      n22 = case shown="True" w7 {
        frame False {
        }
        frame True {
          n23 = call "T_RH_P.vi"("VISA in"="WS visa", "WS_Commands"=enum16{"OpenWS", "ReadTRHP", "CloseWS"}."OpenWS") -> ("TRHP"=→"TRHP":T13)  [unwired: 11 in, 2 out]
        }
      }
      n24 = property on="CH 3 (HSRL comb) counts display" class="IntChart (strict)"("YScale.Multiplier"=w4) -> ()  [unwired: 2 in, 2 out]
      n25 = property on="NRB 2" class="IntChart (strict)"("YScale.Multiplier"=w4) -> ()  [unwired: 2 in, 2 out]
      n26 = Decrement(x=w11) -> (x-1=w10:u32)
      n27 = Subtract(x=w10, y="background length") -> (x-y=→"background start":u32)
      "Index" <- 0 ("Index")
    }
    frame #1 {
      # "Test to see if the lasers are on"
      # "Initializing the DBR's.  In this frame the online and offline DBR's are set to the front panel specified initial currents and then the Agiltron switch is toggled to the online channel"
      n28 = disable-structure shown="Disabled" {
        frame Disabled {
          # "Frame 0: Set the online DBR current, Frame 1: Generate a command for the offline DBR initialization but don't actually implement, Frame 2: Switch the \nAgiltron switch to the online channel"
          n29 = stacked-sequence {
            frame #0 {
              # "In this frame, two command strings are written the the ILX laser diode controller.  First, the string \"LAS:CHAN 1\" is written\nthe the ILX's GPIB address specifying that you want to write any following commands to the online channel,\n, then the string \"LAS:LDI 'Lamda On DBR Current'\" is written setting the current of the online channel (1) to the specified \ndiode current"
              n30 = flat-sequence {
                tunnel: [w71] -> w69
                tunnel: w69 -> [w73]
                frame #0 {
                  # "The GPIB address of the ILX controller"
                  # "Specifying laser channel 1,\nwhich is the online channel"
                  n31 = local write "ILX Address"("ILX Address") -> ()
                  n32 = Number To Decimal String(number="ILX Address") -> (decimal integer string=w71:string)  [unwired: 1 in]
                  n33 = GPIB Write(0:w71, 1:"LAS:CHAN 2") -> ()  [unwired: 3 in, 2 out]
                }
                frame #1 {
                  # "Telling the controller to\nset the current"
                  # "string formatter"
                  # "Set current to specified current"
                  n34 = Format Into String(format string="%.4f" ("Format String"), "Lambda On DBR Current") -> (resulting string=w76:string)  [unwired: 2 in, 1 out]
                  n35 = local write "Lambda On DBR Current"("Lambda On DBR Current") -> ()
                  n36 = Concatenate Strings("LAS:LDI ", w76) -> (w77:string)
                  n37 = GPIB Write(0:w73, 1:w77) -> ()  [unwired: 3 in, 2 out]
                }
              }
            }
            frame #1 {
              # "This frame does not actually appear to do anything, I'm not sure why Amin originally put anything in this frame.  What does occur, \nis that the output current for the offline channel is specified and a command is generated, but, not written, to enable the output of the\noffline laser.  Although, the command is never written, as nearly as I can figure, the idea was that the offline never actually needs to be \naltered, so it will just be left in whatever state it started in upon the program startup."
              n38 = local read "ILX Address"() -> (w79:i32)
              n39 = Number To Decimal String(number=w79) -> ()  [unwired: 1 in, 1 out]
              n40 = Number To Engineering String(4:"Lambda Off DBR Current") -> (0:w83:string)  [unwired: 3 in]
              n41 = local write "Lambda Off DBR Current"("Lambda Off DBR Current") -> ()
              n42 = Concatenate Strings(":SOUR2:FUNC DC; :SOUR2:VOLT:OFFS ", w83, "V; :OUTP2:STAT ON") -> ()  [unwired: 1 out]
            }
            frame #2 {
              # "REPLACE WITH NEW AGILTRON TASK!"
              # "First one"
              # "Address of the Agiltron switch, only altered if the COM port changes,\nif the USB to serial converter changes or the usb port that is is plugged\nin to changes, this may vary.  Check the \"Devices and Printers\" and find \nout which com port the Agiltron switch is under should you see an error \nand adjust the adress on the front panel to match the switch address"
              # "Hex command written to \nthe switch for the online channel"
              # "Switch the Agiltron switch to the online channel, once switched, the online DBR is the laser seeding the TSOA"
              n43 = local read "Switch Comm Port"() -> (w84:refnum<visa-resource-name>)
              n44 = VISA Write(VISA resource name=w84, write buffer="\u0001\u0012\u0000\u0002") -> ()  [unwired: 1 in, 3 out]
            }
          }
        }
        frame Enabled {
        }
      }
      n45 = call "TL_Driver_v2.vi"("Device In"="Device In", "Commands"=T9."Open_TL", "Settings"="Settings") -> ("Device Out"=w49:refnum<visa-resource-name>)  [unwired: 9 in, 3 out]
      n46 = call "TL_Driver_v2.vi"("Device In"=w49, "Commands"=T9."Read_Status", "Settings"="Settings") -> ("Device Out"=w47:refnum<visa-resource-name>, "Readings"=w38:T7)  [unwired: 9 in, 2 out]
      "Readings" <- w38
      n47 = Unbundle By Name(w38) -> ("WV Offline LD"=w42:bool, "WV Etalon TEC"=w43:bool)
      n48 = Compound Arithmetic op=AND(TRUE, w42, w43) -> (w41:bool)
      n49 = case shown="False" w41 {
        tunnel: w47 -> [w52 w55]
        tunnel: [w52 w55] -> w45
        frame False {
          n50 = One Button Dialog(message="LASERS NOT ON!", button name ("OK")="CONTINUE") -> ()  [unwired: 1 out]
        }
        frame True {
        }
      }
      n51 = disable-structure shown="Enabled" {
        frame Disabled {
          # "Initialize the ILX to the front panel temperatures and currents for the on line and off line DBRs\nTurn on the TECs - does not turn on the lasers or set the Agiltron switches"
          n52 = call "ILX2.vi"("ILX Command"=T10."Initialize ILX") -> ("Device Out"=w63:refnum<visa-resource-name>)  [unwired: 10 in, 4 out]
          n53 = call "ILX2.vi"("Device In"=w63, "TEC Control"=TRUE, "ILX Command"=T10."TEC ON/OFF") -> ("Device Out"=w60:refnum<visa-resource-name>)  [unwired: 8 in, 4 out]
          n54 = flat-sequence {
            tunnel: w60 -> [w67]
            tunnel: [w67] -> w57
            frame #0 {
              # "Wait 30 seconds for\nthe ILX to stabilize"
              n55 = Wait (ms)(milliseconds to wait=u32 30000) -> ()  [unwired: 1 out]
            }
          }
          n56 = call "ILX2.vi"("Device In"=w57, "ILX Command"=T10."LASER ON/OFF", "Laser Control"=TRUE ("TEC Control")) -> ("Device Out"=w56:refnum<visa-resource-name>)  [unwired: 8 in, 4 out]
          n57 = flat-sequence {
            tunnel: w56 -> [w65]
            tunnel: [w65] -> _
            frame #0 {
              # "Wait 5 seconds for\nthe ILX to stabilize"
              n58 = Wait (ms)(milliseconds to wait=u32 5000) -> ()  [unwired: 1 out]
            }
          }
        }
        frame Enabled {
        }
      }
      n59 = call "TL_Driver_v2.vi"("Device In"=w45, "Commands"=T9."Read_Status", "Settings"="Settings") -> ("Readings"=w40:T7)  [unwired: 9 in, 3 out]
      n60 = local write "Readings"(w40) -> ()
      n61 = local write "Settings"("Settings") -> ()
    }
    frame #2 {
      # "Active X commands to the Newport 1918-C"
      # "Set the  channel of\nthe Newport 1918-C"
      # "Set the operational mode\nof the Newport 1918-C"
      # "Open commumication\nto the Newport 1918-C"
      n62 = constructor class="PowerMeterCommands"("logging"="logging", "deviceKey"="NewportIn") -> (reference out=w97:refnum<k24>, error out=w94:errorcluster, "deviceKey"=w89:string)  [unwired: 3 in, 2 out]
      "Newport Device Key" <- w89
      n63 = invoke class="PowerMeterCommands" method="GetPower"(reference=w97, error in=w94, "deviceKey"=w89) -> (reference out=w96:refnum<k24>, error out=w93:errorcluster)  [unwired: 1 in, 2 out]
      n64 = invoke class="PowerMeterCommands" method="SetChannel"(reference=w96, error in=w93, "deviceKey"=w89, "channel"="1") -> (reference out=w90:refnum<k24>, error out=w92:errorcluster)  [unwired: 1 in, 3 out]
      n65 = invoke class="PowerMeterCommands" method="CmdGetPower"(reference=w90, error in=w92, "deviceKey"=w89, "power"=sgl 0.0) -> (reference out=→"NewportRef":refnum<k24>)  [unwired: 1 in, 4 out]
    }
    frame #3 {
      # "Clean up multiply and divide by powers of 10 with comments\nBMM 6/19/14"
      # "Generating an array that is 'Number of Bins' long, filled wih the relevant altitude values for later plotting of Range \nCorrected Returns"
      # "Generating an array that is 'Number of Bins' long, filled wih the relevant altitude values for later plotting of returns"
      # "Generate arrays for the altitude and range corrected return altitude.  To be used later for plotting purposes."
      n66 = local read "Time Resolution Per Bin(ns)"() -> (w110:u32)
      n67 = local read "Time Resolution Per Bin(ns)"() -> (w100:u32)
      n68 = local read "Number of Bins"() -> (w113:u32)
      n69 = local read "Number of Bins"() -> (w103:u32)
      n70 = Divide(x=w110, y=1000000000.0) -> (x/y=w108:dbl)
      n71 = Divide(x=w100, y=1000000000.0) -> (x/y=w98:dbl)
      n72 = Multiply(x=w108, y=150000.0) -> (x*y=w111:dbl)
      n73 = Initialize Array(0.0, 0) -> (w116:dbl[])
      n74 = Multiply(x=w98, y=150000000.0) -> (x*y=w101:dbl)
      n75 = Initialize Array(0.0, 0) -> (w106:dbl[])
      n76 = for {
        N: w113 -> [_]
        shift-right: [w129] -> w114
        shift-left: w116 -> [w130]
        tunnel: w111 -> [w126]
        i -> [w128]
        n77 = Multiply(x=w126, y=w128) -> (x*y=w127:dbl)
        n78 = Add(x=w127, y=w126) -> (x+y=w125:dbl)
        n79 = Build Array (concatenate)(w130, w125) -> (w129:dbl[])
      }
      "Altitude Array (km)" <- w114
      n80 = for {
        N: w103 -> [_]
        shift-right: [w123] -> w104
        shift-left: w106 -> [w124]
        tunnel: w101 -> [w119]
        i -> [w122]
        n81 = Multiply(x=w119, y=w122) -> (x*y=w120:dbl)
        n82 = Add(x=w120, y=w119) -> (x+y=w118:dbl)
        n83 = Multiply(x=w118, y=w118) -> (x*y=w121:dbl)
        n84 = Build Array (concatenate)(w124, w121) -> (w123:dbl[])
      }
      "Range Corrected Altitude Array" <- w104
      n85 = local write "Altitude Array (km)"(w114) -> ()
      n86 = local write "Range Corrected Altitude Array"(w104) -> ()
    }
    frame #4 {
      # "Frame 4: Collect data from the scaler card and process and file it"
      n87 = while {
        tunnel: ["stop"] -> w131
        i -> [w132]
        stop <- "stop" stop-if-true
        # "While loop continues data collection cycle"
        n88 = case shown="True" "Collect Data?" {
          frame False {
            # "If 'Collect Data?' is false, wait a ms and check the 'Collect Data?' value again"
            n89 = Wait (ms)(milliseconds to wait=u32 1) -> ()  [unwired: 1 out]
          }
          frame True {
            # "Frame 3: Read the offline wavelength and lock if necessary (code not finished), read output power, read offline data, perform calculations and plot/save offline and NRB data, switch to online\nFrame 4: Calculate the absorption cross section (if wavelength, T, or P changed)\nFrame 5: Calculate Water Vapor Number density and plot"
            # "Frame 0: Create folders and file paths for logging the data, initialize averaging index\nFrame 1: Import current pressure and temperature data from COE weather station\nFrame 2: Read the online wavelength and lock if necessary, read online data and output power\n, plot and save online data, switch to offline DBR"
            # "If 'Collect Data?' is true, collect, process, and log data"
            n90 = stacked-sequence {
              frame #0 {
                # "Looking to see if the current Yr/Mo/Dy/Hr folder exists\nin the data disk folder (E:\\Micropulse_DIAL_data), if not,\ncreate one for the data"
                n91 = local read "FileHour"() -> (w145:i32)
                n92 = Get Date/Time In Seconds() -> (seconds since 1Jan1904=w137:timestamp)
                n93 = Seconds To Date/Time(time stamp (now)=w137) -> (date time rec=w147:T14)  [unwired: 1 in]
                n94 = Unbundle By Name(w147) -> ("hour"=w136:i32)
                n95 = Equal?(x=w145, y=w136) -> (x = y?=w146:bool)
                n96 = case shown="True" "Reset Average" {
                  frame False {
                    n97 = local write "Index"(0 ("Index")) -> ()
                  }
                  frame True {
                    n98 = local read "Index"() -> (w235:i32)
                    n99 = Add(x=w235, y=1) -> (x+y=w234:i32)
                    n100 = local write "Index"(w234) -> ()
                  }
                }
                n101 = Format Date/Time String(time format string (%c)="%y%m%d", seconds (now)=w137) -> (date/time string=w141:string)  [unwired: 1 in]
                n102 = Concatenate Strings("Data File DIR (in)", w141, "FF" ("string")) -> (w143:string)
                n103 = Concatenate Strings("Data File DIR (in)", w141, "NF" ("string")) -> (w138:string)
                n104 = case shown="False" w146 {
                  tunnel: w143 -> [w205 _]
                  tunnel: w138 -> [w204 _]
                  tunnel: w137 -> [w191 _]
                  tunnel: w136 -> [w167 _]
                  frame False {
                    # "Are data files open?"
                    # "Within the \"E:\\Micropulse_DIAL_data...\n'Current month/day/year' \ncheck if the current hour folder exists,\nif not, create one"
                    n105 = local write "FileHour"(w167) -> ()
                    n106 = flat-sequence {
                      tunnel: [w225] -> w192
                      tunnel: w205 -> [w224]
                      tunnel: w204 -> [w225]
                      tunnel: [w224] -> w193
                      frame #0 {
                        # "Does \"E:\\Micropulse_DIAL_data...\n'Current month/day/year' exist?\nIf not, create a new folder with that name"
                        n107 = String To Path(string=w224) -> (path=w229:path)
                        n108 = String To Path(string=w225) -> (path=w227:path)
                        n109 = call <vilib>:"Check if File or Folder Exists.vi"("path"=w229) -> ("file or folder exists?"=w228:bool)  [unwired: 8 in, 2 out]
                        n110 = call <vilib>:"Check if File or Folder Exists.vi"("path"=w227) -> ("file or folder exists?"=w226:bool)  [unwired: 8 in, 2 out]
                        n111 = case shown="False" w228 {
                          tunnel: w229 -> [w231 _]
                          frame False {
                            # "create new folder"
                            n112 = Create Folder(path (use dialog)=w231) -> ()  [unwired: 2 in, 3 out]
                          }
                          frame True {
                            # "Folder exists\ndo nothing"
                          }
                        }
                        n113 = case shown="False" w226 {
                          tunnel: w227 -> [w230 _]
                          frame False {
                            # "create new folder"
                            n114 = Create Folder(path (use dialog)=w230) -> ()  [unwired: 2 in, 3 out]
                          }
                          frame True {
                            # "Folder exists\ndo nothing"
                          }
                        }
                      }
                    }
                    n115 = Concatenate Strings(w193, "\\" ("string")) -> (w200:string)
                    n116 = Concatenate Strings(w192, "\\" ("string")) -> (w195:string)
                    n117 = Format Date/Time String(time format string (%c)="%H", seconds (now)=w191) -> (date/time string=w203:string)  [unwired: 1 in]
                    n118 = Format Date/Time String(time format string (%c)="%H", seconds (now)=w191) -> (date/time string=w198:string)  [unwired: 1 in]
                    n119 = Concatenate Strings(w200, w203) -> (w163:string)
                    "File Path_Far Field (out)" <- w163
                    n120 = Concatenate Strings(w195, w198) -> (w164:string)
                    "File Path_Near Field (out)" <- w164
                    n121 = String To Path(string=w163) -> (path=w201:path)
                    n122 = String To Path(string=w164) -> (path=w196:path)
                    n123 = call <vilib>:"Check if File or Folder Exists.vi"("path"=w201) -> ("file or folder exists?"=w190:bool, "dup path"=w188:path)  [unwired: 8 in, 1 out]
                    n124 = call <vilib>:"Check if File or Folder Exists.vi"("path"=w196) -> ("file or folder exists?"=w189:bool, "dup path"=w187:path)  [unwired: 8 in, 1 out]
                    n125 = case shown="False" w190 {
                      tunnel: w188 -> [w222 _]
                      tunnel: w163 -> [w221 w223]
                      tunnel: [w221 w223] -> w161
                      frame False {
                        # "new folder"
                        n126 = Create Folder(path (use dialog)=w222) -> ()  [unwired: 2 in, 3 out]
                      }
                      frame True {
                        # "Folder exists\ndo nothing"
                      }
                    }
                    n127 = case shown="False" w189 {
                      tunnel: w187 -> [w219 _]
                      tunnel: w164 -> [w218 w220]
                      tunnel: [w218 w220] -> w162
                      frame False {
                        # "new folder"
                        n128 = Create Folder(path (use dialog)=w219) -> ()  [unwired: 2 in, 3 out]
                      }
                      frame True {
                        # "Folder exists\ndo nothing"
                      }
                    }
                    n129 = Concatenate Strings(w162, "\\Online_Raw_Data.dat" ("string")) -> (w181:string)
                    n130 = Concatenate Strings(w162, "\\Offline_Raw_Data.dat" ("string")) -> (w180:string)
                    n131 = Concatenate Strings(w161, "\\Online_Raw_Data.dat" ("string")) -> (w186:string)
                    n132 = Concatenate Strings(w161, "\\Offline_Raw_Data.dat" ("string")) -> (w185:string)
                    n133 = local read "DataOpen"() -> (w178:bool)
                    n134 = String To Path(string=w186) -> (path=w177:path)
                    n135 = String To Path(string=w185) -> (path=w176:path)
                    n136 = String To Path(string=w181) -> (path=w175:path)
                    n137 = String To Path(string=w180) -> (path=w174:path)
                    n138 = case shown="True" w178 {
                      tunnel: w177 -> [w209 w213]
                      tunnel: [w209 w213] -> w171
                      tunnel: w176 -> [w208 w212]
                      tunnel: [w208 w212] -> w170
                      tunnel: w175 -> [w207 w211]
                      tunnel: [w207 w211] -> w169
                      tunnel: [w206 w210] -> w168
                      tunnel: w174 -> [w206 w210]
                      frame False {
                        # "No files open\ndo nothing"
                      }
                      frame True {
                        # "Close open files"
                        n139 = local read "NF_Off_Ref"() -> (w215:refnum<file>)
                        n140 = local read "NF_On_Ref"() -> (w214:refnum<file>)
                        n141 = local read "FF_Off_Ref"() -> (w217:refnum<file>)
                        n142 = local read "FF_On_Ref"() -> (w216:refnum<file>)
                        n143 = Close File(refnum=w216) -> ()  [unwired: 1 in, 2 out]
                        n144 = Close File(refnum=w217) -> ()  [unwired: 1 in, 2 out]
                        n145 = Close File(refnum=w214) -> ()  [unwired: 1 in, 2 out]
                        n146 = Close File(refnum=w215) -> ()  [unwired: 1 in, 2 out]
                      }
                    }
                    n147 = Open/Create/Replace File(file path (use dialog)=w171, operation (0:open)=T11."open or create") -> (refnum out=w157:refnum<file>)  [unwired: 4 in, 2 out]
                    n148 = Open/Create/Replace File(file path (use dialog)=w170, operation (0:open)=T11."open or create") -> (refnum out=w158:refnum<file>)  [unwired: 4 in, 2 out]
                    n149 = Open/Create/Replace File(file path (use dialog)=w169, operation (0:open)=T11."open or create") -> (refnum out=w159:refnum<file>)  [unwired: 4 in, 2 out]
                    n150 = Open/Create/Replace File(file path (use dialog)=w168, operation (0:open)=T11."open or create") -> (refnum out=w160:refnum<file>)  [unwired: 4 in, 2 out]
                    n151 = Get File Size(file=w157) -> (refnum out=→"FF_On_Ref":refnum<file>, size (in bytes)=→"FF_On_Ptr":i64)  [unwired: 1 in, 1 out]
                    n152 = Get File Size(file=w158) -> (refnum out=→"FF_Off_Ref":refnum<file>, size (in bytes)=→"FF_Off_Ptr":i64)  [unwired: 1 in, 1 out]
                    n153 = Get File Size(file=w159) -> (refnum out=→"NF_On_Ref":refnum<file>, size (in bytes)=→"NF_On_Ptr":i64)  [unwired: 1 in, 1 out]
                    n154 = Get File Size(file=w160) -> (refnum out=→"NF_Off_Ref":refnum<file>, size (in bytes)=→"NF_Off_Ptr":i64)  [unwired: 1 in, 1 out]
                  }
                  frame True {
                    # "Don't need to do anything!"
                  }
                }
              }
              frame #1 {
                # "Writing and plotting retrieved\nweather parameters"
                # "Matlab script goes online and retrieves most recent press, temp, and relative humidity data \nfrom the weather station on the roof of Cobleigh"
                # "Importing the current weather conditions from the COE weather station"
                n155 = disable-structure shown="Disabled" {
                  frame Disabled {
                    n156 = script code="%try\n%s=urlread('http://www.coe.montana.edu/ee/weather/mostCurrentCSV.php');\n%amin=textscan(s,'%s %s %s %s %s %s %s %s %s %s %s %s %s');\n%data=amin{1}{2};\n%[test remain]=strtok(data,',');\n%remain=str2num(remain);\n%press=remain(3)./1000;\n%temp=remain(5);\n%RH=remain(7);\n%catch\npress=.850;\ntemp=20;\nRH=40;\n%end"() -> ()  [unwired: 1 in, 4 out]
                  }
                  frame Enabled {
                  }
                }
                n157 = local read "WS_On/Off"() -> (w236:bool)
                n158 = case shown="True" w236 {
                  frame False {
                  }
                  frame True {
                    n159 = local read "WS visa"() -> (w241:refnum<visa-resource-name>)
                    n160 = call "T_RH_P.vi"("VISA in"=w241, "WS_Commands"=enum16{"OpenWS", "ReadTRHP", "CloseWS"}."ReadTRHP") -> ("TRHP"=w237:T13)  [unwired: 11 in, 2 out]
                    n161 = local write "TRHP"(w237) -> ()
                    n162 = Unbundle By Name(w237) -> ("Temp"=→"Temperature (C)":dbl, "RelH"=→"Relative Humdity (%)":dbl, "Press"=→"Pressure (mb)":dbl)
                  }
                }
              }
              frame #2 {
                # "Frame 3: Read, process, and plot online data\nFrame 4:\nFrame 5: Write the data to the folders from Frame 0 of outter sequence"
                # "Frame 0: Read the online wavelength and adjust to locking tolerance if out of range, Switch to offline DBR\nFrame 1: Read the output power from the Newport meter, calculate and plot the output pulse energy\nFrame 2: Wait 'Scalar Wait Time' for buffer to clear other wavelength data"
                # "Online"
                n163 = stacked-sequence {
                  frame #0 {
                    # "Read the online wavelength and continue adjusting the online DBR if outside the wavelength tolerance\nuntil it is within tolerance"
                    n164 = while {
                      i -> [w246]
                      stop <- w243 stop-if-true
                      # "Frame 2: Decrement DBR current if above tolerance\nFrame 3: Increment DBR current if below tolerance"
                      # "Frame 0: Read the current wavelength from the wavemeter\nFrame 1: Calculate the difference between desired and actual wavelength"
                      # "Continue reading and adjusting online DBR current until within locking tolerance"
                      n165 = stacked-sequence {
                        tunnel: w246 -> [w248 _ _ _ _]
                        tunnel: [_ _ w262 _ _] -> w244
                        frame #0 {
                          n166 = Equal To 0?(x=w248) -> (x = 0?=w247:bool)
                          n167 = case shown="True" w247 {
                            frame False {
                            }
                            frame True {
                              # "Set the TSOA switch to\namplify the ABSORBING\nwavelength"
                              n168 = Build Array(FALSE ("Boolean")) -> (w249:bool[])
                              n169 = call-poly <vilib>:"DAQmx Write.vi"("task/channels in"=refnum<k21> "BristolWM", "data"=w249) -> ()  [unwired: 11 in, 3 out]
                            }
                          }
                        }
                        frame #1 {
                          # "Reading the wavelength from the wavemeter"
                          n170 = flat-sequence {
                            tunnel: [w254] -> w253
                            tunnel: w253 -> [w257]
                            tunnel: [w256] -> w252
                            tunnel: w252 -> [w260]
                            frame #0 {
                              n171 = local read "Bristol In"() -> (w255:i32)
                              n172 = dll-call lib="C:/Users/H2ODial/Desktop/Shared Telescope WV DIAL Code/bristol/CLDevIface.dll" fn="CLOpenUSBSerialDevice"("commPort"=w255) -> ("return type"=w254:i32)  [unwired: 4 in, 2 out]
                            }
                            frame #1 {
                              n173 = dll-call lib="C:/Users/H2ODial/Desktop/Shared Telescope WV DIAL Code/bristol/CLDevIface.dll" fn="CLGetLambdaReading"("devHandle"=w257) -> ("return type"=→"WV Online Read (nm)":dbl, "devHandle"=w256:i32)  [unwired: 3 in, 2 out]
                            }
                            frame #2 {
                              n174 = dll-call lib="C:/Users/H2ODial/Desktop/Shared Telescope WV DIAL Code/bristol/CLDevIface.dll" fn="CLCloseDevice"("commPort"=w260) -> ("return type"=w259:i32)  [unwired: 4 in, 2 out]
                              n175 = local write "Bristol Out"(w259) -> ()
                            }
                          }
                        }
                        frame #2 {
                          # "If WL difference is within tolerance, stop looping, and illuminate 'Wavelength Lock Online' indicator"
                          # "Calculating the difference between the actual and desired online wavelength"
                          n176 = local read "WV Online Read (nm)"() -> (w261:dbl)
                          n177 = local read "Online_Tol"() -> (w267:dbl)
                          n178 = Multiply(x=-1.0, y=w267) -> (x*y=w268:dbl)
                          n179 = Subtract(x=w261, y="WV Online Set (nm)") -> (x-y=w263:dbl)
                          "WL_Difference" <- w263
                          n180 = Greater?(x=w263, y=w268) -> (0:w264:bool)
                          n181 = Less?(x=w263, y=w267) -> (x < y?=w265:bool)
                          n182 = And(x=w264, y=w265) -> (x .and. y?=w262:bool)
                          "Wavelength Lock Online" <- w262
                        }
                        frame #3 {
                          # "If the wavelength difference is greater that 0.0002 nm, decrement the \nDBR current by 0.01 mA"
                          n183 = local read "WL_Difference"() -> (w272:dbl)
                          n184 = Greater Or Equal?(x=w272, y="Online_Tol") -> (x >= y?=w271:bool)
                          n185 = case shown="True" w271 {
                            frame False {
                              # "Wavelength difference is not greater than 0.0002 nm, do nothing"
                            }
                            frame True {
                              # "Generating a command string\nto decrement the current"
                              # "WL difference is greater than 0.0002 nm,\ndecrement the DBR current by 0.01 mA"
                              n186 = local read "Settings"() -> (w279:T6)
                              n187 = local read "y"() -> (w274:dbl)
                              n188 = Unbundle By Name(w279) -> ("WV Online TEC"=w278:dbl)
                              n189 = local read "Device In"() -> (w275:refnum<visa-resource-name>)
                              n190 = Subtract(x=w278, y=w274) -> (x-y=w277:dbl)
                              n191 = Bundle By Name(cluster=w279, "WV Online TEC"=w277, "Module"=T12."WV Online TEC") -> (w281:T6)
                              n192 = call "TL_Driver_v2.vi"("Device In"=w275, "Commands"=T9."SET", "Settings"=w281) -> ("Readings"=w280:T7)  [unwired: 9 in, 3 out]
                              n193 = local write "Settings"(w281) -> ()
                              n194 = local write "Readings"(w280) -> ()
                            }
                          }
                        }
                        frame #4 {
                          # "If WL difference is < 0.0002 nm, increment the DBR current"
                          n195 = local read "Online_Tol"() -> (w283:dbl)
                          n196 = local read "WL_Difference"() -> (w286:dbl)
                          n197 = Multiply(x=-1.0, y=w283) -> (x*y=w282:dbl)
                          n198 = Less Or Equal?(x=w286, y=w282) -> (x <= y?=w285:bool)
                          n199 = case shown="True" w285 {
                            frame False {
                              # "WL difference is no <= to -0.0002 nm, do nothing"
                            }
                            frame True {
                              # "WL difference is < -0.0002,\nincrement the DBR current by 0.01 mA"
                              # "Generating a command string\nto decrement the current"
                              n200 = local read "Settings"() -> (w295:T6)
                              n201 = Unbundle By Name(w295) -> ("WV Online TEC"=w292:dbl)
                              n202 = local read "y"() -> (w288:dbl)
                              n203 = local read "Device In"() -> (w289:refnum<visa-resource-name>)
                              n204 = Add(x=w292, y=w288) -> (x+y=w291:dbl)
                              n205 = Bundle By Name(cluster=w295, "WV Online TEC"=w291, "Module"=T12."WV Online TEC") -> (w294:T6)
                              n206 = call "TL_Driver_v2.vi"("Device In"=w289, "Commands"=T9."SET", "Settings"=w294) -> ("Readings"=w293:T7)  [unwired: 9 in, 3 out]
                              n207 = local write "Settings"(w294) -> ()
                              n208 = local write "Readings"(w293) -> ()
                            }
                          }
                        }
                      }
                      n209 = Or(x=w244, y="Cancel online") -> (x .or. y?=w243:bool)
                    }
                  }
                  frame #1 {
                    # "Converting to pulse energy, assumes 5 percent pickoff"
                    # "Reading the Newport Power meter"
                    # "Reading the output power of the laser transmitter from the Newport power meter, once read, convert to corresponding pulse energy and plot"
                    n210 = local read "Newport Device Key"() -> (w300:string)
                    n211 = local read "NewportRef"() -> (w296:refnum<k24>)
                    n212 = disable-structure shown="Disabled" {
                      frame Disabled {
                        # "Plotting the online and offling pulse energies"
                        n213 = local read "Online Pulse Energy"() -> (w311:dbl)
                        n214 = local read "Offline Pulse Energy"() -> (w310:dbl)
                        n215 = Bundle("Online Pulse Energy"=w311, "Offline Pulse Energy"=w310) -> (→"Pulse Energy (Micro Joule)":T15)  [unwired: 1 in]
                      }
                      frame Enabled {
                      }
                    }
                    n216 = Number To Decimal String(number="SampleSize") -> (decimal integer string=w298:string)  [unwired: 1 in]
                    n217 = invoke class="PowerMeterCommands" method="PerformDAQ"(reference=w296, "deviceKey"=w300, "interval"="1", "sampleSize"=w298) -> ("PerformDAQ"=w301:dbl[])  [unwired: 2 in, 5 out]
                    n218 = call-poly <vilib>:"Mean.vi"("X"=w301) -> ("mean"=w299:dbl)  [unwired: 1 out]
                    n219 = Multiply(x=w299, y=1000.0) -> (x*y=w307:dbl)
                    n220 = Divide(x=w307, y=0.05) -> (x/y=w305:dbl)
                    n221 = Divide(x=w305, y=7.0) -> (x/y=→"Online Pulse Energy":dbl)
                  }
                  frame #2 {
                    # "Wait 'Scalar Wait Time' for the next available batch of scalar card data"
                    n222 = local read "AMCS_Profile"() -> (w312:i32)
                    n223 = disable-structure shown="Disabled" {
                      frame Disabled {
                        # "Waiting 'Scalar Wait Time'"
                        n224 = Wait (ms)(milliseconds to wait="Scalar Wait Time") -> ()  [unwired: 1 out]
                      }
                      frame Enabled {
                      }
                    }
                    n225 = while {
                      tunnel: [w319] -> w313
                      tunnel: [w315] -> _
                      tunnel: w312 -> [w315]
                      stop <- w317 stop-if-true
                      n226 = global read "AMCS_Data.vi" "AMCS_Profile"() -> (w319:i32)
                      n227 = Wait (ms)(milliseconds to wait=u32 10) -> ()  [unwired: 1 out]
                      n228 = Equal?(x=w319, y=w315) -> (x = y?=w318:bool)
                      n229 = case shown="False" w318 {
                        tunnel: [TRUE FALSE] -> w317
                        frame False {
                        }
                        frame True {
                        }
                      }
                    }
                    "AMCS_Profile" <- w313
                  }
                  frame #3 {
                    # "convert time per range bin to meters\nand calculate smoothed bins using\nsmoothing range"
                    # "Plotting online cross section and smoothed online data"
                    # "Calculate the bin by bin mean of the data"
                    # "Collect 'Integration Period (Seconds)' number\nof scalar data"
                    # "Reading, processing, and plotting the online data"
                    n230 = local read "Data Reads (number of loops)"() -> (w347:i32)
                    n231 = for {
                      N: w347 -> [_]
                      tunnel: [w368] -> w359 mode=indexing
                      tunnel: [w367] -> w322 mode=indexing
                      # "Scalar Data is retrieved from Global \nVariable that scaler.vi is writing to,"
                      n232 = global read "AMCS_Data.vi" "AMCS_Data"() -> (w371:u16[][])
                      n233 = disable-structure shown="Disabled" {
                        frame Disabled {
                          n234 = global read "Scalar_Data_3.vi" "Scalar Data 3"() -> ()  [unwired: 1 out]
                          n235 = global read "Scalar_Data.vi" "Scalar Data"() -> ()  [unwired: 1 out]
                        }
                        frame Enabled {
                        }
                      }
                      n236 = Index Array(array=w371, index (row) #1=0 ("index (row)"), index (row) #2=2 ("index (row)")) -> (element #1=w368:u16[], element #2=w367:u16[])  [unwired: 2 in]
                    }
                    n237 = Transpose 2D Array(2D array=w359) -> (transposed array=w363:u16[][])
                    n238 = Transpose 2D Array(2D array=w322) -> (transposed array=w345:u16[][])
                    n239 = for {
                      tunnel: w363 -> [w373] mode=indexing
                      tunnel: [w372] -> w364 mode=indexing
                      n240 = call-poly <vilib>:"Mean.vi"("X"=w373) -> ("mean"=w372:dbl)  [unwired: 1 out]
                    }
                    n241 = for {
                      tunnel: w345 -> [w366] mode=indexing
                      tunnel: [w365] -> w346 mode=indexing
                      n242 = call-poly <vilib>:"Mean.vi"("X"=w366) -> ("mean"=w365:dbl)  [unwired: 1 out]
                    }
                    n243 = local read "bins"() -> (w339:u32)
                    n244 = Array Subset(array=w364, index=1 ("dimension size"), length=w339) -> (w351:dbl[])
                    n245 = Array Subset(array=w346, index=1 ("dimension size"), length=w339) -> (w343:dbl[])
                    n246 = local read "background length"() -> (w329:i32)
                    n247 = local read "background start"() -> (w330:u32)
                    n248 = Array Size(array=w351) -> (size(s)=w348:i32)
                    n249 = Array Size(array=w343) -> (size(s)=w340:i32)
                    n250 = Initialize Array(1.0 ("element"), w348) -> (w350:dbl[])
                    n251 = Initialize Array(1.0 ("element"), w340) -> (w342:dbl[])
                    n252 = Multiply(x=w351, y=w350) -> (x*y=w352:dbl[])
                    "CH 0 Bin Readings" <- w352
                    n253 = Multiply(x=w343, y=w342) -> (x*y=w333:dbl[])
                    "CH 2 Bin Readings" <- w333
                    n254 = local read "Total DIAL Integration Time (Minutes)"() -> (w355:i32)
                    n255 = local read "Time Resolution Per Bin(ns)"() -> (w325:u32)
                    n256 = Array Subset(array=w352, index=w330, length=w329) -> (w361:dbl[])
                    n257 = Array Subset(array=w333, index=w330, length=w329) -> (w335:dbl[])
                    n258 = call-poly <vilib>:"Mean.vi"("X"=w361) -> ("mean"=w360:dbl)  [unwired: 1 out]
                    n259 = call-poly <vilib>:"Mean.vi"("X"=w335) -> ("mean"=w336:dbl)  [unwired: 1 out]
                    n260 = Divide(x=w355, y=w347) -> (x/y=w353:dbl)
                    n261 = local read "Index"() -> (w334:i32)
                    n262 = Subtract(x=w352, y=w360) -> (x-y=w357:dbl[])
                    n263 = Subtract(x=w333, y=w336) -> (x-y=w337:dbl[])
                    n264 = To Double Precision Float(number=w325) -> (double precision float=w326:dbl)
                    n265 = Multiply(x=w353, y=60.0) -> (x*y=w331:dbl)
                    n266 = Multiply(x=w326, y=0.15) -> (x*y=w328:dbl)
                    n267 = call "Ring Buffer Online Near.vi"("Index"=w334, "Profiles to Average"=w331, "Input Array"=w337) -> ("AvgArray"=w338:dbl[])  [unwired: 7 in, 1 out]
                    n268 = call "Ring Buffer Online Far.vi"("Index"=w334, "Profiles to Average"=w331, "Input Array"=w357) -> ("AvgArray"=w356:dbl[])  [unwired: 7 in, 1 out]
                    n269 = Divide(x="Smoothing Range", y=w328) -> (x/y=w323:dbl)
                    "Smoothed Bins" <- w323
                    n270 = call "Smooth Arrray.vi"("smooth size"=w323, "Raw Array"=w356) -> ("Smoothed Array"=→"CH0 (WV on) smoothed":dbl[])  [unwired: 9 in]
                    n271 = call "Smooth Arrray.vi"("smooth size"=w323, "Raw Array"=w338) -> ("Smoothed Array"=→"CH2 (molecular) smoothed":dbl[])  [unwired: 9 in]
                    n272 = disable-structure shown="Disabled" {
                      frame Disabled {
                        n273 = script code="format long;\ncounts=sum(Online);\nif counts >=0.5e6\ntime=time;\nelse\ntime=time\nend"() -> ()  [unwired: 3 in, 2 out]
                      }
                      frame Enabled {
                      }
                    }
                  }
                  frame #4 {
                    # "Toggling the Agiltron switch to the offline DBR seed laser"
                    n274 = disable-structure shown="Disabled" {
                      frame Disabled {
                        n275 = flat-sequence {
                          frame #0 {
                            # "Second one"
                            # "Command the switch to switch to position 2\ncorresponding to the offline DBR"
                            # "Hex string command \ncorrespond to offline"
                            n276 = VISA Write(VISA resource name="Switch Comm Port", write buffer="\u0001\u0012\u0000\u0001") -> ()  [unwired: 1 in, 3 out]
                          }
                        }
                      }
                      frame Enabled {
                      }
                    }
                  }
                  frame #5 {
                    # "Save the recently collected online data if 'Save Data?' is true"
                    n277 = case shown="True" "Save Data?" {
                      frame False {
                        # "'Save Data?' is false, do nothing"
                      }
                      frame True {
                        # "'Save Data?' is true, save onfline data to the Data Disk"
                        # "Write only one copy of data at this time"
                        # "Retrieve Julian Date"
                        n278 = local read "Time Resolution Per Bin(ns)"() -> (w383:u32)
                        n279 = local read "Number of Accumulates"() -> (w381:u32)
                        n280 = local read "Number of Bins"() -> (w382:u32)
                        n281 = local read "WV Online Read (nm)"() -> (w377:dbl)
                        n282 = local read "Lambda On DBR Current"() -> (w405:dbl)
                        n283 = local read "CH 2 Bin Readings"() -> (w403:dbl[])
                        n284 = local read "Online Pulse Energy"() -> (w404:dbl)
                        n285 = local read "CH 0 Bin Readings"() -> (w407:dbl[])
                        n286 = To Double Precision Float(number=w383) -> (double precision float=w378:dbl)
                        n287 = To Double Precision Float(number=w382) -> (double precision float=w379:dbl)
                        n288 = To Double Precision Float(number=w381) -> (double precision float=w380:dbl)
                        n289 = call "Julian_Date_2.vi"() -> ("Julian Date"=w406:dbl)  [unwired: 11 in]
                        n290 = Build Array (concatenate)(w406, w377, w405, w404, w378, w379, w380, w407) -> (w398:dbl[])
                        n291 = Build Array (concatenate)(w406, w377, w405, w404, w378, w379, w380, w403) -> (w388:dbl[])
                        n292 = local write "DataOpen"(TRUE ("DataOpen")) -> ()
                        n293 = local read "NF_On_Ref"() -> (w386:refnum<file>)
                        n294 = local read "FF_On_Ref"() -> (w402:refnum<file>)
                        n295 = local read "NF_On_Ptr"() -> (w387:i64)
                        n296 = local read "FF_On_Ptr"() -> (w401:i64)
                        n297 = Set File Position(offset (in bytes) (0)=w401, refnum=w402) -> (refnum out=w399:refnum<file>, error out=w396:errorcluster)  [unwired: 2 in]
                        n298 = Set File Position(offset (in bytes) (0)=w387, refnum=w386) -> (refnum out=w392:refnum<file>, error out=w390:errorcluster)  [unwired: 2 in]
                        n299 = Write to Binary File(file (use dialog)=w392, data=w388, error in=w390, 5:FALSE ("prepend array or string size? (T)")) -> (refnum out=w391:refnum<file>, error out=w389:errorcluster)  [unwired: 2 in, 1 out]
                        n300 = Write to Binary File(file (use dialog)=w399, data=w398, error in=w396, 5:FALSE ("prepend array or string size? (T)")) -> (refnum out=w397:refnum<file>, error out=w395:errorcluster)  [unwired: 2 in, 1 out]
                        n301 = Get File Position(4:w389, 7:w391) -> (2:w385:i64)  [unwired: 2 out]
                        n302 = Get File Position(4:w395, 7:w397) -> (2:w394:i64)  [unwired: 2 out]
                        n303 = local write "NF_On_Ptr"(w385) -> ()
                        n304 = local write "FF_On_Ptr"(w394) -> ()
                      }
                    }
                  }
                }
              }
              frame #3 {
                # "Frame 3: Read offline data, calculate aerosol data, and plot offline and normalized relative backscatter\nFrame 4:\nFrame 5: Save the offline data and related information"
                # "Frame 0: Read the offline wavelength and lock if necessary, Switch to online DBR\nFrame 1: Read the output power from the Newport power meter\nFrame 2: Wait 'Scalar Wait Time' for buffers to clear of online contiminated data"
                # "offline"
                n305 = stacked-sequence {
                  frame #0 {
                    # "Every 60 data collection cycles, read the offline DBR wavelength, and if outside of wavelength tolerance, adjust DBR current until within tolerance"
                    n306 = local read "L_Count"() -> (w409:i32)
                    n307 = Quotient & Remainder(x=w409, y=60.0) -> (x-y*floor(x/y)=w410:dbl)  [unwired: 1 out]
                    n308 = Equal To 0?(x=w410) -> (x = 0?=w408:bool)
                    n309 = case shown="True" w408 {
                      frame False {
                      }
                      frame True {
                        n310 = while {
                          i -> [w415]
                          stop <- w413 stop-if-true
                          # "If WL difference is within tolerance, stop looping, and illuminate 'Wavelength Lock Offline' indicator"
                          # "Frame 2: Decrement DBR current if above tolerance\nFrame 3: Increment DBR current if below tolerance"
                          # "Frame 0: Read the current wavelength from the wavemeter\nFrame 1: Calculate the difference between desired and actual wavelength"
                          # "Continue reading and adjusting offline DBR current until within locking tolerance"
                          n311 = stacked-sequence {
                            tunnel: w415 -> [w417 _ _ _ _]
                            tunnel: [_ _ w431 _ _] -> w412
                            frame #0 {
                              n312 = Equal To 0?(x=w417) -> (x = 0?=w416:bool)
                              n313 = case shown="True" w416 {
                                frame False {
                                }
                                frame True {
                                # "Set the TSOA switch to\namplify the non ABSORBING\nwavelength"
                                n314 = Build Array(TRUE ("Boolean")) -> (w419:bool[])
                                n315 = call-poly <vilib>:"DAQmx Write.vi"("task/channels in"=refnum<k21> "BristolWM", "data"=w419) -> ()  [unwired: 11 in, 3 out]
                                n316 = Wait (ms)(milliseconds to wait=u32 3200) -> ()  [unwired: 1 out]
                                }
                              }
                            }
                            frame #1 {
                              # "Reading the wavelength from the wavemeter"
                              n317 = flat-sequence {
                                tunnel: [w424] -> w423
                                tunnel: w423 -> [w427]
                                tunnel: [w426] -> w422
                                tunnel: w422 -> [w430]
                                frame #0 {
                                n318 = local read "Bristol In"() -> (w425:i32)
                                n319 = dll-call lib="C:/Users/H2ODial/Desktop/Shared Telescope WV DIAL Code/bristol/CLDevIface.dll" fn="CLOpenUSBSerialDevice"("commPort"=w425) -> ("return type"=w424:i32)  [unwired: 4 in, 2 out]
                                }
                                frame #1 {
                                n320 = dll-call lib="C:/Users/H2ODial/Desktop/Shared Telescope WV DIAL Code/bristol/CLDevIface.dll" fn="CLGetLambdaReading"("devHandle"=w427) -> ("return type"=→"WV Offline Read (nm)":dbl, "devHandle"=w426:i32)  [unwired: 3 in, 2 out]
                                }
                                frame #2 {
                                n321 = dll-call lib="C:/Users/H2ODial/Desktop/Shared Telescope WV DIAL Code/bristol/CLDevIface.dll" fn="CLCloseDevice"("commPort"=w430) -> ("return type"=w429:i32)  [unwired: 4 in, 2 out]
                                n322 = local write "Bristol Out"(w429) -> ()
                                }
                              }
                            }
                            frame #2 {
                              # "Calculating the difference between the actual and desired online wavelength"
                              n323 = local read "Offline_Tol"() -> (w433:dbl)
                              n324 = local read "WV Offline Read (nm)"() -> (w439:dbl)
                              n325 = Multiply(x=-1.0, y=w433) -> (x*y=w432:dbl)
                              n326 = Subtract(x=w439, y="WV Offline Set (nm)") -> (x-y=w435:dbl)
                              "WL Difference off" <- w435
                              n327 = Greater?(x=w435, y=w432) -> (0:w436:bool)
                              n328 = Less?(x=w435, y=w433) -> (x < y?=w437:bool)
                              n329 = And(x=w436, y=w437) -> (x .and. y?=w431:bool)
                              "Wavelength Lock Offline" <- w431
                              n330 = case shown="True" w431 {
                                frame False {
                                }
                                frame True {
                                # "Set the TSOA switch to\namplify the ABSORBING\nwavelength"
                                n331 = Build Array(FALSE ("Boolean")) -> (w441:bool[])
                                n332 = call-poly <vilib>:"DAQmx Write.vi"("task/channels in"=refnum<k21> "BristolWM", "data"=w441) -> ()  [unwired: 11 in, 3 out]
                                n333 = Wait (ms)(milliseconds to wait=u32 3200) -> ()  [unwired: 1 out]
                                }
                              }
                            }
                            frame #3 {
                              # "If the wavelength difference is greater that 0.0002 nm, decrement the \nDBR current by 0.01 mA"
                              n334 = local read "WL Difference off"() -> (w446:dbl)
                              n335 = Greater Or Equal?(x=w446, y="Offline_Tol") -> (x >= y?=w445:bool)
                              n336 = case shown="True" w445 {
                                frame False {
                                # "Wavelength difference is not greater than 0.0002 nm, do nothing"
                                }
                                frame True {
                                # "Generating a command string\nto decrement the current"
                                n337 = local read "Settings"() -> (w453:T6)
                                n338 = Unbundle By Name(w453) -> ("WV Offline TEC"=w451:dbl)
                                n339 = Subtract(x=w451, y="y") -> (x-y=w450:dbl)
                                n340 = local read "Device In"() -> (w448:refnum<visa-resource-name>)
                                n341 = Bundle By Name(cluster=w453, "WV Offline TEC"=w450, "Module"=T12."WV Offline TEC") -> (w454:T6)
                                n342 = call "TL_Driver_v2.vi"("Device In"=w448, "Commands"=T9."SET", "Settings"=w454) -> ("Readings"=w455:T7)  [unwired: 9 in, 3 out]
                                n343 = local write "Settings"(w454) -> ()
                                n344 = local write "Readings"(w455) -> ()
                                }
                              }
                            }
                            frame #4 {
                              # "If WL difference is < 0.0002 nm, increment the DBR current"
                              n345 = local read "WL Difference off"() -> (w458:dbl)
                              n346 = Less Or Equal?(x=w458, y=-0.0001) -> (x <= y?=w456:bool)
                              n347 = case shown="True" w456 {
                                frame False {
                                # "WL difference is no <= to -0.0002 nm, do nothing"
                                }
                                frame True {
                                # "Generating a command string\nto decrement the current"
                                # "WL difference is less than 0.0002 nm,\nincrement the DBR current by 0.01 mA"
                                n348 = local read "Settings"() -> (w466:T6)
                                n349 = Unbundle By Name(w466) -> ("WV Offline TEC"=w464:dbl)
                                n350 = local read "y"() -> (w460:dbl)
                                n351 = Add(x=w464, y=w460) -> (x+y=w463:dbl)
                                n352 = local read "Device In"() -> (w461:refnum<visa-resource-name>)
                                n353 = Bundle By Name(cluster=w466, "WV Offline TEC"=w463, "Module"=T12."WV Offline TEC") -> (w467:T6)
                                n354 = call "TL_Driver_v2.vi"("Device In"=w461, "Commands"=T9."SET", "Settings"=w467) -> ("Readings"=w465:T7)  [unwired: 9 in, 3 out]
                                n355 = local write "Settings"(w467) -> ()
                                n356 = local write "Readings"(w465) -> ()
                                }
                              }
                            }
                          }
                          n357 = Or(x=w412, y="Cancel Offline") -> (x .or. y?=w413:bool)
                        }
                      }
                    }
                  }
                  frame #1 {
                    # "Reading the power meter"
                    # "Updating the pulse energy plot"
                    # "Converting to pulse energy"
                    # "Reading the offline output power, converting to pulse energy,  and updating the Pulse energy plot"
                    n358 = local read "SampleSize"() -> (w470:i32)
                    n359 = local read "Newport Device Key"() -> (w471:string)
                    n360 = local read "Online Pulse Energy"() -> (w477:dbl)
                    n361 = local read "Offline Pulse Energy"() -> (w476:dbl)
                    n362 = local read "NewportRef"() -> (w468:refnum<k24>)
                    n363 = Number To Decimal String(number=w470) -> (decimal integer string=w472:string)  [unwired: 1 in]
                    n364 = invoke class="PowerMeterCommands" method="PerformDAQ"(reference=w468, "deviceKey"=w471, "interval"="1", "sampleSize"=w472) -> ("PerformDAQ"=w473:dbl[])  [unwired: 2 in, 5 out]
                    n365 = Bundle("Online Pulse Energy"=w477, "Offline Pulse Energy"=w476) -> (w475:T15)  [unwired: 1 in]
                    n366 = local write "Pulse Energy (Micro Joule)"(w475) -> ()
                    n367 = call-poly <vilib>:"Mean.vi"("X"=w473) -> ("mean"=w469:dbl)  [unwired: 1 out]
                    n368 = Multiply(x=w469, y=1000.0) -> (x*y=w482:dbl)
                    n369 = Divide(x=w482, y=0.05) -> (x/y=w480:dbl)
                    n370 = Divide(x=w480, y=7.0) -> (x/y=→"Offline Pulse Energy":dbl)
                  }
                  frame #2 {
                    # "Added in the ability to interactively control the ThorLab  setting (just etalon temp for now)"
                    # "Wait 'Scalar Wait Time' for buffers to clear of online contiminated offline data"
                    n371 = disable-structure shown="Disabled" {
                      frame Disabled {
                        # "Wait 'Scalar Wait Time'"
                        n372 = local read "Scalar Wait Time"() -> (w492:u32)
                        n373 = Wait (ms)(milliseconds to wait=w492) -> ()  [unwired: 1 out]
                      }
                      frame Enabled {
                      }
                    }
                    n374 = event shown="[1] \"Settings.WV Etalon TEC\": Value Change" {
                      selector: _ -> [_ _]
                      dyn-events: _ -> [_ _]
                      timeout: 1 -> [_ _]
                      event Timeout {
                        n375 = event-data() -> ()  [unwired: 1 in, 2 out]
                      }
                      event "Settings.WV Etalon TEC": Value Change {
                        # "Generating a command string\nto update the etalon"
                        n376 = event-data() -> ()  [unwired: 1 in, 5 out]
                        n377 = local read "Settings"() -> (w489:T6)
                        n378 = Unbundle By Name(w489) -> ("WV Etalon TEC"=w491:dbl)
                        n379 = Bundle By Name(cluster=w489, "WV Etalon TEC"=w491, "Module"=T12."WV Etalon TEC") -> (w487:T6)
                        n380 = call "TL_Driver_v2.vi"("Device In"=refnum<visa-resource-name> "Pro8000", "Commands"=T9."SET", "Settings"=w487) -> ("Readings"=w488:T7)  [unwired: 9 in, 3 out]
                        n381 = local write "Readings"(w488) -> ()
                        n382 = local write "Settings"(w487) -> ()
                      }
                    }
                  }
                  frame #3 {
                    w527 = 1 ("dimension size")
                    w531 = 1
                    # "Read in latest scalar card data from \n'Scalar Data' global variable that \nscaler.vi is writing to, then wait 1 sec\nfor next batch of data"
                    # "Plotting the normalized relative \nbackscatter"
                    # "Calculating the normalized relative backscatter"
                    # "Calculating/Plotting smoothed data,\ncross sections etc."
                    # "Pick off data with\nout header"
                    # "Calculate mean bin by bin mean"
                    # "Reading in 'Integration Period (Seconds)' of data"
                    # "Read the offline data from the scalar card, perform smoothing, calculate normalized relative backscatter, and plot"
                    # "File path in MATLAB script is of old dial is:\nF:\\Micropulse DIAL\\Micropulse DIAL Matlab\\\nFinal Overlap Function.mat')];"
                    # "Collects Data From Card,\nSends It To The Chart,\nAnd Saves A Copy As A\nFile If Option Selected On\nFront Panel"
                    n383 = for {
                      N: "Data Reads (number of loops)" -> [_]
                      tunnel: [w563] -> w495 mode=indexing
                      tunnel: [w562] -> w494 mode=indexing
                      n384 = global read "AMCS_Data.vi" "AMCS_Data"() -> (w564:u16[][])
                      n385 = disable-structure shown="Disabled" {
                        frame Disabled {
                          n386 = global read "Scalar_Data_4.vi" "Scalar Data 4"() -> ()  [unwired: 1 out]
                          n387 = global read "Scalar_Data_2.vi" "Scalar Data 2"() -> ()  [unwired: 1 out]
                        }
                        frame Enabled {
                        }
                      }
                      n388 = Index Array(array=w564, index (row) #1=1 ("index (row)"), index (row) #2=3 ("index (row)")) -> (element #1=w563:u16[], element #2=w562:u16[])  [unwired: 2 in]
                    }
                    n389 = local read "Total DIAL Integration Time (Minutes)"() -> (w552:i32)
                    n390 = Divide(x=w552, y="Data Reads (number of loops)") -> (x/y=w550:dbl)
                    n391 = local read "Total Aerosol Integration Time (Minutes)"() -> (w554:dbl)
                    n392 = local read "background length"() -> (w499:i32)
                    n393 = Multiply(x=w550, y=60.0) -> (x*y=w537:dbl)
                    n394 = local read "background start"() -> (w500:u32)
                    n395 = Transpose 2D Array(2D array=w495) -> (transposed array=w560:u16[][])
                    n396 = Transpose 2D Array(2D array=w494) -> (transposed array=w543:u16[][])
                    n397 = Divide(x=w554, y="Data Reads (number of loops)") -> (x/y=w555:dbl)
                    n398 = for {
                      tunnel: w560 -> [w570] mode=indexing
                      tunnel: [w569] -> w561 mode=indexing
                      tunnel: w543 -> [w568] mode=indexing
                      tunnel: [w567] -> _ mode=indexing
                      tunnel: [w567] -> w540 mode=indexing
                      n399 = call-poly <vilib>:"Mean.vi"("X"=w570) -> ("mean"=w569:dbl)  [unwired: 1 out]
                      n400 = call-poly <vilib>:"Mean.vi"("X"=w568) -> ("mean"=w567:dbl)  [unwired: 1 out]
                    }
                    n401 = local read "bins"() -> (w528:u32)
                    n402 = Multiply(x=w555, y=60.0) -> (x*y=w518:dbl)
                    n403 = Array Subset(array=w540, index=w527, length=w528) -> (w541:dbl[])
                    "CH3 Bin Readings" <- w541
                    n404 = Array Subset(array=w561, index=w527, length=w528) -> (w539:dbl[])
                    "CH1  Bin Readings" <- w539
                    n405 = Array Subset(array=w541, index=w500, length=w499) -> (w542:dbl[])
                    n406 = Array Subset(array=w539, index=w500, length=w499) -> (w559:dbl[])
                    n407 = local read "Smoothed Bins"() -> (w496:dbl)
                    n408 = call-poly <vilib>:"Mean.vi"("X"=w542) -> ("mean"=w506:dbl)  [unwired: 1 out]
                    n409 = call-poly <vilib>:"Mean.vi"("X"=w559) -> ("mean"=w507:dbl)  [unwired: 1 out]
                    n410 = local read "Index"() -> (w517:i32)
                    n411 = Subtract(x=w541, y=w506) -> (x-y=w519:dbl[])
                    n412 = Subtract(x=w539, y=w507) -> (x-y=w535:dbl[])
                    n413 = call "Ring Buffer Offline Far.vi"("Index"=w517, "Profiles to Average"=w537, "Input Array"=w535) -> ("AvgArray"=w557:dbl[], "RingBufferOut"=→"CH1 RingBuffer long":dbl[][])  [unwired: 7 in]
                    n414 = call "Ring Buffer Aerosol Far.vi"("Index"=w517, "Profiles to Average"=w518, "Input Array"=w535) -> ("AvgArray"=w553:dbl[], "RingBufferOut"=→"CH1 RingBuffer short":dbl[][])  [unwired: 7 in]
                    n415 = call "Ring Buffer Offline Near.vi"("Index"=w517, "Profiles to Average"=w537, "Input Array"=w519) -> ("AvgArray"=w538:dbl[], "RingBufferOut"=→"CH3 RingBuffer long":dbl[][])  [unwired: 7 in]
                    n416 = call "Ring Buffer Aerosol Near.vi"("Index"=w517, "Profiles to Average"=w518, "Input Array"=w519) -> ("AvgArray"=w515:dbl[], "RingBufferOut"=→"CH3 RingBuffer short":dbl[][])  [unwired: 7 in]
                    n417 = Reshape Array(w535, w527, w528) -> (→"CH 1 (WV off) counts display":dbl[][])
                    n418 = Reshape Array(w519, w527, w528) -> (→"CH 3 (HSRL comb) counts display":dbl[][])
                    n419 = call "Smooth Arrray.vi"("smooth size"=w496, "Raw Array"=w557) -> ("Smoothed Array"=→"CH1 (WV off) smooth S":dbl[])  [unwired: 9 in]
                    n420 = call "Smooth Arrray.vi"("smooth size"=w496, "Raw Array"=w553) -> ("Smoothed Array"=w526:dbl[])  [unwired: 9 in]
                    "CH1 (WV off) smooth L" <- w526
                    n421 = call "Smooth Arrray.vi"("smooth size"=w496, "Raw Array"=w538) -> ("Smoothed Array"=→"CH3 (HSRL combined) smooth L":dbl[])  [unwired: 9 in]
                    n422 = call "Smooth Arrray.vi"("smooth size"=w496, "Raw Array"=w515) -> ("Smoothed Array"=w498:dbl[])  [unwired: 9 in]
                    "CH3 (HSRL combined) smooth S" <- w498
                    n423 = local read "Time Resolution Per Bin(ns)"() -> (w493:u32)
                    n424 = local read "Number of Accumulates"() -> (w502:u32)
                    n425 = local read "Temperature (C)"() -> (w549:dbl)
                    n426 = local read "Pressure (mb)"() -> (w548:dbl)
                    n427 = script code="%accum_num=10000;     % scaler card setting number of accumulations\nt_bin = t_bin/1e9                 % scaler card setting time per bin\n%t_d = 37.3e-9;                % APD dead time from spec sheet\n\n% conversion from accumulated counts to count rate  (c/s)\nc_convert = 1./t_bin./accum_num;\nCR_far = p_raw_far.*c_convert;\nCR_near = p_raw_near.*c_convert;\nCR_total_far = (p_raw_far+b_far).*c_convert;\nCR_total_near = (p_raw_near+b_near).*c_convert;\nb_CR_far =b_far.*c_convert;\nb_CR_near =b_near.*c_convert;\n \n% create a range array\nsize_p =  size(p_raw_far,2);\ngate = t_bin*3e8/2;\nr = (gate:gate:size_p*gate)./1e3; \n   \n%APD correction factor\n D_far = 1./(1-(t_d*CR_total_far));\n D_near = 1./(1-(t_d*CR_total_near));\n\n %Calculating normalize relative backscatter profile\n nrb_far = CR_far.*D_far.*r.^2.*1e-6;\n nrb_near = CR_near.*D_near.*r.^2.*1e-6;"("E"=6.0 ("Real"), "temp"=w549, "press"=w548, "p_raw_far"=w526, "b_far"=w507, "b_near"=w506, "p_raw_near"=w498, "accum_num"=w502, "t_d"="dead time", "t_bin"=w493) -> ("nrb_far"=w521:cdb[], "D_far"=w512:dbl[], "nrb_near"=w520:cdb[], "D_near"=w511:dbl[], "b_CR_far"=w504:dbl, "b_CR_near"=w503:dbl)  [unwired: 1 in, 1 out]
                    n428 = local read "bins"() -> (w530:u32)
                    n429 = local read "Altitude Array (km)"() -> (w523:dbl[])
                    n430 = Bundle(w504, w503) -> (→"?":cluster{dbl, dbl})  [unwired: 1 in]
                    n431 = Build Array(w521, w520) -> (w525:cdb[][])
                    n432 = Build Array(w512, w511) -> (w510:dbl[][])
                    n433 = Reshape Array(w520, w531, w530) -> (→"NRB 2":cdb[][])
                    n434 = Reshape Array(w521, w531, w530) -> (→"NRB":cdb[][])
                    n435 = Build Array(w523, w523) -> (w522:dbl[][])
                    n436 = call "Convert to Dynamic Data7"("2D Array"=w510) -> ("Dynamic Data Type"=w509:dynamicdata)  [unwired: 3 in]
                    n437 = call "Convert to Dynamic Data3"("2D Array"=w525) -> ("Dynamic Data Type"=w524:dynamicdata)  [unwired: 3 in]
                    n438 = call "Convert to Dynamic Data4"("2D Array"=w522) -> ("Dynamic Data Type"=w513:dynamicdata)  [unwired: 3 in]
                    n439 = call "Build XY Graph2"("Y Input"=w513, "X Input"=w524) -> ("XY Graph"=→"NRB plot":cluster{"Y":dbl[], "Y":dbl[]}[])  [unwired: 3 in, 6 out]
                    n440 = call "Build XY Graph4"("Y Input"=w513, "X Input"=w509) -> ("XY Graph"=→"Correction":cluster{"Y":dbl[], "Y":dbl[]}[])  [unwired: 3 in, 6 out]
                  }
                  frame #4 {
                    # "REPLACE WITH NEW AGILTRON TASK!"
                    # "Toggle Agiltron switch to online DBR"
                    n441 = disable-structure shown="Disabled" {
                      frame Disabled {
                        # "ABSORBING"
                        n442 = flat-sequence {
                          frame #0 {
                            # "Third one"
                            # "Command the switch to switch to position 1\ncorresponding to the online DBR"
                            # "Hex string command \ncorrespond to online"
                            n443 = local read "Switch Comm Port"() -> (w574:refnum<visa-resource-name>)
                            n444 = VISA Write(VISA resource name=w574, write buffer="\u0001\u0012\u0000\u0002") -> ()  [unwired: 1 in, 3 out]
                          }
                        }
                        n445 = Build Array(FALSE ("Boolean")) -> (w573:bool[])
                        n446 = call-poly <vilib>:"DAQmx Write.vi"("task/channels in"=refnum<k21> "AgiltronSwitch", "data"=w573) -> ()  [unwired: 11 in, 3 out]
                      }
                      frame Enabled {
                      }
                    }
                  }
                  frame #5 {
                    # "If 'Save Data?' is true, save all relavant offline info"
                    n447 = local read "Save Data?"() -> (w576:bool)
                    n448 = case shown="True" w576 {
                      frame False {
                        # "'Save Data?' is false, do nothing"
                      }
                      frame True {
                        # "Write only one data file at this time"
                        # "Retrive Julian Date"
                        # "'Save Data?' is true, save offline data to the Data Disk"
                        n449 = local read "Lambda Off DBR Current"() -> (w598:dbl)
                        n450 = local read "WV Offline Read (nm)"() -> (w597:dbl)
                        n451 = local read "Relative Humdity (%)"() -> (w602:dbl)
                        n452 = local read "CH3 Bin Readings"() -> (w595:dbl[])
                        n453 = local read "CH1  Bin Readings"() -> (w603:dbl[])
                        n454 = local read "Offline Pulse Energy"() -> (w599:dbl)
                        n455 = local read "Temperature (C)"() -> (w600:dbl)
                        n456 = local read "Pressure (mb)"() -> (w601:dbl)
                        n457 = call "Julian_Date_2.vi"() -> ("Julian Date"=w596:dbl)  [unwired: 11 in]
                        n458 = Build Array (concatenate)(w596, w597, w598, w599, w600, w601, w602, w603) -> (w581:dbl[])
                        n459 = Build Array (concatenate)(w596, w597, w598, w599, w600, w601, w602, w595) -> (w578:dbl[])
                        n460 = local read "FF_Off_Ref"() -> (w583:refnum<file>)
                        n461 = local read "NF_Off_Ref"() -> (w580:refnum<file>)
                        n462 = local read "FF_Off_Ptr"() -> (w582:i64)
                        n463 = local read "NF_Off_Ptr"() -> (w579:i64)
                        n464 = Set File Position(offset (in bytes) (0)=w582, refnum=w583) -> (refnum out=w594:refnum<file>, error out=w592:errorcluster)  [unwired: 2 in]
                        n465 = Set File Position(offset (in bytes) (0)=w579, refnum=w580) -> (refnum out=w590:refnum<file>, error out=w588:errorcluster)  [unwired: 2 in]
                        n466 = Write to Binary File(file (use dialog)=w594, data=w581, error in=w592, 5:FALSE ("prepend array or string size? (T)")) -> (refnum out=w593:refnum<file>, error out=w591:errorcluster)  [unwired: 2 in, 1 out]
                        n467 = Write to Binary File(file (use dialog)=w590, data=w578, error in=w588, 5:FALSE ("prepend array or string size? (T)")) -> (refnum out=w589:refnum<file>, error out=w587:errorcluster)  [unwired: 2 in, 1 out]
                        n468 = Get File Position(4:w591, 7:w593) -> (2:w584:i64)  [unwired: 2 out]
                        n469 = Get File Position(4:w587, 7:w589) -> (2:w577:i64)  [unwired: 2 out]
                        n470 = local write "FF_Off_Ptr"(w584) -> ()
                        n471 = local write "NF_Off_Ptr"(w577) -> ()
                      }
                    }
                  }
                }
              }
              frame #4 {
                n472 = First Call?() -> (First Call?: T/F=w606:bool)
                n473 = Or(x="calculate absorption cross sections", y=w606) -> (x .or. y?=w604:bool)
                n474 = case shown="True" w604 {
                  frame False {
                  }
                  frame True {
                    # "calculate absorption cross sections from HITRAN data base"
                  }
                }
              }
              frame #5 {
                # "Data Processing Far Channel"
                # "Calculating the range resolved water vapor number density and plotting"
              }
            }
          }
        }
        "L_Count" <- w132
      }
    }
  }
  n475 = case shown="True" w3 {
    frame False {
    }
    frame True {
      # "close data files"
      n476 = local read "NF_Off_Ref"() -> (w608:refnum<file>)
      n477 = local read "NF_On_Ref"() -> (w609:refnum<file>)
      n478 = local read "FF_Off_Ref"() -> (w610:refnum<file>)
      n479 = local read "FF_On_Ref"() -> (w611:refnum<file>)
      n480 = local read "WS_On/Off"() -> (w607:bool)
      n481 = case shown="True" w607 {
        frame False {
        }
        frame True {
          n482 = local read "WS visa"() -> (w612:refnum<visa-resource-name>)
          n483 = call "T_RH_P.vi"("VISA in"=w612, "WS_Commands"=enum16{"OpenWS", "ReadTRHP", "CloseWS"}."CloseWS") -> ()  [unwired: 11 in, 3 out]
        }
      }
      n484 = Close File(refnum=w611) -> ()  [unwired: 1 in, 2 out]
      n485 = Close File(refnum=w610) -> ()  [unwired: 1 in, 2 out]
      n486 = Close File(refnum=w609) -> ()  [unwired: 1 in, 2 out]
      n487 = Close File(refnum=w608) -> ()  [unwired: 1 in, 2 out]
    }
  }
  "FileHour" <- -1 ("FileHour")
  "DataOpen" <- FALSE
